vi "tvac_gui_chamber.vi"() -> ()   [LabVIEW 2017]
uses:
  Zones.ctl
  <vilib>/httpClient/ClientHandle.ctl
  <vilib>/Utility/miscctls.llb/LVPositionTypeDef.ctl
  Type_Defs/Cryo_Pump_Plots.ctl
  <vilib>/Utility/error.llb/DialogType.ctl
  <vilib>/Utility/miscctls.llb/LVBoundsTypeDef.ctl
  msg7171_linux.llb/send single message.vi
  <vilib>/httpClient/POSTBuffer.vi
  <vilib>/Utility/file.llb/Read Delimited Spreadsheet (string).vi
  <vilib>/Utility/file.llb/Write Delimited Spreadsheet (string).vi
  <vilib>/httpClient/LabVIEWHTTPClient.lvlib
panel:
  out "Taskbar Status":T1 {"Chamber" format="%#_2g"; "Cryo" format="%#_2g"; "Roughing" format="%#_2g"}
  in  "importexe":dbl
  in  "Path to PNG file":path=path "C:/Users/stefan/Documents/GitHub/TVAC/head/Labview2017/TVAC_GUI/Visualization/chamber_test.png"
  in  "Moving 1":bool
  in  "TC1to45PicRef":refnum<vi>
  in  "profilearray":dbl[][](array[numeric])
  in  "LastSetPt":i32
  in  "string":string
  in  "tprofilesheet":string[][](array[string])
  in  "Custom Graph Selector":i32
  in  "exit":bool
  in  "AlarmColor":u32(colorbox)
  in  "Alarm String":string
  in  "Plot Color":u32(colorbox)=16860
  in  "Temperature":dbl format="%#_13g"
  in  "TC Label":string
  in  "Graph ON/OFF":u32(colorbox)=4250624
  in  "index (col)":i32
  in  "index (row)":i32
  out "working array":bool[](array[boolean])
  in  "Tab Control":T2(tab)
  in  "Log/Linear Y-Axis":u16(ring) items=["Linear", "Log"]
  in  "Total Time":dbl
  in  "Set Time TC Graph":bool
  in  "Graphing Selection":u16(ring) items=["User Selection", "Graph All Thermocouples", "Clear Graph"]
  in  "Time Scale":u16(ring) items=["Minutes", "Hours", "Seconds"]
  out "Waveform Chart":waveform(dbl)[](graph)
  out "Thermocouples":T3(array[cluster])
  in  "Log/Linear Y-Axis 6":u16(ring) items=["Linear", "Log"]
  in  "Log/Linear Y-Axis 5":u16(ring) items=["Linear", "Log"]
  in  "Log/Linear Y-Axis 3":u16(ring) items=["Linear", "Log"]
  in  "Log/Linear Y-Axis 2":u16(ring) items=["Linear", "Log"]
  in  "Total Time 6":dbl
  in  "Set Time TC Graph 6":bool
  in  "Time Scale 6":u16(ring) items=["Minutes", "Hours", "Seconds"]
  in  "Total Time 5":dbl
  in  "Set Time TC Graph 5":bool
  in  "Time Scale 5":u16(ring) items=["Minutes", "Hours", "Seconds"]
  in  "Total Time 4":dbl
  in  "Set Time TC Graph 4":bool
  in  "Time Scale 4":u16(ring) items=["Minutes", "Hours", "Seconds"]
  in  "Total Time 3":dbl
  in  "Set Time TC Graph 3":bool
  in  "Time Scale 3":u16(ring) items=["Minutes", "Hours", "Seconds"]
  in  "Total Time 2":dbl
  in  "Set Time TC Graph 2":bool
  in  "Time Scale 2":u16(ring) items=["Minutes", "Hours", "Seconds"]
  in  "Log/Linear Y-Axis 1":u16(ring) items=["Linear", "Log"]
  in  "Total Time 1":dbl
  in  "Set Time TC Graph 1":bool
  in  "Time Scale 1":u16(ring) items=["Minutes", "Hours", "Seconds"]
  in  "Custom Chart 2 Selection":i32[](listbox)=[0]
  in  "Custom Chart 1 Selection":i32[](listbox)=[0]
  out "Custom Chart 1":waveform(dbl)[](graph)
  in  "Custom Chart 3 Selection":i32[](listbox)=[0]
  in  "Custom Chart 4 Selection":i32[](listbox)=[0]
  in  "Custom Chart 5 Selection":i32[](listbox)=[0]
  in  "Custom Chart 6 Selection":i32[](listbox)=[0]
  out "Custom Chart 2":waveform(dbl)[](graph)
  out "Custom Chart 3":waveform(dbl)[](graph)
  out "Custom Chart 4":waveform(dbl)[](graph)
  out "Custom Chart 5":waveform(dbl)[](graph)
  out "Custom Chart 6":waveform(dbl)[](graph)
  in  "Log/Linear Y-Axis 4":u16(ring) items=["Linear", "Log"]
  in  "Initiate Vacuum State":bool
  in  "Complete Event List":i32(listbox)
  in  "Database Logging On/Off":bool
  out "Thermal Profile Compiling Summary":string
  out "Active Profile":bool
  out "ThermalProfileStatus":string
  out "Thermal Profile":cluster{dbl, dbl, "temp":dbl[][]}(graph)
  in  "Thermal Profile Loader":T4(tab)
  in  "ZoneSetup":T5={"Number of Set points"=0.0, "Zone Selection"=[8], "Initiate Setup"=FALSE, "Thermal Profile Name"="", "Saved Database Profiles"=0, "Import CSV as a Thermal Profile"=path "", "Import Profile"=FALSE, "LoadFromDatabase"=FALSE} {"Saved Database Profiles" items=["debug4", "debug4_2", "debug5", "debug5_1", "debug5_2", "debug5_3", "debug5_4", "debug5_5", "debug5_6", "debug6_1", "oct_26_1", "oct_26_4", "oct_26_5", "oct_26_fast_1", "oct_26_fast_2", "oct_26_fast_3", "Oct_27_1", "oct_27_2", "oct_27_3", "oct_27_4", "oct_27_5", "oct_27_full_test", "testing_oct24_1", "testing_oct24_2", "testing_oct24_debug1", "testing_oct_25_1"]}
  in  "RampSoakTimes":cluster{"RampSoakTimes":dbl[][]}
  in  "Zone 1":T6={"Zone Thermocouples"=[0], "Temperature Calculation"=0, "Thermocouples Selected"="", "Temperature Goal"=[], "Max Allowable Temp"="", "Min Allowable Temp"="", "Max Temp Slope"=""} {"Temperature Calculation" items=["Average", "Minimum", "Maximum"]}
  in  "Zone 2":T6={"Zone Thermocouples"=[0], "Temperature Calculation"=0, "Thermocouples Selected"="", "Temperature Goal"=[], "Max Allowable Temp"="", "Min Allowable Temp"="", "Max Temp Slope"=""} {"Temperature Calculation" items=["Average", "Minimum", "Maximum"]}
  in  "Zone 3":T6={"Zone Thermocouples"=[0], "Temperature Calculation"=0, "Thermocouples Selected"="", "Temperature Goal"=[], "Max Allowable Temp"="", "Min Allowable Temp"="", "Max Temp Slope"=""} {"Temperature Calculation" items=["Average", "Minimum", "Maximum"]}
  in  "Zone 4":T6={"Zone Thermocouples"=[0], "Temperature Calculation"=0, "Thermocouples Selected"="", "Temperature Goal"=[], "Max Allowable Temp"="", "Min Allowable Temp"="", "Max Temp Slope"=""} {"Temperature Calculation" items=["Average", "Minimum", "Maximum"]}
  in  "Zone 5":T6={"Zone Thermocouples"=[0], "Temperature Calculation"=0, "Thermocouples Selected"="", "Temperature Goal"=[], "Max Allowable Temp"="", "Min Allowable Temp"="", "Max Temp Slope"=""} {"Temperature Calculation" items=["Average", "Minimum", "Maximum"]}
  in  "Zone 6":T6={"Zone Thermocouples"=[0], "Temperature Calculation"=0, "Thermocouples Selected"="", "Temperature Goal"=[], "Max Allowable Temp"="", "Min Allowable Temp"="", "Max Temp Slope"=""} {"Temperature Calculation" items=["Average", "Minimum", "Maximum"]}
  in  "Zone 7":T6={"Zone Thermocouples"=[0], "Temperature Calculation"=0, "Thermocouples Selected"="", "Temperature Goal"=[], "Max Allowable Temp"="", "Min Allowable Temp"="", "Max Temp Slope"=""} {"Temperature Calculation" items=["Average", "Minimum", "Maximum"]}
  in  "Zone 8":T6={"Zone Thermocouples"=[0], "Temperature Calculation"=0, "Thermocouples Selected"="", "Temperature Goal"=[], "Max Allowable Temp"="", "Min Allowable Temp"="", "Max Temp Slope"=""} {"Temperature Calculation" items=["Average", "Minimum", "Maximum"]}
  in  "Zone 9":T6={"Zone Thermocouples"=[0], "Temperature Calculation"=0, "Thermocouples Selected"="", "Temperature Goal"=[], "Max Allowable Temp"="", "Min Allowable Temp"="", "Max Temp Slope"=""} {"Temperature Calculation" items=["Average", "Minimum", "Maximum"]}
  out "Current Profile Name":string
  in  "Delete Profile":bool
  in  "New File Name":string
  in  "Rename":bool
  in  "2. Save Into Database and CSV":bool
  in  "3. Load into Memory":bool
  in  "1. Compile Profile":bool
  in  "4. Run Profile":bool
  in  "Delete From Database":u16(ring) items=["Awesome Profile", "Super Awesome Profile", "Rocket Profile", "Bannana"]
  in  "HARD STOP":bool
  in  "Pause Profile":bool
  in  "Hold Profile":bool
  out "tpStatus":T7 {"Chamber" format="%#_2g"; "Cryo" format="%#_2g"; "Roughing" format="%#_2g"}
  out "generalStatus":T7 {"Chamber" format="%#_2g"; "Cryo" format="%#_2g"; "Roughing" format="%#_2g"}
  in  "Tab Control 2":enum32{"TCs 1-75", "TCs 76-80, 96-120"}(tab)
  out "TC1to75visual":T8={"1"=TRUE, "2"=TRUE, "3"=TRUE, "4"=TRUE, "5"=TRUE, "6"=TRUE, "7"=TRUE, "8"=TRUE, "9"=TRUE, "10"=TRUE, "11"=TRUE, "12"=TRUE, "13"=TRUE, "14"=TRUE, "15"=TRUE, "16"=TRUE, "17"=TRUE, "18"=TRUE, "19"=TRUE, "20"=TRUE, "21"=TRUE, "22"=TRUE, "23"=TRUE, "24"=TRUE, "25"=TRUE, "26"=TRUE, "27"=TRUE, "28"=TRUE, "29"=TRUE, "30"=TRUE, "31"=TRUE, "32"=TRUE, "33"=TRUE, "34"=TRUE, "35"=TRUE, "36"=TRUE, "37"=TRUE, "38"=TRUE, "39"=TRUE, "40"=TRUE, "41"=TRUE, "42"=TRUE, "43"=TRUE, "44"=TRUE, "45"=TRUE, "46"=TRUE, "47"=TRUE, "48"=TRUE, "49"=TRUE, "50"=TRUE, "51"=TRUE, "52"=TRUE, "53"=TRUE, "54"=TRUE, "55"=TRUE, "56"=TRUE, "57"=TRUE, "58"=TRUE, "59"=TRUE, "60"=TRUE, "61"=TRUE, "62"=TRUE, "63"=TRUE, "64"=TRUE, "65"=TRUE, "66"=TRUE, "67"=TRUE, "68"=TRUE, "69"=TRUE, "70"=TRUE, "71"=TRUE, "72"=TRUE, "73"=TRUE, "74"=TRUE, "75"=TRUE, "new picture"=bytes[0]}
  in  "Reset All TC Positions":bool
  in  "Import UUT":bool
  out "Chamber Layout":T9 {"TC 120" format="%#_5g"; "TC 119" format="%#_5g"; "TC 118" format="%#_5g"; "TC 117" format="%#_5g"; "TC 116" format="%#_5g"; "TC 115" format="%#_5g"; "TC 114" format="%#_5g"; "TC 113" format="%#_5g"; "TC 112" format="%#_5g"; "TC 111" format="%#_5g"; "TC 110" format="%#_5g"; "TC 109" format="%#_5g"; "TC 108" format="%#_5g"; "TC 107" format="%#_5g"; "TC 106" format="%#_5g"; "TC 105" format="%#_5g"; "TC 104" format="%#_5g"; "TC 103" format="%#_5g"; "TC 102" format="%#_5g"; "TC 101" format="%#_5g"; "TC 100" format="%#_5g"; "TC 99" format="%#_5g"; "TC 98" format="%#_5g"; "TC 97" format="%#_5g"; "TC 96" format="%#_5g"; "TC 80" format="%#_5g"; "TC 79" format="%#_5g"; "TC 78" format="%#_5g"; "TC 77" format="%#_5g"; "TC 76" format="%#_5g"}
  out "Chamber Layout Picture":picture
  in  "Events":enum32{"Current", "Past"}(tab)
  in  "Clear All Events":bool
  in  "Current Events (click to clear)":i32(listbox)
  in  "Export Events":bool
  in  "Event History":i32(listbox)
  in  "Errors":enum32{"Current", "Past"}(tab)
  in  "Current Errors (click to clear)":i32(listbox)
  in  "Clear All Errors":bool
  in  "Export Errors":bool
  in  "Error History":i32(listbox)
  in  "Engineering":string
  in  "GetEvent":bool=TRUE
  in  "TCs On":bool=TRUE
  in  "Pressure On":bool=TRUE
  in  "MCC On":bool=TRUE
  in  "ZoneTemps On":bool=TRUE
  in  "Compressor On":bool
  in  "GetError":bool=TRUE
  out "flushed msgs":T10(array[cluster])
  out "system log event":string
  in  "getTvacStatus":bool=TRUE
  in  "Local Debug":bool
  in  "TVAC Labview":bool=TRUE
  # "Hidden Controls"
  # "Active Thermal Profile Commands"
  # "Create a New Thermal Profile"
  # "Import CSV as a Thermal Profile"
  # "Run Saved Database Profile"
  # "Set Pt #"
  # "Ramp Time (min)"
  # "Soak Time (min)"
  # "Set Pt #"
  # "Goal Temp (K)"
  # "Set Pt #"
  # "Goal Temp (K)"
  # "Set Pt #"
  # "Goal Temp (K)"
  # "Set Pt #"
  # "Goal Temp (K)"
  # "Set Pt #"
  # "Goal Temp (K)"
  # "Set Pt #"
  # "Goal Temp (K)"
  # "Set Pt #"
  # "Goal Temp (K)"
  # "Set Pt #"
  # "Goal Temp (K)"
  # "Set Pt #"
  # "Goal Temp (K)"
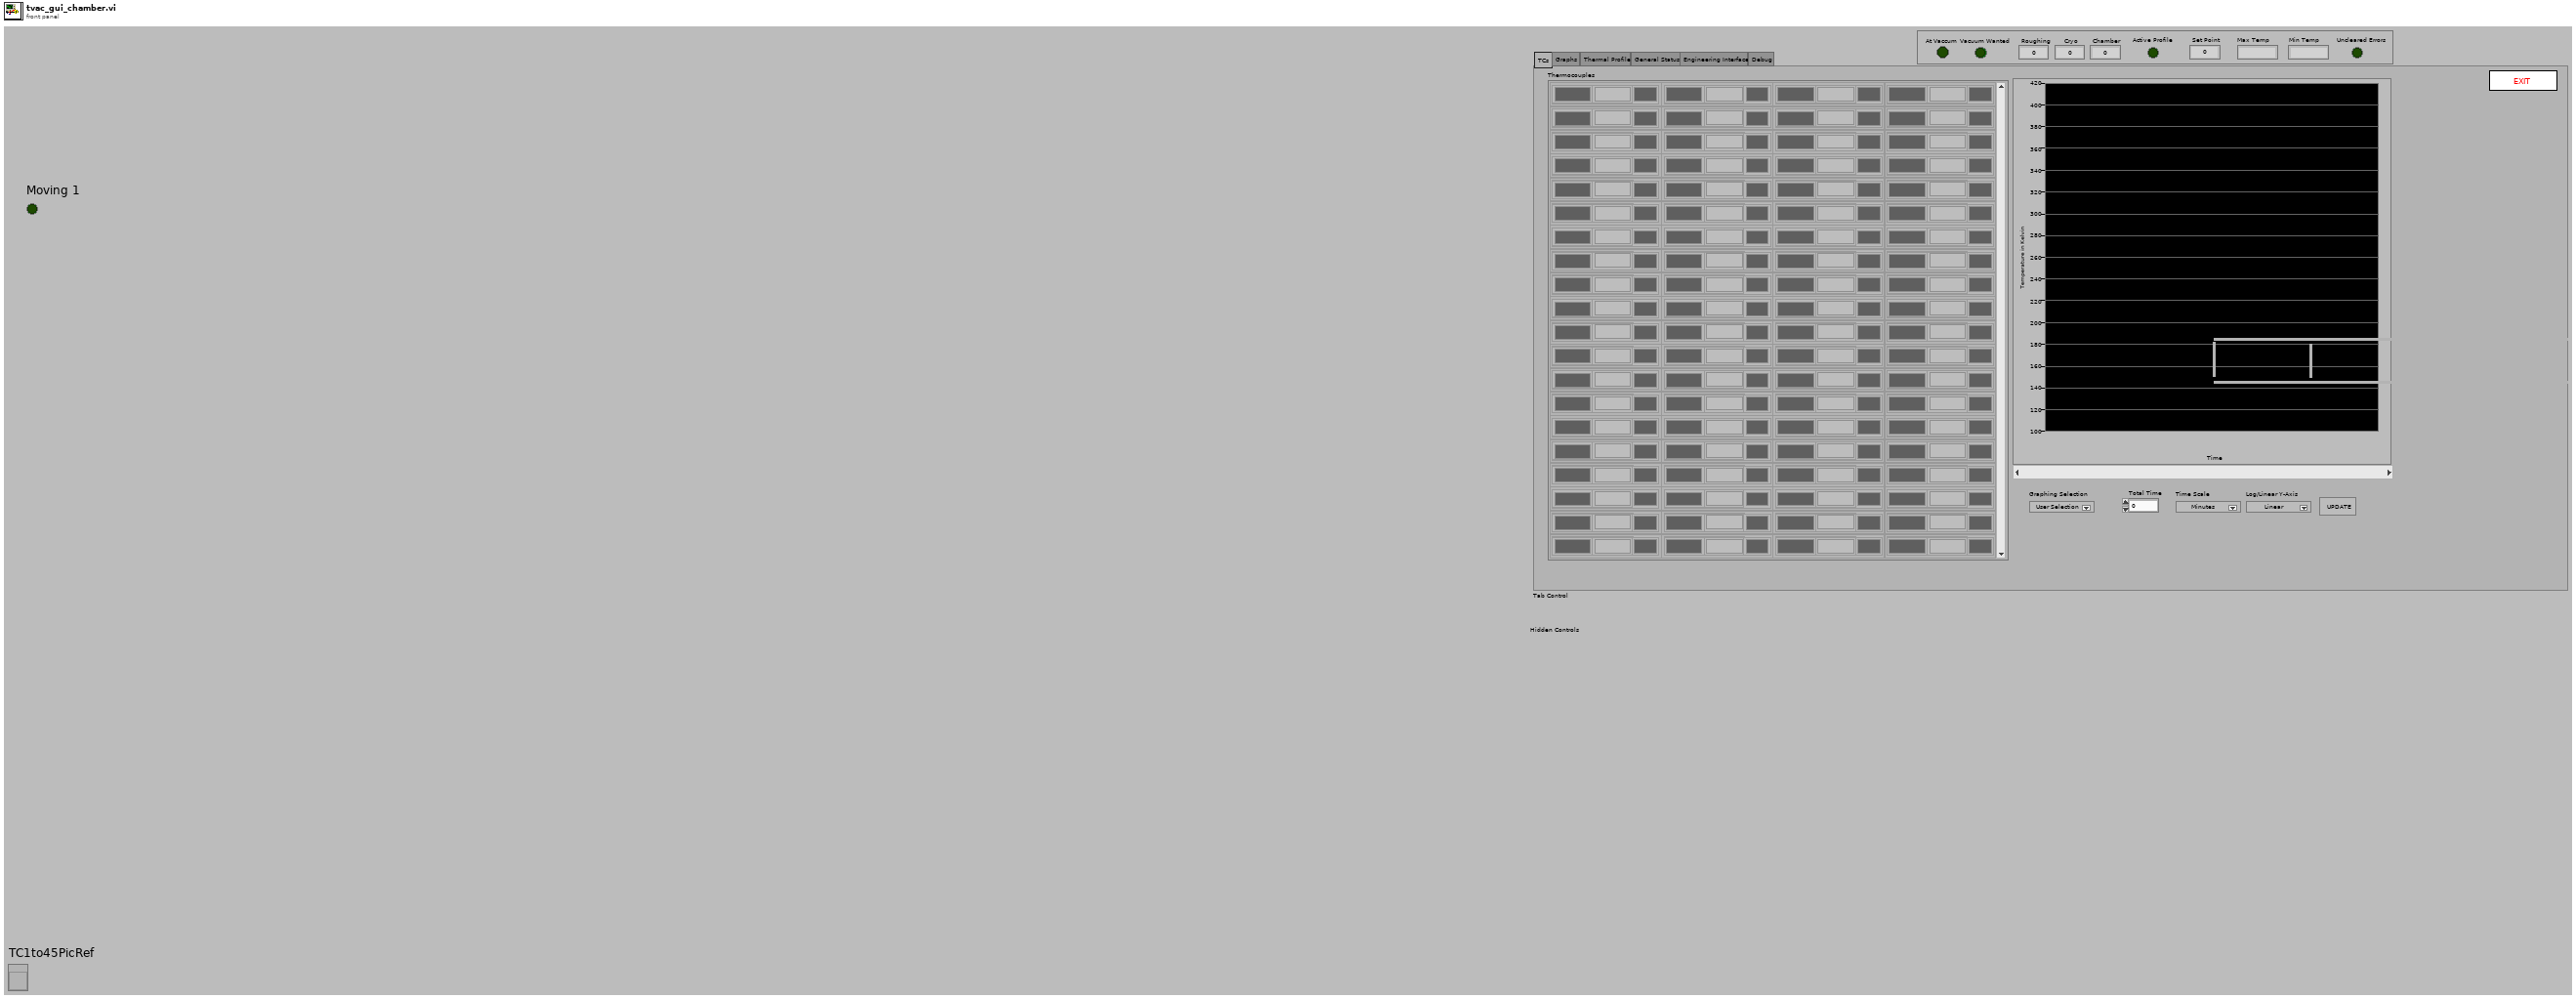
[diagram p1: front panel]
types:
  T1 = cluster{"At Vaccum":bool, "Vacuum Wanted":bool, "Roughing":dbl, "Cryo":dbl, "Chamber":dbl, "Active Profile":bool, "Set Point":dbl, "Max Temp":string, "Min Temp":string, "Uncleared Errors":bool}
  T2 = enum32{"TCs", "Graphs", "Thermal Profile", "General Status", "Engineering Interface", "Debug"}
  T3 = cluster{"TC Label":string, "Alarm Status":string, "Alarm Color":u32, "Temperature":string, "PlotColor":u32, "Graph On/Off":u32}[][]
  T4 = enum32{"Setup", "Set Point Timing", "Zone 1", "Zone 2", "Zone 3", "Zone 4", "Zone 5", "Zone 6", "Zone 7", "Zone 8", "Zone 9", "Run"}
  T5 = cluster{"Number of Set points":dbl, "Zone Selection":i32[], "Initiate Setup":bool, "Thermal Profile Name":string, "Saved Database Profiles":u16, "Import CSV as a Thermal Profile":path, "Import Profile":bool, "LoadFromDatabase":bool}
  T6 = typedef "Zones.ctl" = cluster{"Zone Thermocouples":i32[], "Temperature Calculation":u16, "Thermocouples Selected":string, "Temperature Goal":dbl[][], "Max Allowable Temp":string, "Min Allowable Temp":string, "Max Temp Slope":string}
  T7 = cluster{"Set Point":dbl, "Vacuum Wanted":bool, "Profile State":string, "Active Profile":bool, "Roughing":dbl, "Cryo":dbl, "Chamber":dbl, "Current Ramp/Soak Time":dbl, "Zone Temps":dbl[], "Remaining Ramp/Soak Time":dbl, "Max Ramp Rate":dbl, "Vacuum State":string, "At Vaccum":bool}
  T8 = cluster{"1":bool, "2":bool, "3":bool, "4":bool, "5":bool, "6":bool, "7":bool, "8":bool, "9":bool, "10":bool, "11":bool, "12":bool, "13":bool, "14":bool, "15":bool, "16":bool, "17":bool, "18":bool, "19":bool, "20":bool, "21":bool, "22":bool, "23":bool, "24":bool, "25":bool, "26":bool, "27":bool, "28":bool, "29":bool, "30":bool, "31":bool, "32":bool, "33":bool, "34":bool, "35":bool, "36":bool, "37":bool, "38":bool, "39":bool, "40":bool, "41":bool, "42":bool, "43":bool, "44":bool, "45":bool, "46":bool, "47":bool, "48":bool, "49":bool, "50":bool, "51":bool, "52":bool, "53":bool, "54":bool, "55":bool, "56":bool, "57":bool, "58":bool, "59":bool, "60":bool, "61":bool, "62":bool, "63":bool, "64":bool, "65":bool, "66":bool, "67":bool, "68":bool, "69":bool, "70":bool, "71":bool, "72":bool, "73":bool, "74":bool, "75":bool, "new picture":picture}
  T9 = cluster{"TC 76":dbl, "TC 77":dbl, "TC 78":dbl, "TC 79":dbl, "TC 80":dbl, "TC 96":dbl, "TC 97":dbl, "TC 98":dbl, "TC 99":dbl, "TC 100":dbl, "TC 101":dbl, "TC 102":dbl, "TC 103":dbl, "TC 104":dbl, "TC 105":dbl, "TC 106":dbl, "TC 107":dbl, "TC 108":dbl, "TC 109":dbl, "TC 110":dbl, "TC 111":dbl, "TC 112":dbl, "TC 113":dbl, "TC 114":dbl, "TC 115":dbl, "TC 116":dbl, "TC 117":dbl, "TC 118":dbl, "TC 119":dbl, "TC 120":dbl}
  T10 = cluster{"source":string, "event":string, "event buffer":string}[]
  T11 = typedef "LVPositionTypeDef.ctl" = cluster{"Left":i32, "Top":i32}
  T12 = cluster{"recordData":bool, "currentSetpoint":i32, "vacuumWanted":bool, "inPause":bool, "activeProfile":bool, "inRamp":bool, "inHold":bool, "CryoPressure":dbl, "ChamberPressure":dbl, "RoughingPressure":dbl, "OperationalVacuum":bool}
  T13 = cluster{"profiles":cluster{"zone":i32, "average":string, "thermocouples":i32[], "maxTemp":i32, "minTemp":i32, "maxSlope":dbl, "thermalprofiles":cluster{"thermalsetpoint":i32, "tempgoal":i32, "ramp":i32, "soakduration":i32}[]}[]}
  T14 = cluster{"thermocouple":i32, "time":dbl, "temp":dbl, "working":bool, "alarm":i32}[]
  T15 = cluster{"Cp Stage 1 Temp":dbl[], "Cp Stage 2 Temp":dbl[]}
  T16 = typedef "LabVIEWHTTPClient.lvlib/ClientHandle.ctl" = refnum<k1>
  T17 = cluster{"ZoneSetup":cluster{"Number of Set points":dbl, "Zone Selection":i32[], "Initiate Setup":bool, "Thermal Profile Name":string, "Saved Database Profiles":u16, "Import CSV as a Thermal Profile":path, "Import Profile":bool, "LoadFromDatabase":bool}, "go":bool, "Http session":T16, "URL prefex":string, "index (row)":i32, "index (col)":i32, "Graph ON/OFF":u32, "TC Label":string, "Temperature":dbl, "AlarmColor":u32, "Plot Color":u32, "Alarm String":string, "Thermocouples":cluster{"TC Label":string, "Alarm Status":string, "Alarm Color":u32, "Temperature":string, "PlotColor":u32, "Graph On/Off":u32}[][], "working array":bool[], "i":i32, "NumberTCs":i32, "Waveform Chart":waveform(dbl)[], "Custom Chart 1":waveform(dbl)[], "Pressure":dbl[], "numSensors":i32, "Database":dbl[], "PumpTemps":cluster{"Cp Stage 1 Temp":dbl[], "Cp Stage 2 Temp":dbl[]}, "Zones":dbl[], "Time":i32, "TCs":cluster{"thermocouple":i32, "time":dbl, "temp":dbl, "working":bool, "alarm":i32}[], "ZoneTemps":cluster{"ZoneTemps":dbl[]}, "Compressor":cluster{"CompressorTemp":dbl}, "ErrorArray":string[][], "PrevErrorArray":string[][], "MasterErrorArray":string[][], "tprofilesheet":string[][], "Zone 1":T6, "ZoneProfile":cluster{"profiles":cluster{"zone":i32, "average":string, "thermocouples":i32[], "maxTemp":i32, "minTemp":i32, "maxSlope":dbl, "thermalprofiles":cluster{"thermalsetpoint":i32, "tempgoal":i32, "ramp":i32, "soakduration":i32}[]}[]}, "ZonesSelected":bool[], "Zone 2":T6, "Zone 3":T6, "Zone 4":T6, "Zone 5":T6, "Zone 6":T6, "Zone 7":T6, "Zone 8":T6, "Zone 9":T6, "MasterEventArray":string[][], "PrevEventArray":string[][], "EventArray":string[][], "TC1to45PicRef":refnum<vi>, "TvacStatus":cluster{"recordData":bool, "currentSetpoint":i32, "vacuumWanted":bool, "inPause":bool, "activeProfile":bool, "inRamp":bool, "inHold":bool, "CryoPressure":dbl, "ChamberPressure":dbl, "RoughingPressure":dbl, "OperationalVacuum":bool}}
  T18 = cluster{"TC Label":string, "Alarm Status":string, "Alarm Color":u32, "Temperature":string, "PlotColor":u32, "Graph On/Off":u32}
  T19 = cluster{"time":string, "TCs":cluster{"thermocouple":i32, "time":dbl, "temp":dbl, "working":bool, "alarm":i32}[]}
  T20 = cluster{"name":string, "profiles":cluster{"zone":i32, "average":string, "thermocouples":i32[], "maxTemp":i32, "minTemp":i32, "maxSlope":i32, "thermalprofiles":cluster{"thermalsetpoint":i32, "tempgoal":i32, "ramp":i32, "soakduration":i32}[]}[]}
  T21 = enum16{"open", "replace", "create", "open or create", "replace or create", "replace or create with confirmation"}
  T22 = cluster{"zone":i32, "average":string, "thermocouples":i32[], "maxTemp":i32, "minTemp":i32, "maxSlope":dbl, "thermalprofiles":cluster{"thermalsetpoint":i32, "tempgoal":i32, "ramp":i32, "soakduration":i32}[]}
  T23 = cluster{"thermalsetpoint":i32, "tempgoal":i32, "ramp":i32, "soakduration":i32}
  T24 = cluster{"time":string[], "event":string[], "item":string[], "itemID":i32[], "details":string[], "actions":string[][]}
  T25 = enum32{"TCs", "Graphs", "Thermal Profile", "General Status"}
  T26 = cluster{"time":string[], "category":string[], "message":string[]}
  T27 = cluster{"CryoPressure":dbl, "ChamberPressure":dbl, "RoughingPressure":dbl}
  T28 = cluster{"Set Point":dbl, "Vacuum Wanted":bool, "Profile State":string, "Active Profile":bool, "Roughing":dbl, "Cryo":dbl, "Chamber":dbl, "Current Ramp/Soak Time":dbl, "Zone Temps":dbl[], "Remaining Ramp/Soak Time":dbl, "Max Ramp Rate":dbl, "Vacuum State":string, "At Vacuum":bool}
  T29 = typedef "imagedata.ctl" = cluster{"image type":i32, "image depth":i32, "image":u8[], "mask":u8[], "colors":u32[], "Rectangle":cluster{"left":i16, "top":i16, "right":i16, "bottom":i16}}
  T30 = typedef "LVPoint32TypeDef.ctl" = cluster{"Horizontal":i32, "Vertical":i32}
  T31 = typedef "LVRangeTypeDef.ctl" = cluster{"Minimum":dbl, "Maximum":dbl, "Increment":dbl, "Minor Increment":dbl, "Start":dbl}
  T32 = cluster{"zone":i32, "average":string, "thermocouples":i32[], "maxTemp":i32, "minTemp":i32, "maxSlope":dbl, "thermalprofiles":cluster{"thermalsetpoint":i32, "tempgoal":i32, "ramp":i32, "soakduration":i32}[]}[]
  T33 = typedef "LVRowAndColumnTypeDef.ctl" = cluster{"Row":i32, "Column":i32}
  T34 = cluster{"thermalsetpoint":i32, "tempgoal":i32, "ramp":i32, "soakduration":i32}[]
  T35 = cluster{"time":dbl[], "zone1":dbl[], "zone2":dbl[], "zone3":dbl[], "zone4":dbl[], "zone5":dbl[], "zone6":dbl[], "zone7":dbl[], "zone8":dbl[], "zone9":dbl[]}
  T36 = typedef "Cryo_Pump_Plots.ctl" = cluster{"Duty Cycle (0-100)":dbl, "1st stage Temp (K)":dbl, "2st stage Temp (K)":dbl, "Helium Return Pressure (psig)":u32, "Helium Discharge Temp (C)":u32, "Water Inlet Temp (C)":u32, "Water Outlet Temp (C)":u32}
  T37 = typedef "DialogType.ctl" = u16
  T38 = cluster{"thermocouple":i32, "time":dbl, "temp":dbl, "working":bool, "alarm":i32}
  T39 = cluster{"[0]":dbl, "[1]":dbl, "[2]":dbl, "[3]":dbl, "[4]":dbl, "[5]":dbl, "[6]":dbl, "[7]":dbl, "[8]":dbl, "[9]":dbl, "[10]":dbl, "[11]":dbl, "[12]":dbl, "[13]":dbl, "[14]":dbl, "[15]":dbl, "[16]":dbl, "[17]":dbl, "[18]":dbl, "[19]":dbl, "[20]":dbl, "[21]":dbl, "[22]":dbl, "[23]":dbl, "[24]":dbl, "[25]":dbl, "[26]":dbl, "[27]":dbl, "[28]":dbl, "[29]":dbl}
  T40 = typedef "LVBoundsTypeDef.ctl" = cluster{"Width":u32, "Height":u32}
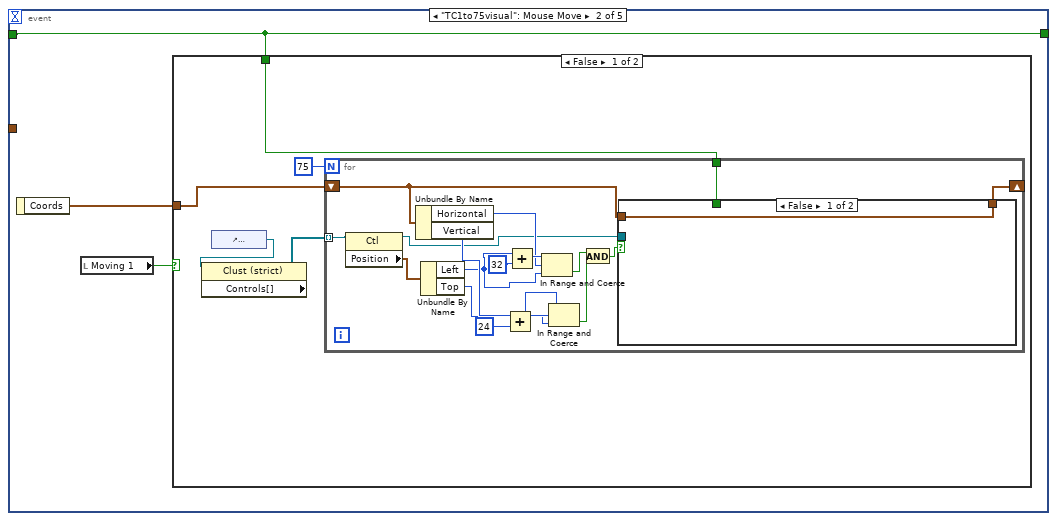
[diagram p3: hidden frame]
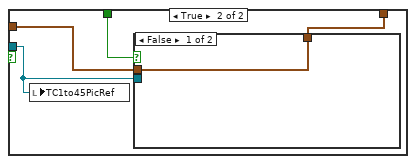
[diagram p4: hidden frame]
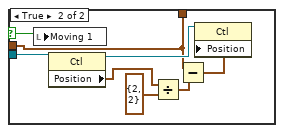
[diagram p5: hidden frame]
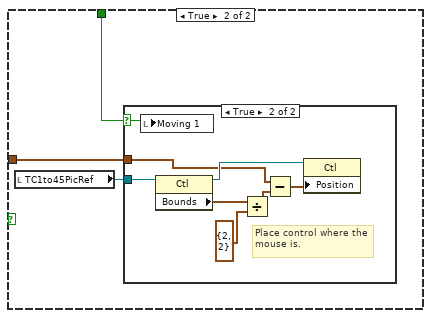
[diagram p6: hidden frame]
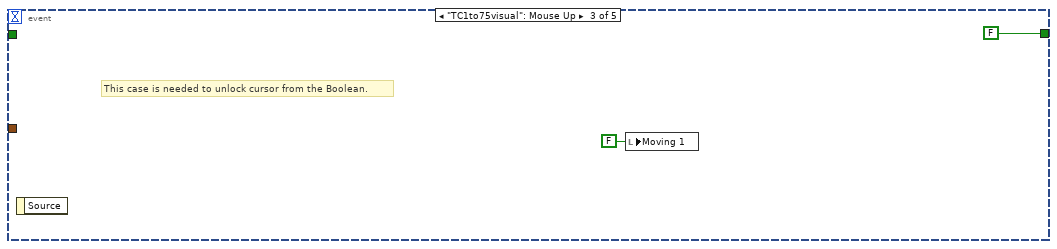
[diagram p8: hidden frame]
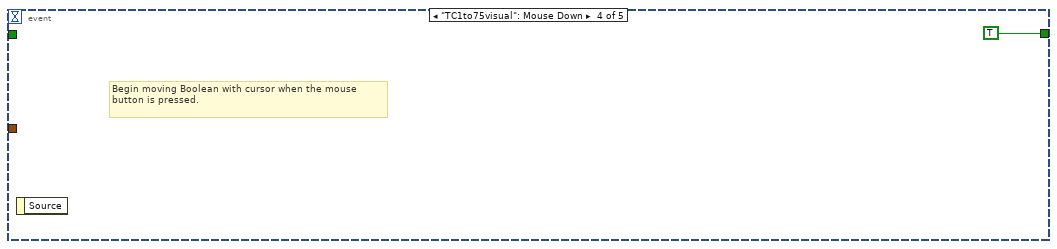
[diagram p9: hidden frame]
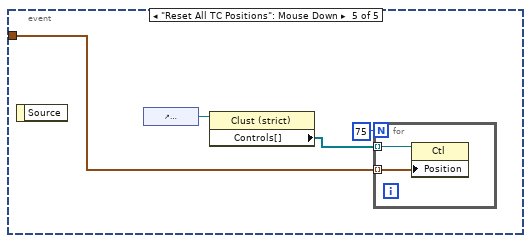
[diagram p10: hidden frame]
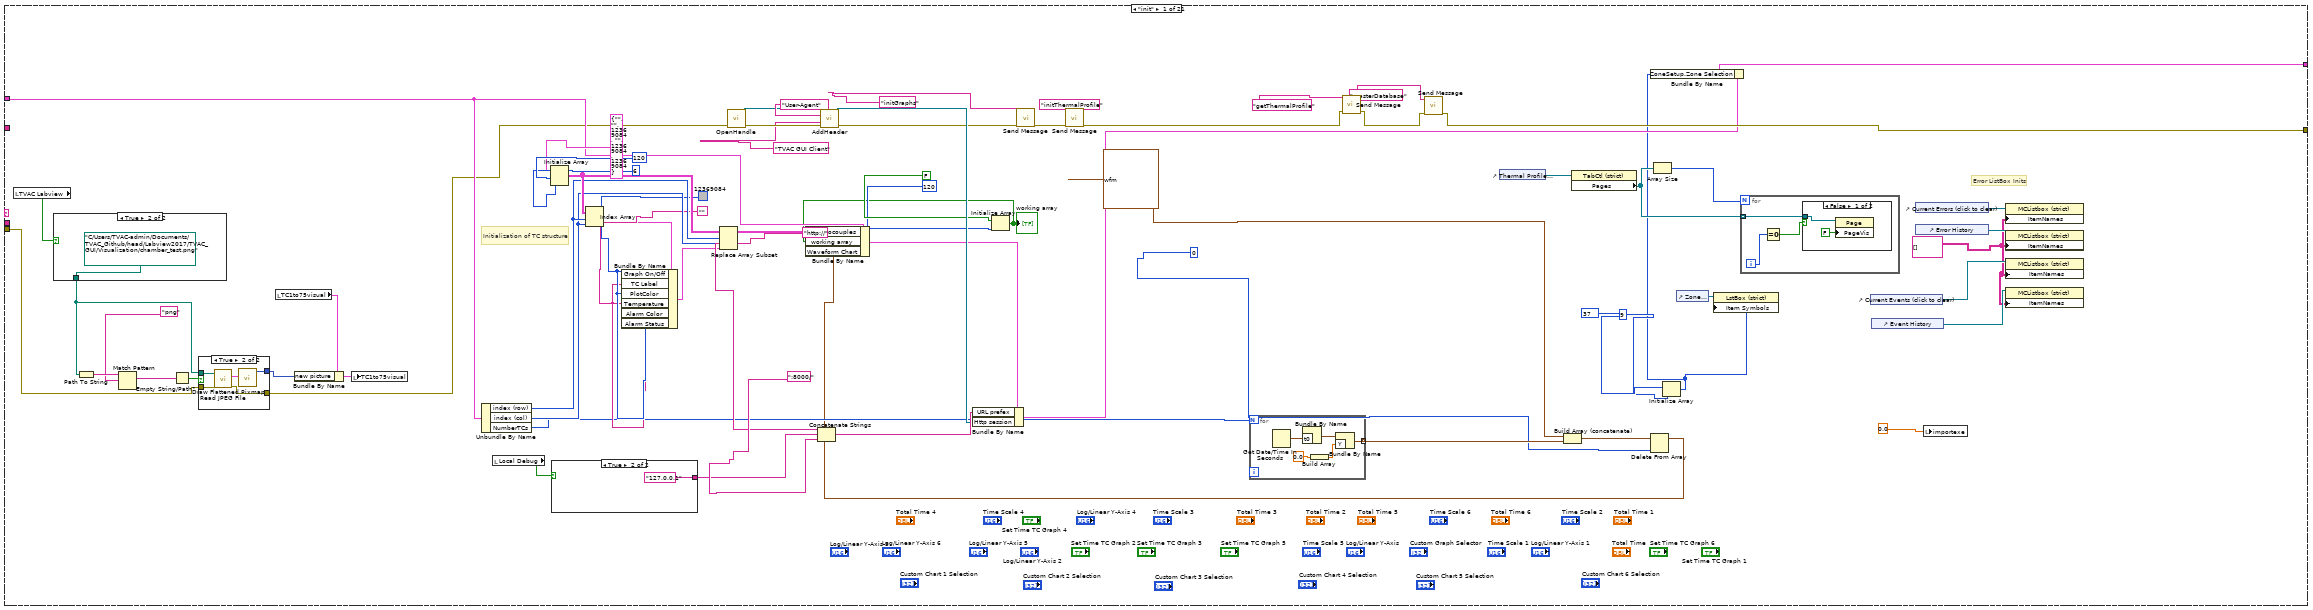
[diagram p11: hidden frame]
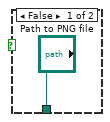
[diagram p12: hidden frame]
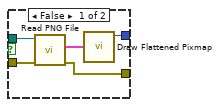
[diagram p13: hidden frame]
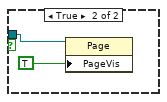
[diagram p14: hidden frame]
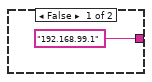
[diagram p15: hidden frame]
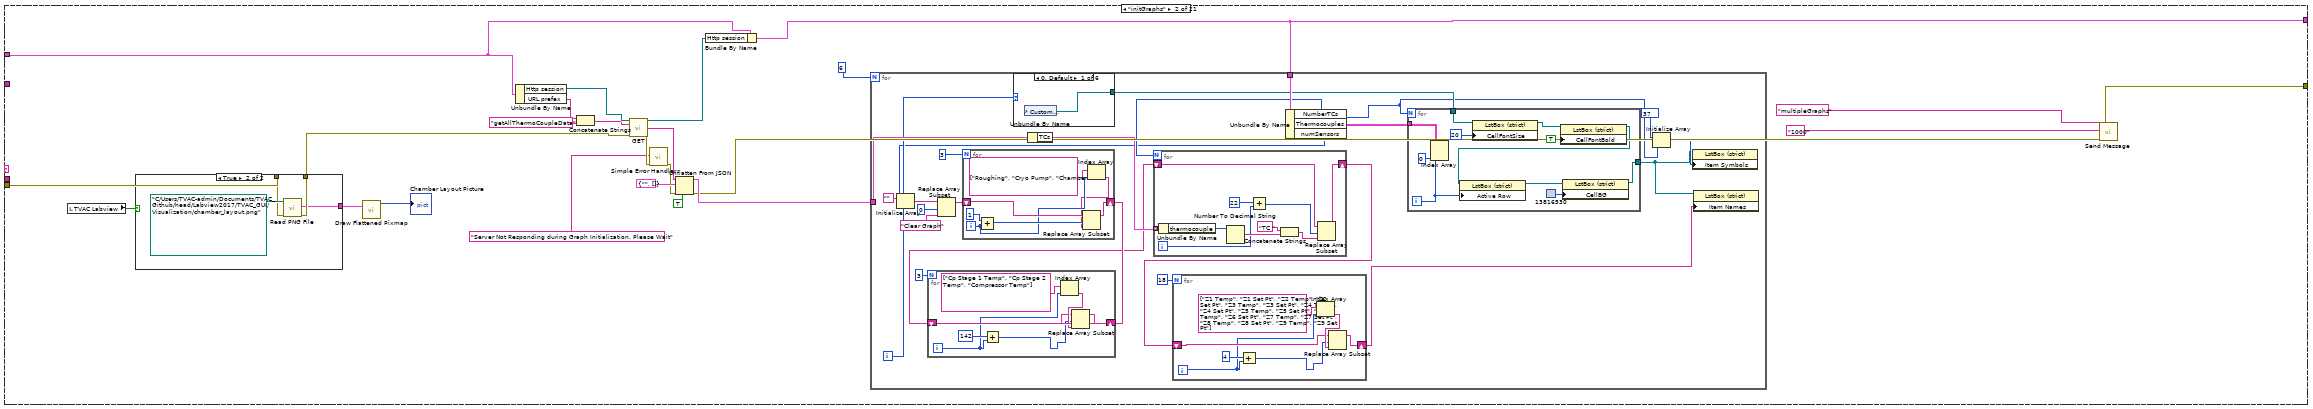
[diagram p16: hidden frame]
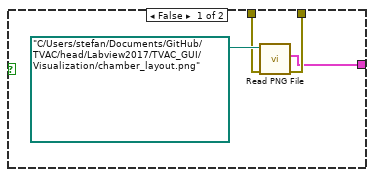
[diagram p17: hidden frame]
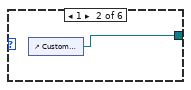
[diagram p18: hidden frame]
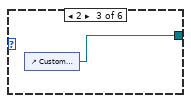
[diagram p19: hidden frame]
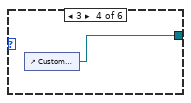
[diagram p20: hidden frame]
diagram:
  w5 = T12 {"recordData"=FALSE, "currentSetpoint"=0, "vacuumWanted"=FALSE, "inPause"=FALSE, "activeProfile"=FALSE, "inRamp"=FALSE, "inHold"=FALSE, "CryoPressure"=0.0, "ChamberPressure"=0.0, "RoughingPressure"=0.0, "OperationalVacuum"=FALSE}  # TvacStatus
  w9 = string[][] []  # MasterEventArray
  w7 = string[][] []  # EventArray
  w8 = string[][] []  # PrevEventArray
  w10 = string[][] []  # MasterErrorArray
  w14 = T13 {"profiles"=[]}  # ZoneProfile
  w23 = bool[] [FALSE, FALSE, FALSE, FALSE, FALSE, FALSE, FALSE, FALSE, FALSE]  # ZonesSelected
  w27 = string[][] []  # PrevErrorArray
  w28 = string[][] []  # ErrorArray
  w31 = cluster{"ZoneTemps":dbl[]} {"ZoneTemps"=[]}  # ZoneTemps
  w34 = dbl[] [24.54828257301887, 25.0, 20.035959453954195, 26.0, 28.926820041278148, 27.0, 21.321976066931608, 28.0, 29.197600688359813, 29.0, 29.117373424110085, 30.0, 21.092914485312942, 31.0, 27.791581465649088, 32.0, 24.70861457288988, 33.0]  # Zones
  w35 = T15 {"Cp Stage 1 Temp"=[0.0], "Cp Stage 2 Temp"=[0.0]}  # PumpTemps
  w36 = dbl[] [0.0, 1000.5841582194602, 1000.5841582194602, 1000.5841582194602, 0.6389895835935778, 0.7578061575842531, 1.153531014677555, 1.4572061556343079, 1.0192558642672256, 0.9245021790184325, 0.34311035179988925, 1.1970333160202968, 1.066989851322369, 0.5926593131154867, 0.7219240511326698, 1.0529790116491695, 1.4485694746891444, 0.9139060201605569, 0.7997359753068659, 0.6568795179977746, 0.8470104541419833, 1.0272585161866683, 0.6577301535824354, 0.645139941938139, 1.5235316442408067, 0.5128651184775285, 1.6421980587090137, 1.3961508335147417, 1.1242639015795428, 1.5954313466624428, 1.1919135255187876, 1.2615004458206727, 1.1320092264321664, 1.922759836270222, 1.1315561200367314, 1.4924621723754858, 0.6988771274186227, 1.069709701591943, 0.9920698240997152, 0.5395549253287656, 0.42891479657680576, 1.2794224940227927, 0.2687949632437338, 0.16127136772755854, 1.0174597006256374, 1.2079238230365172, 0.9745554383837218, 1.5348516925460962, 0.9488878852839246, 1.6634477658652282, 1.1924291951744272, 1.2231949298067308, 1.2223766746774598, 1.30664154589907, 1.2872878364107239, 0.5274250065177812, 0.7905999067114673, 1.2748974665085449, 1.216972941585413, 0.959115576325391, 0.5743502840762814, 0.8219540421676025, 0.613053899308251, 1.3785560870413707, 1.034117232127813, 1.1237698659753859, 1.4495548642149667, 0.6967905980938514, 0.6224497255665377, 1.6551326273040576, 1.2103048396824558, 0.6078721016951973, 1.3790669246280296, 0.5454332940871525, 1.5318777012492035, 1.2496539590411258, 0.9145395304446965, 1.3855381787793546, 1.0857600342029163, 1.3185833631438346, 0.9769688683142593, 1.026663691242448, 0.6744610422623843, 1.1965175398567691, 0.4847084945450119, 0.6435799980029115, 0.8079659363810663, 0.9130053929540112, 0.5271098423006861, 0.8088111736464799, 1.1455315536576556, 1.139809531926708, 1.5840192673434794, 1.0296748968089129, 1.7370669751200136, 1.3715484550405317, 0.3362063953932494, 1.0385868418202253, 1.4947740276021626, 1.0393600693910505, 0.8870410800672984, 1.2470388696569872, 0.9846724980375481, 0.9952471377109308, 1.0807485178906029, 1.1016630607035562, 1.3301039036808464, 0.8856852816151205, 0.4719509873120426, 0.5191430277856135, 0.12135113366044793, 0.4230478635224125, 1.1140562049976255, 1.5484968368781251, 1.1999891199114734, 1.8721302183420216, 1.071489235222563, 0.6260864330445979, 1.0305668002030492, 1.0223711899566386, 0.7842533472819472, 1.7301290335750898, 1.318694748426881, 0.6978662965493679]  # Database
  w38 = dbl[] [0.0, 0.0, 0.0]  # Pressure
  w57 = ""  # URL prefex
  w58 = T16 refnum  # Http session
  w59 = TRUE  # go
  n1 = call "Register Module.vi"() -> ("error out"=w55:errorcluster)  [unwired: 10 in, 1 out]
  n2 = call-poly "Send Message.vi"("error in (no error)"=w55, "event"="init") -> ("error out"=w54:errorcluster)  [unwired: 9 in]
  n3 = local read "Waveform Chart"() -> (w41:waveform(dbl)[])
  n4 = local read "Thermocouples"() -> (w40:T3)
  n5 = local read "Custom Chart 1"() -> (w39:waveform(dbl)[])
  n6 = Bundle("ZoneSetup"="ZoneSetup", "go"=w59, "Http session"=w58, "URL prefex"=w57, "index (row)"="index (row)", "index (col)"="index (col)", "Graph ON/OFF"="Graph ON/OFF", "TC Label"="TC Label", "Temperature"="Temperature", "AlarmColor"="AlarmColor", "Plot Color"="Plot Color", "Alarm String"="Alarm String", "Thermocouples"=w40, "working array"=bool[] [TRUE, TRUE, TRUE, TRUE, TRUE, TRUE, TRUE, TRUE, TRUE, TRUE, TRUE, TRUE, TRUE, TRUE, TRUE, TRUE, TRUE, TRUE, TRUE, TRUE, TRUE, TRUE, TRUE, TRUE, TRUE, TRUE, TRUE, TRUE, TRUE, TRUE, TRUE, TRUE, TRUE, TRUE, TRUE, TRUE, TRUE, TRUE, TRUE, TRUE, TRUE, TRUE, TRUE, TRUE, TRUE, TRUE, TRUE, TRUE, TRUE, TRUE, TRUE, TRUE, TRUE, TRUE, TRUE, TRUE, TRUE, TRUE, TRUE, TRUE, TRUE, TRUE, TRUE, TRUE, TRUE, TRUE, TRUE, TRUE, TRUE, TRUE, TRUE, TRUE, TRUE, TRUE, TRUE, TRUE, TRUE, TRUE, TRUE, TRUE, TRUE, TRUE, TRUE, TRUE, TRUE, TRUE, TRUE, TRUE, TRUE, TRUE, TRUE, TRUE, TRUE, TRUE, TRUE, TRUE, TRUE, TRUE, TRUE, TRUE, TRUE, TRUE, TRUE, TRUE, TRUE, TRUE, TRUE, TRUE, TRUE, TRUE, TRUE, TRUE, TRUE, TRUE, TRUE, TRUE, TRUE, TRUE, TRUE, TRUE], "i"=0, "NumberTCs"=120, "Waveform Chart"=w41, "Custom Chart 1"=w39, "Pressure"=w38, "numSensors"=145, "Database"=w36, "PumpTemps"=w35, "Zones"=w34, "Time"=0, "TCs"=T14 [], "ZoneTemps"=w31, "Compressor"=cluster{"CompressorTemp":dbl} {"CompressorTemp"=0.0}, "ErrorArray"=w28, "PrevErrorArray"=w27, "MasterErrorArray"=w10, "tprofilesheet"="tprofilesheet", "Zone 1"="Zone 1", "ZoneProfile"=w14, "ZonesSelected"=w23, "Zone 2"="Zone 2", "Zone 3"="Zone 3", "Zone 4"="Zone 4", "Zone 5"="Zone 5", "Zone 6"="Zone 6", "Zone 7"="Zone 7", "Zone 8"="Zone 8", "Zone 9"="Zone 9", "MasterEventArray"=w9, "PrevEventArray"=w8, "EventArray"=w7, "TC1to45PicRef"="TC1to45PicRef", "TvacStatus"=w5) -> (w45:T17)  [unwired: 1 in]
  n7 = invoke on="exit" class="Bool (strict)" method="Reinit To Default"() -> ()  [unwired: 3 in, 3 out]
  n8 = while {
    shift-left: w45 -> [w66]
    shift-right: [w64] -> _
    shift-right: [w65] -> w13
    shift-left: w54 -> [w70]
    stop <- w63 continue-if-true
    n9 = call "Get Message.vi"("error in (no error)"=w70) -> ("error out"=w69:errorcluster, "event buffer"=w61:string, "event"=w68:string, "source"=w67:string)  [unwired: 7 in]
    n10 = case shown="\"receiveCryoPump_plots\"" w68 {
      selector: w68 -> [_ _ _ _ _ _ _ _ _ _ _ _ _ _ _ _ _ _ _ _ w3925]
      tunnel: [w88 w170 w271 w377 w2380 w2704 w3217 w3332 w3414 w3420 w3434 w3457 w3552 w3614 w3626 w3674 w3740 w3753 w3773 w3923 w3927] -> w64
      tunnel: w66 -> [w113 w171 w272 w379 w2431 w2695 w3231 w3337 w3413 w3420 w3433 w3451 w3546 w3615 w3631 w3699 w3739 w3754 w3773 w3919 w3927]
      tunnel: w61 -> [_ _ _ _ w2393 _ _ _ w3411 w3418 w3426 w3458 w3553 w3606 w3630 w3704 w3737 _ w3774 _ _]
      tunnel: w69 -> [w75 w176 w280 w381 w2376 w2703 w3233 w3327 w3412 w3421 w3427 w3455 w3550 w3607 w3629 w3703 w3738 w3759 _ w3922 w3926]
      tunnel: [w98 w179 w277 w380 w2409 w2701 w3233 w3327 w3412 w3421 w3427 w3455 w3550 w3607 w3629 w3703 w3738 w3759 _ w3921 w3924] -> w60
      tunnel: w67 -> [_ _ _ _ _ _ _ _ _ _ _ _ _ _ _ _ _ _ _ _ _]
      frame "init" {
        w83 = string[][] [] ("Item Names")
        w118 = ""
        w119 = u32 12369084 ("PlotColor")
        # "Error ListBox Inits"
        # "Initialization of TC structure"
        n11 = local read "TVAC Labview"() -> (w71:bool)
        n12 = case shown="True" w71 {
          tunnel: ["Path to PNG file" path "C:/Users/TVAC-admin/Documents/TVAC_Github/head/Labview2017/TVAC_GUI/Visualization/chamber_test.png" ("Path to PNG file")] -> w76
          frame False {
          }
          frame True {
          }
        }
        n13 = Path To String(path=w76) -> (string=w80:string)
        n14 = Match Pattern(string=w80, regular expression="png") -> (match substring=w78:string)  [unwired: 1 in, 3 out]
        n15 = Empty String/Path?(string/path=w78) -> (empty?=w77:bool)
        n16 = case shown="True" w77 {
          tunnel: [w144 w149] -> w73
          tunnel: w75 -> [w143 w146]
          tunnel: [w142 w147] -> w74
          tunnel: w76 -> [w140 w145]
          frame False {
            n17 = call <vilib>:"Read PNG File.vi"("error in (no error)"=w143, "path to PNG file"=w140) -> ("error out"=w142:errorcluster, "image data"=w141:T29)  [unwired: 7 in, 1 out]
            n18 = call <vilib>:"Draw Flattened Pixmap.vi"("image data"=w141) -> ("new picture"=w144:picture)  [unwired: 8 in]
          }
          frame True {
            n19 = call <vilib>:"Read JPEG File.vi"("error in (no error)"=w146, "path to JPEG file"=w145) -> ("error out"=w147:errorcluster, "image data"=w148:T29)  [unwired: 7 in, 1 out]
            n20 = call <vilib>:"Draw Flattened Pixmap.vi"("image data"=w148) -> ("new picture"=w149:picture)  [unwired: 8 in]
          }
        }
        n21 = local read "TC1to75visual"() -> (w81:T8)
        n22 = Bundle By Name(cluster=w81, "new picture"=w73) -> (w82:T8)
        n23 = local write "TC1to75visual"(w82) -> ()
        n24 = Unbundle By Name(w113) -> ("index (row)"=w121:i32, "index (col)"=w120:i32, "NumberTCs"=w110:i32)
        n25 = local read "Local Debug"() -> (w126:bool)
        n26 = Initialize Array(T18 {"TC Label"="", "Alarm Status"="", "Alarm Color"=12369084, "Temperature"="", "PlotColor"=12369084, "Graph On/Off"=12369084}, 120 ("dimension size"), 6 ("dimension size")) -> (w122:T3)
        n27 = case shown="True" w126 {
          tunnel: ["192.168.99.1" ("Address") "127.0.0.1" ("Address")] -> w127
          frame False {
          }
          frame True {
          }
        }
        n28 = Index Array(array=w122, index (row)=w121, index (col)=w120) -> (element=w117:T18)
        n29 = Bundle By Name(cluster=w117, "Graph On/Off"=w119, "TC Label"=w118, "PlotColor"=w119, "Temperature"=w118, "Alarm Color"=w119, "Alarm Status"=w118) -> (w116:T18)
        n30 = Replace Array Subset(array=w122, new element=w116, index (row)=w121, index (col)=w120) -> (w104:T3)
        n31 = call <vilib>:"OpenHandle.vi"("error in (no error)"=w74) -> ("client handle out"=w134:T16, "error out"=w137:errorcluster)  [unwired: 13 in]
        n32 = Concatenate Strings("http://" ("url"), w127, ":8000/" ("url")) -> (w131:string)
        n33 = call <vilib>:"AddHeader.vi"("client handle"=w134, "header"="User-Agent", "value"="TVAC GUI Client", "error in (no error)"=w137) -> ("client handle out"=w130:T16, "error out"=w129:errorcluster)  [unwired: 10 in]
        n34 = Initialize Array(FALSE ("Boolean"), 120 ("dimension size")) -> (w111:bool[])
        "working array" <- w111
        n35 = call-poly "Send Message.vi"("error in (no error)"=w129, "event"="initGraphs") -> ("error out"=w103:errorcluster)  [unwired: 9 in]
        n36 = call-poly "Send Message.vi"("error in (no error)"=w103, "event"="initThermalProfile") -> ("error out"=w101:errorcluster)  [unwired: 9 in]
        n37 = for {
          N: w110 -> [_]
          tunnel: [w157] -> w108 mode=indexing
          n38 = Get Date/Time In Seconds() -> (seconds since 1Jan1904=w161:timestamp)
          n39 = Bundle By Name("t0"=w161) -> (w158:waveform(dbl))  [unwired: 1 in]
          n40 = Build Array(0.0) -> (w160:dbl[])
          n41 = Bundle By Name(cluster=w158, "Y"=w160) -> (w157:waveform(dbl))
        }
        n42 = call-poly "Send Message.vi"("error in (no error)"=w101, "event"="getThermalProfile") -> ("error out"=w99:errorcluster)  [unwired: 9 in]
        n43 = call-poly "Send Message.vi"("error in (no error)"=w99, "event"="masterDatabase") -> ("error out"=w98:errorcluster)  [unwired: 9 in]
        n44 = control-ref of="Thermal Profile Loader"() -> (w96:refnum<vi>)
        n45 = Build Array (concatenate)(waveform(dbl) {"t0"=timestamp(0 s since 1904-01-01), "dt"=1.0, "Y"=[0.0]} ("element"), w108) -> (w109:waveform(dbl)[])
        n46 = property on="Property Node" class="TabCtl (strict)"(reference=w96) -> ("Pages"=w94:refnum<vi>[])  [unwired: 1 in, 2 out]
        n47 = Delete From Array(array=w109, index=0) -> (array with subset deleted=w107:waveform(dbl)[])  [unwired: 1 in, 1 out]
        n48 = Bundle By Name(cluster=w113, "Thermocouples"=w104, "working array"=w111, "Waveform Chart"=w107) -> (w112:T17)
        n49 = Bundle By Name(cluster=w112, "URL prefex"=w131, "Http session"=w130) -> (w91:T17)
        n50 = Array Size(array=w94) -> (size(s)=w95:i32)
        n51 = Initialize Array(37, 9 ("dimension size")) -> (w89:i32[])
        n52 = Bundle By Name(cluster=w91, "ZoneSetup.Zone Selection"=w89) -> (w88:T17)
        n53 = control-ref of="Zone Selection"() -> (w90:refnum<vi>)
        n54 = property class="LstBox (strict)"(reference=w90, "Item Symbols"=w89) -> ()  [unwired: 1 in, 2 out]
        n55 = for {
          N: w95 -> [_]
          tunnel: w94 -> [w150] mode=indexing
          i -> [w152]
          n56 = Equal To 0?(x=w152) -> (x = 0?=w151:bool)
          n57 = case shown="False" w151 {
            tunnel: w150 -> [w153 w155]
            frame False {
              n58 = property on="Property Node" class="Page"(reference=w153, "PageVis"=FALSE ("Page Visible")) -> ()  [unwired: 1 in, 2 out]
            }
            frame True {
              n59 = property on="Property Node" class="Page"(reference=w155, "PageVis"=TRUE ("Page Selector Visible")) -> ()  [unwired: 1 in, 2 out]
            }
          }
        }
        n60 = control-ref of="Current Events (click to clear)"() -> (w85:refnum<vi>)
        n61 = control-ref of="Event History"() -> (w84:refnum<vi>)
        n62 = control-ref of="Current Errors (click to clear)"() -> (w87:refnum<vi>)
        n63 = control-ref of="Error History"() -> (w86:refnum<vi>)
        n64 = local write "importexe"(0.0 ("importexe")) -> ()
        n65 = property on="Property Node" class="MCListbox (strict)"(reference=w87, "ItemNames"=w83) -> ()  [unwired: 1 in, 2 out]
        n66 = property on="Property Node" class="MCListbox (strict)"(reference=w86, "ItemNames"=w83) -> ()  [unwired: 1 in, 2 out]
        n67 = property on="Property Node" class="MCListbox (strict)"(reference=w85, "ItemNames"=w83) -> ()  [unwired: 1 in, 2 out]
        n68 = property on="Property Node" class="MCListbox (strict)"(reference=w84, "ItemNames"=w83) -> ()  [unwired: 1 in, 2 out]
      }
      frame "initGraphs" {
        n69 = local read "TVAC Labview"() -> (w177:bool)
        n70 = case shown="True" w177 {
          tunnel: w176 -> [w190 w194]
          tunnel: [w189 w193] -> w175
          tunnel: [w188 w192] -> w174
          frame False {
            n71 = call <vilib>:"Read PNG File.vi"("error in (no error)"=w190, "path to PNG file"=path "C:/Users/stefan/Documents/GitHub/TVAC/head/Labview2017/TVAC_GUI/Visualization/chamber_layout.png") -> ("error out"=w189:errorcluster, "image data"=w188:T29)  [unwired: 7 in, 1 out]
          }
          frame True {
            n72 = call <vilib>:"Read PNG File.vi"("error in (no error)"=w194, "path to PNG file"=path "C:/Users/TVAC-admin/Documents/TVAC_Github/head/Labview2017/TVAC_GUI/Visualization/chamber_layout.png") -> ("error out"=w193:errorcluster, "image data"=w192:T29)  [unwired: 7 in, 1 out]
          }
        }
        n73 = call <vilib>:"Draw Flattened Pixmap.vi"("image data"=w174) -> ("new picture"=→"Chamber Layout Picture":picture)  [unwired: 8 in]
        n74 = Unbundle By Name(w171) -> ("Http session"=w187:T16, "URL prefex"=w185:string)
        n75 = Concatenate Strings(w185, "getAllThermoCoupleData" ("url")) -> (w186:string)
        n76 = call <vilib>:"GET.vi"("client handle"=w187, "url"=w186, "error in (no error)"=w175) -> ("client handle out"=w169:T16, "body"=w183:string, "error out"=w166:errorcluster)  [unwired: 9 in, 1 out]
        n77 = call <vilib>:"Simple Error Handler.vi"("error source (\" \")"="Server Not Responding during Graph Initialization. Please Wait", "error in (no error)"=w166) -> ("error out"=w165:errorcluster)  [unwired: 3 in, 4 out]
        n78 = Unflatten From JSON(JSON string=w183, type and defaults=T19 {"time"="", "TCs"=[]} ("Cluster"), default null elements? (F)=TRUE, error in (no error)=w165) -> (value=w182:T19, error out=w167:errorcluster)  [unwired: 3 in]
        n79 = Bundle By Name(cluster=w171, "Http session"=w169) -> (w170:T17)
        n80 = for {
          N: 6 ("Numeric") -> [_]
          tunnel: w182 -> [w217]
          tunnel: w170 -> [w216]
          i -> [w199]
          n81 = case shown="0, Default" w199 {
            tunnel: [w219 w220 w221 w222 w223 w224] -> w200
            frame 0, Default {
              n82 = control-ref of="Custom Chart 1 Selection"() -> (w219:refnum<vi>)
            }
            frame 1 {
              n83 = control-ref of="Custom Chart 2 Selection"() -> (w220:refnum<vi>)
            }
            frame 2 {
              n84 = control-ref of="Custom Chart 3 Selection"() -> (w221:refnum<vi>)
            }
            frame 3 {
              n85 = control-ref of="Custom Chart 4 Selection"() -> (w222:refnum<vi>)
            }
            frame 4 {
              n86 = control-ref of="Custom Chart 5 Selection"() -> (w223:refnum<vi>)
            }
            frame 5 {
              n87 = control-ref of="Custom Chart 6 Selection"() -> (w224:refnum<vi>)
            }
          }
          n88 = Unbundle By Name(w217) -> ("TCs"=w213:T14)
          n89 = Unbundle By Name(w216) -> ("NumberTCs"=w211:i32, "Thermocouples"=w218:T3, "numSensors"=w197:i32)
          n90 = Initialize Array("", w197) -> (w209:string[])
          n91 = Replace Array Subset(array=w209, new element="Clear Graph" ("new element/subarray"), index=0) -> (w206:string[])
          n92 = for {
            N: 3 -> [_]
            shift-right: [w244] -> w204
            shift-left: w206 -> [w245]
            i -> [w240]
            n93 = Add(x=1 ("index"), y=w240) -> (x+y=w242:i32)
            n94 = Index Array(array=string[] ["Roughing", "Cryo Pump", "Chamber"], index=w240) -> (element=w239:string)
            n95 = Replace Array Subset(array=w245, new element=w239, index=w242) -> (w244:string[])
          }
          n96 = for {
            N: 3 -> [_]
            shift-right: [w235] -> w203
            shift-left: w204 -> [w236]
            i -> [w232]
            n97 = Add(x=142 ("index"), y=w232) -> (x+y=w233:i32)
            n98 = Index Array(array=string[] ["Cp Stage 1 Temp", "Cp Stage 2 Temp", "Compressor Temp"], index=w232) -> (element=w237:string)
            n99 = Replace Array Subset(array=w236, new element=w237, index=w233) -> (w235:string[])
          }
          n100 = for {
            N: w211 -> [_]
            tunnel: w213 -> [w252] mode=indexing
            shift-right: [w246] -> w196
            shift-left: w203 -> [w248]
            i -> [w250]
            n101 = Unbundle By Name(w252) -> ("thermocouple"=w253:i32)
            n102 = Number To Decimal String(number=w253) -> (decimal integer string=w255:string)  [unwired: 1 in]
            n103 = Add(x=22 ("index"), y=w250) -> (x+y=w249:i32)
            n104 = Concatenate Strings("TC " ("string"), w255) -> (w247:string)
            n105 = Replace Array Subset(array=w248, new element=w247, index=w249) -> (w246:string[])
          }
          n106 = for {
            N: 18 -> [_]
            shift-right: [w225] -> w202
            shift-left: w196 -> [w227]
            i -> [w226]
            n107 = Add(x=4 ("index"), y=w226) -> (x+y=w228:i32)
            n108 = Index Array(array=string[] ["Z1 Temp", "Z1 Set Pt", "Z2 Temp", "Z2 Set Pt", "Z3 Temp", "Z3 Set Pt", "Z4 Temp", "Z4 Set Pt", "Z5 Temp", "Z5 Set Pt", "Z6 Temp", "Z6 Set Pt", "Z7 Temp", "Z7 Set Pt", "Z8 Temp", "Z8 Set Pt", "Z9 Temp", "Z9 Set Pt"], index=w226) -> (element=w230:string)
            n109 = Replace Array Subset(array=w227, new element=w230, index=w228) -> (w225:string[])
          }
          n110 = for {
            N: w197 -> [_]
            tunnel: w218 -> [w266]
            tunnel: w200 -> [w260]
            tunnel: [w256] -> w198
            i -> [w263]
            n111 = Index Array(array=w266, index (row)=w263, index (col)=0 ("disabled index (col)")) -> ()  [unwired: 1 out]
            n112 = property on="Property Node" class="LstBox (strict)"(reference=w260, "CellFontSize"=u32 20 ("Active Row:Cell Font:Size")) -> (reference out=w259:refnum<vi>)  [unwired: 1 in, 1 out]
            n113 = property on="Property Node" class="LstBox (strict)"(reference=w259, "CellFontBold"=TRUE ("Active Row:Cell Font:Bold")) -> (reference out=w258:refnum<vi>)  [unwired: 1 in, 1 out]
            n114 = property on="Property Node" class="LstBox (strict)"(reference=w258, "Active Row"=w263) -> (reference out=w257:refnum<vi>)  [unwired: 1 in, 1 out]
            n115 = property on="Property Node" class="LstBox (strict)"(reference=w257, "CellBG"=u32 13816530 ("Active Row:Cell Background Color")) -> (reference out=w256:refnum<vi>)  [unwired: 1 in, 1 out]
          }
          n116 = Initialize Array(37, w197) -> (w214:i32[])
          n117 = property on="Property Node" class="LstBox (strict)"(reference=w198, "Item Symbols"=w214) -> ()  [unwired: 1 in, 2 out]
          n118 = property on="Property Node" class="LstBox (strict)"(reference=w198, "Item Names"=w202) -> ()  [unwired: 1 in, 2 out]
        }
        n119 = call-poly "Send Message.vi"("error in (no error)"=w167, "event buffer"="1000", "event"="multipleGraphs") -> ("error out"=w179:errorcluster)  [unwired: 8 in]
      }
      frame "initThermalProfile" {
        n120 = Unbundle By Name(w272) -> ("Http session"=w286:T16, "URL prefex"=w284:string)
        n121 = Concatenate Strings(w284, "getAllThermoCoupleData" ("url")) -> (w285:string)
        n122 = call <vilib>:"GET.vi"("client handle"=w286, "url"=w285, "error in (no error)"=w280) -> ("client handle out"=w273:T16, "body"=w282:string, "error out"=w269:errorcluster)  [unwired: 9 in, 1 out]
        n123 = call <vilib>:"Simple Error Handler.vi"("error source (\" \")"="Server Not Responding during Graph Initialization. Please Wait", "error in (no error)"=w269) -> ("error out"=w268:errorcluster)  [unwired: 3 in, 4 out]
        n124 = Unflatten From JSON(JSON string=w282, type and defaults=T19 {"time"="", "TCs"=[]} ("Cluster"), default null elements? (F)=TRUE, error in (no error)=w268) -> (value=w281:T19, error out=w270:errorcluster)  [unwired: 3 in]
        n125 = Bundle By Name(cluster=w272, "Http session"=w273) -> (w271:T17)
        n126 = for {
          N: 9 ("Numeric") -> [_]
          tunnel: w281 -> [w309]
          tunnel: w271 -> [w308]
          i -> [w299]
          w287 = ""
          w292 = 81 ("dimension size")
          w293 = 80
          n127 = Add(x=w293, y=1 ("index")) -> (x+y=w294:i32)
          n128 = Initialize Array("", w294) -> (w303:string[])
          n129 = Replace Array Subset(array=w303, new element="Clear Selection" ("new element/subarray"), index=0) -> (w297:string[])
          n130 = case shown="4" w299 {
            tunnel: [w315 w320 w325 w330 w335 w340 w345 w350 w355] -> w300
            tunnel: [w314 w319 w324 w329 w334 w339 w344 w349 w354] -> w291
            tunnel: [w313 w318 w323 w328 w333 w338 w343 w348 w353] -> w290
            tunnel: [w312 w317 w322 w327 w332 w337 w342 w347 w352] -> w289
            tunnel: [w311 w316 w321 w326 w331 w336 w341 w346 w351] -> w288
            frame 0, Default {
              n131 = control-ref of="Zone Thermocouples"() -> (w315:refnum<vi>)
              n132 = control-ref of="Thermocouples Selected"() -> (w314:refnum<vi>)
              n133 = control-ref of="Min Allowable Temp"() -> (w312:refnum<vi>)
              n134 = control-ref of="Max Temp Slope"() -> (w311:refnum<vi>)
              n135 = control-ref of="Max Allowable Temp"() -> (w313:refnum<vi>)
            }
            frame 1 {
              n136 = control-ref of="Max Temp Slope"() -> (w316:refnum<vi>)
              n137 = control-ref of="Max Allowable Temp"() -> (w318:refnum<vi>)
              n138 = control-ref of="Min Allowable Temp"() -> (w317:refnum<vi>)
              n139 = control-ref of="Thermocouples Selected"() -> (w319:refnum<vi>)
              n140 = control-ref of="Zone Thermocouples"() -> (w320:refnum<vi>)
            }
            frame 2 {
              n141 = control-ref of="Max Temp Slope"() -> (w321:refnum<vi>)
              n142 = control-ref of="Min Allowable Temp"() -> (w322:refnum<vi>)
              n143 = control-ref of="Thermocouples Selected"() -> (w324:refnum<vi>)
              n144 = control-ref of="Max Allowable Temp"() -> (w323:refnum<vi>)
              n145 = control-ref of="Zone Thermocouples"() -> (w325:refnum<vi>)
            }
            frame 3 {
              n146 = control-ref of="Max Allowable Temp"() -> (w328:refnum<vi>)
              n147 = control-ref of="Min Allowable Temp"() -> (w327:refnum<vi>)
              n148 = control-ref of="Max Temp Slope"() -> (w326:refnum<vi>)
              n149 = control-ref of="Zone Thermocouples"() -> (w330:refnum<vi>)
              n150 = control-ref of="Thermocouples Selected"() -> (w329:refnum<vi>)
            }
            frame 4 {
              n151 = control-ref of="Max Temp Slope"() -> (w331:refnum<vi>)
              n152 = control-ref of="Max Allowable Temp"() -> (w333:refnum<vi>)
              n153 = control-ref of="Min Allowable Temp"() -> (w332:refnum<vi>)
              n154 = control-ref of="Zone Thermocouples"() -> (w335:refnum<vi>)
              n155 = control-ref of="Thermocouples Selected"() -> (w334:refnum<vi>)
            }
            frame 5 {
              n156 = control-ref of="Min Allowable Temp"() -> (w337:refnum<vi>)
              n157 = control-ref of="Max Allowable Temp"() -> (w338:refnum<vi>)
              n158 = control-ref of="Max Temp Slope"() -> (w336:refnum<vi>)
              n159 = control-ref of="Thermocouples Selected"() -> (w339:refnum<vi>)
              n160 = control-ref of="Zone Thermocouples"() -> (w340:refnum<vi>)
            }
            frame 6 {
              n161 = control-ref of="Max Temp Slope"() -> (w341:refnum<vi>)
              n162 = control-ref of="Min Allowable Temp"() -> (w342:refnum<vi>)
              n163 = control-ref of="Max Allowable Temp"() -> (w343:refnum<vi>)
              n164 = control-ref of="Thermocouples Selected"() -> (w344:refnum<vi>)
              n165 = control-ref of="Zone Thermocouples"() -> (w345:refnum<vi>)
            }
            frame 7 {
              n166 = control-ref of="Max Temp Slope"() -> (w346:refnum<vi>)
              n167 = control-ref of="Min Allowable Temp"() -> (w347:refnum<vi>)
              n168 = control-ref of="Max Allowable Temp"() -> (w348:refnum<vi>)
              n169 = control-ref of="Thermocouples Selected"() -> (w349:refnum<vi>)
              n170 = control-ref of="Zone Thermocouples"() -> (w350:refnum<vi>)
            }
            frame 8 {
              n171 = control-ref of="Min Allowable Temp"() -> (w352:refnum<vi>)
              n172 = control-ref of="Max Allowable Temp"() -> (w353:refnum<vi>)
              n173 = control-ref of="Zone Thermocouples"() -> (w355:refnum<vi>)
              n174 = control-ref of="Thermocouples Selected"() -> (w354:refnum<vi>)
              n175 = control-ref of="Max Temp Slope"() -> (w351:refnum<vi>)
            }
          }
          n176 = Unbundle By Name(w309) -> ("TCs"=w305:T14)
          n177 = for {
            N: w293 -> [_]
            tunnel: w305 -> [w362] mode=indexing
            shift-right: [w356] -> w296
            shift-left: w297 -> [w358]
            i -> [w360]
            n178 = Unbundle By Name(w362) -> ("thermocouple"=w363:i32)
            n179 = Number To Decimal String(number=w363) -> (decimal integer string=w365:string)  [unwired: 1 in]
            n180 = Add(x=1 ("index"), y=w360) -> (x+y=w359:i32)
            n181 = Concatenate Strings("TC " ("string"), w365) -> (w357:string)
            n182 = Replace Array Subset(array=w358, new element=w357, index=w359) -> (w356:string[])
          }
          n183 = property class="Str"(reference=w291, "Text.Text"=w287) -> ()  [unwired: 1 in, 2 out]
          n184 = property class="Str"(reference=w290, "Value"=w287) -> ()  [unwired: 1 in, 2 out]
          n185 = property class="Str"(reference=w288, "Value"=w287) -> ()  [unwired: 1 in, 2 out]
          n186 = property class="Str"(reference=w289, "Value"=w287) -> ()  [unwired: 1 in, 2 out]
          n187 = Unbundle By Name(w308) -> ("Thermocouples"=w310:T3)
          n188 = for {
            N: w292 -> [_]
            tunnel: w310 -> [w376]
            tunnel: w300 -> [w370]
            tunnel: [w366] -> w298
            i -> [w373]
            n189 = Index Array(array=w376, index (row)=w373, index (col)=0 ("disabled index (col)")) -> ()  [unwired: 1 out]
            n190 = property on="Property Node" class="LstBox (strict)"(reference=w370, "CellFontSize"=u32 20 ("Active Row:Cell Font:Size")) -> (reference out=w369:refnum<vi>)  [unwired: 1 in, 1 out]
            n191 = property on="Property Node" class="LstBox (strict)"(reference=w369, "CellFontBold"=TRUE ("Active Row:Cell Font:Bold")) -> (reference out=w368:refnum<vi>)  [unwired: 1 in, 1 out]
            n192 = property on="Property Node" class="LstBox (strict)"(reference=w368, "Active Row"=w373) -> (reference out=w367:refnum<vi>)  [unwired: 1 in, 1 out]
            n193 = property on="Property Node" class="LstBox (strict)"(reference=w367, "CellBG"=u32 13816530 ("Active Row:Cell Background Color")) -> (reference out=w366:refnum<vi>)  [unwired: 1 in, 1 out]
          }
          n194 = Initialize Array(37, w292) -> (w306:i32[])
          n195 = property on="Property Node" class="LstBox (strict)"(reference=w298, "Item Symbols"=w306) -> ()  [unwired: 1 in, 2 out]
          n196 = property on="Property Node" class="LstBox (strict)"(reference=w298, "Item Names"=w296) -> ()  [unwired: 1 in, 2 out]
        }
        n197 = call-poly "Send Message.vi"("error in (no error)"=w270, "event buffer"="1000", "event"="multipleGraphs") -> ("error out"=w277:errorcluster)  [unwired: 8 in]
      }
      frame "", "Idle" {
        n198 = control-ref of="Thermocouples"() -> (w389:refnum<vi>)
        n199 = property on="Property Node" class="Arr (strict)"(reference=w389) -> ("Position"=w388:T11)  [unwired: 1 in, 2 out]
        n200 = Unbundle By Name(w388) -> ("Left"=w387:i32, "Top"=w385:i32)
        n201 = Add(x=4, y=w387) -> (x+y=w383:i32)
        n202 = Add(x=w385, y=23 ("x")) -> (x+y=w382:i32)
        n203 = event shown="[27] \"Current Errors (click to clear)\": Mouse Down" {
          selector: _ -> [_ _ _ _ _ _ _ _ _ _ _ _ _ _ _ _ _ _ _ _ _ _ _ _ _ _ _ _ _ _ _ _ _ _ _ _ _ _ _ _ _ _ _ _ _ _]
          dyn-events: _ -> [_ _ _ _ _ _ _ _ _ _ _ _ _ _ _ _ _ _ _ _ _ _ _ _ _ _ _ _ _ _ _ _ _ _ _ _ _ _ _ _ _ _ _ _ _ _]
          timeout: 200 ("milliseconds to wait") -> [_ _ _ _ _ _ _ _ _ _ _ _ _ _ _ _ _ _ _ _ _ _ _ _ _ _ _ _ _ _ _ _ _ _ _ _ _ _ _ _ _ _ _ _ _ _]
          tunnel: [w390 w475 w489 w503 w517 w531 w545 w558 w579 w672 w736 w801 w866 w931 w996 w1061 w1126 w1190 w1196 w1249 w1265 w1275 w1281 w1305 w1329 w1340 w1514 w1596 w1628 w1673 w1715 w1746 w1766 w1856 w1910 w1964 w2018 w2072 w2126 w2180 w2234 w2288 w2339 w2343 w2353 w2370] -> w380
          tunnel: [w399 w477 w491 w505 w519 w533 w547 w562 w580 w666 w737 w802 w867 w932 w997 w1062 w1127 w1193 w1209 w1239 w1259 w1273 w1278 w1302 w1326 w1345 w1512 w1592 w1624 w1671 w1713 w1741 w1778 w1855 w1909 w1963 w2017 w2071 w2125 w2179 w2233 w2287 w2341 w2345 w2359 w2373] -> w377
          tunnel: w379 -> [w400 w477 w491 w505 w519 w533 w547 w562 w581 w668 w737 w802 w867 w932 w997 w1062 w1127 w1194 w1200 w1240 w1260 w1274 w1279 w1303 w1327 w1346 w1513 w1593 w1625 w1672 w1714 w1742 w1778 w1855 w1909 w1963 w2017 w2071 w2125 w2179 w2233 w2287 w2341 w2345 w2359 w2373]
          tunnel: w383 -> [_ _ _ _ _ _ _ _ w578 _ _ _ _ _ _ _ _ _ _ _ _ _ _ _ _ _ _ _ _ _ _ _ _ _ _ _ _ _ _ _ _ _ _ _ _ _]
          tunnel: w382 -> [_ _ _ _ _ _ _ _ w575 _ _ _ _ _ _ _ _ _ _ _ _ _ _ _ _ _ _ _ _ _ _ _ _ _ _ _ _ _ _ _ _ _ _ _ _ _]
          tunnel: w381 -> [w395 w476 w490 w504 w518 w532 w546 w559 w579 w672 w736 w801 w866 w931 w996 w1061 w1126 w1187 w1201 w1249 w1265 w1275 w1282 w1306 w1330 w1336 w1515 w1596 w1628 w1673 w1715 w1746 w1767 w1856 w1910 w1964 w2018 w2072 w2126 w2180 w2234 w2288 w2340 w2344 w2356 w2372]
          event Timeout {
            n204 = event-data() -> ("Time"=w398:u32)  [unwired: 1 in, 1 out]
            n205 = Unbundle By Name(w400) -> ("Time"=w403:i32)
            n206 = Subtract(x=w398, y=w403) -> (x-y=w402:u32)
            n207 = Greater?(x=w402, y=u32 5000 ("millisecond multiple")) -> (0:w391:bool)
            n208 = case shown="True" w391 {
              tunnel: w400 -> [w407 w430]
              tunnel: [w407 w429] -> w399
              tunnel: w398 -> [_ w428]
              tunnel: [w406 w408] -> w397
              tunnel: w395 -> [w406 w427]
              frame False {
              }
              frame True {
                n209 = case shown="True" "TCs On" {
                  tunnel: w427 -> [w441 w445]
                  tunnel: [w441 w443] -> w426
                  frame False {
                  }
                  frame True {
                    n210 = call-poly "Send Message.vi"("Destination Module"="getData.vi", "error in (no error)"=w445, "event"="getTC") -> ("error out"=w443:errorcluster)  [unwired: 8 in]
                  }
                }
                n211 = Bundle By Name(cluster=w430, "Time"=w428) -> (w429:T17)
                n212 = case shown="True" "Pressure On" {
                  tunnel: w426 -> [w461 w464]
                  tunnel: [w461 w462] -> w425
                  frame False {
                  }
                  frame True {
                    n213 = call-poly "Send Message.vi"("Destination Module"="getData.vi", "error in (no error)"=w464, "event"="getPressure") -> ("error out"=w462:errorcluster)  [unwired: 8 in]
                  }
                }
                n214 = case shown="True" "MCC On" {
                  tunnel: w425 -> [w456 w458]
                  tunnel: [w456 w457] -> w424
                  frame False {
                  }
                  frame True {
                    n215 = call-poly "Send Message.vi"("Destination Module"="getData.vi", "error in (no error)"=w458, "event"="getMCCData") -> ("error out"=w457:errorcluster)  [unwired: 8 in]
                  }
                }
                n216 = case shown="True" "ZoneTemps On" {
                  tunnel: w424 -> [w451 w455]
                  tunnel: [w451 w452] -> w423
                  frame False {
                  }
                  frame True {
                    n217 = call-poly "Send Message.vi"("Destination Module"="getData.vi", "error in (no error)"=w455, "event"="getZoneTemps") -> ("error out"=w452:errorcluster)  [unwired: 8 in]
                  }
                }
                n218 = case shown="True" "Compressor On" {
                  tunnel: w423 -> [w446 w448]
                  tunnel: [w446 w447] -> w422
                  frame False {
                  }
                  frame True {
                    n219 = call-poly "Send Message.vi"("Destination Module"="getData.vi", "error in (no error)"=w448, "event"="getCompressorTemp") -> ("error out"=w447:errorcluster)  [unwired: 8 in]
                  }
                }
                n220 = case shown="True" "GetError" {
                  tunnel: w422 -> [w466 w468]
                  tunnel: [w466 w467] -> w415
                  frame False {
                  }
                  frame True {
                    n221 = call-poly "Send Message.vi"("Destination Module"="getData.vi", "error in (no error)"=w468, "event"="getLastError") -> ("error out"=w467:errorcluster)  [unwired: 8 in]
                  }
                }
                n222 = case shown="True" "GetEvent" {
                  tunnel: w415 -> [w436 w439]
                  tunnel: [w436 w438] -> w413
                  frame False {
                  }
                  frame True {
                    n223 = call-poly "Send Message.vi"("Destination Module"="getData.vi", "error in (no error)"=w439, "event"="getLastEvent") -> ("error out"=w438:errorcluster)  [unwired: 8 in]
                  }
                }
                n224 = case shown="True" "getTvacStatus" {
                  tunnel: w413 -> [w431 w434]
                  tunnel: [w431 w433] -> w409
                  frame False {
                  }
                  frame True {
                    n225 = call-poly "Send Message.vi"("Destination Module"="getData.vi", "error in (no error)"=w434, "event"="getTvacStatus") -> ("error out"=w433:errorcluster)  [unwired: 8 in]
                  }
                }
                n226 = call-poly "Send Message.vi"("Destination Module"="getData.vi" ("event"), "error in (no error)"=w409, "event"="getDatabase") -> ("error out"=w408:errorcluster)  [unwired: 8 in]
              }
            }
            n227 = call-poly "Send Message.vi"("error in (no error)"=w397, "event"="masterDatabase") -> ("error out"=w394:errorcluster)  [unwired: 9 in]
            n228 = call-poly "Send Message.vi"("error in (no error)"=w394, "event"="graphTC") -> ("error out"=w393:errorcluster)  [unwired: 9 in]
            n229 = call-poly "Send Message.vi"("error in (no error)"=w393, "event buffer"="1000", "event"="multipleGraphs") -> ("error out"=w390:errorcluster)  [unwired: 8 in]
          }
          event "Custom Chart 1 Selection": Mouse Down {
            n230 = event-data() -> ("CtlRef"=w474:refnum<vi>, "Coords"=w473:T30)  [unwired: 1 in, 6 out]
            n231 = invoke on="Invoke Node" class="LstBox (strict)" method="Point To Row"(reference=w474, "Point"=w473) -> ("InBounds"=w471:bool, "Row"=w472:i32)  [unwired: 5 in, 5 out]
            n232 = case shown="True" w471 {
              tunnel: w476 -> [w478 w484]
              tunnel: [w478 w483] -> w475
              tunnel: w472 -> [_ w479]
              frame False {
              }
              frame True {
                n233 = local write "Custom Graph Selector"(0) -> ()
                n234 = Number To Decimal String(number=w479) -> (decimal integer string=w481:string)  [unwired: 1 in]
                n235 = call-poly "Send Message.vi"("error in (no error)"=w484, "event buffer"=w481, "event"="multipleGraphs") -> ("error out"=w483:errorcluster)  [unwired: 8 in]
              }
            }
          }
          event "Custom Chart 2 Selection": Mouse Down {
            n236 = event-data() -> ("CtlRef"=w488:refnum<vi>, "Coords"=w487:T30)  [unwired: 1 in, 6 out]
            n237 = invoke on="Invoke Node" class="LstBox (strict)" method="Point To Row"(reference=w488, "Point"=w487) -> ("InBounds"=w485:bool, "Row"=w486:i32)  [unwired: 5 in, 5 out]
            n238 = case shown="True" w485 {
              tunnel: w490 -> [w492 w498]
              tunnel: [w492 w497] -> w489
              tunnel: w486 -> [_ w493]
              frame False {
              }
              frame True {
                n239 = local write "Custom Graph Selector"(1) -> ()
                n240 = Number To Decimal String(number=w493) -> (decimal integer string=w495:string)  [unwired: 1 in]
                n241 = call-poly "Send Message.vi"("error in (no error)"=w498, "event buffer"=w495, "event"="multipleGraphs") -> ("error out"=w497:errorcluster)  [unwired: 8 in]
              }
            }
          }
          event "Custom Chart 3 Selection": Mouse Down {
            n242 = event-data() -> ("CtlRef"=w502:refnum<vi>, "Coords"=w501:T30)  [unwired: 1 in, 6 out]
            n243 = invoke on="Invoke Node" class="LstBox (strict)" method="Point To Row"(reference=w502, "Point"=w501) -> ("InBounds"=w499:bool, "Row"=w500:i32)  [unwired: 5 in, 5 out]
            n244 = case shown="False" w499 {
              tunnel: w504 -> [w506 w512]
              tunnel: [w506 w511] -> w503
              tunnel: w500 -> [_ w507]
              frame False {
              }
              frame True {
                n245 = local write "Custom Graph Selector"(2) -> ()
                n246 = Number To Decimal String(number=w507) -> (decimal integer string=w509:string)  [unwired: 1 in]
                n247 = call-poly "Send Message.vi"("error in (no error)"=w512, "event buffer"=w509, "event"="multipleGraphs") -> ("error out"=w511:errorcluster)  [unwired: 8 in]
              }
            }
          }
          event "Custom Chart 4 Selection": Mouse Down {
            n248 = event-data() -> ("CtlRef"=w516:refnum<vi>, "Coords"=w515:T30)  [unwired: 1 in, 6 out]
            n249 = invoke on="Invoke Node" class="LstBox (strict)" method="Point To Row"(reference=w516, "Point"=w515) -> ("InBounds"=w513:bool, "Row"=w514:i32)  [unwired: 5 in, 5 out]
            n250 = case shown="False" w513 {
              tunnel: w518 -> [w520 w526]
              tunnel: [w520 w525] -> w517
              tunnel: w514 -> [_ w521]
              frame False {
              }
              frame True {
                n251 = local write "Custom Graph Selector"(3) -> ()
                n252 = Number To Decimal String(number=w521) -> (decimal integer string=w523:string)  [unwired: 1 in]
                n253 = call-poly "Send Message.vi"("error in (no error)"=w526, "event buffer"=w523, "event"="multipleGraphs") -> ("error out"=w525:errorcluster)  [unwired: 8 in]
              }
            }
          }
          event "Custom Chart 5 Selection": Mouse Down {
            n254 = event-data() -> ("CtlRef"=w530:refnum<vi>, "Coords"=w529:T30)  [unwired: 1 in, 6 out]
            n255 = invoke on="Invoke Node" class="LstBox (strict)" method="Point To Row"(reference=w530, "Point"=w529) -> ("InBounds"=w527:bool, "Row"=w528:i32)  [unwired: 5 in, 5 out]
            n256 = case shown="False" w527 {
              tunnel: w532 -> [w534 w540]
              tunnel: [w534 w539] -> w531
              tunnel: w528 -> [_ w535]
              frame False {
              }
              frame True {
                n257 = Number To Decimal String(number=w535) -> (decimal integer string=w537:string)  [unwired: 1 in]
                n258 = local write "Custom Graph Selector"(4) -> ()
                n259 = call-poly "Send Message.vi"("error in (no error)"=w540, "event buffer"=w537, "event"="multipleGraphs") -> ("error out"=w539:errorcluster)  [unwired: 8 in]
              }
            }
          }
          event "Custom Chart 6 Selection": Mouse Down {
            n260 = event-data() -> ("CtlRef"=w544:refnum<vi>, "Coords"=w543:T30)  [unwired: 1 in, 6 out]
            n261 = invoke on="Invoke Node" class="LstBox (strict)" method="Point To Row"(reference=w544, "Point"=w543) -> ("InBounds"=w541:bool, "Row"=w542:i32)  [unwired: 5 in, 5 out]
            n262 = case shown="False" w541 {
              tunnel: w546 -> [w548 w554]
              tunnel: [w548 w553] -> w545
              tunnel: w542 -> [_ w549]
              frame False {
              }
              frame True {
                n263 = local write "Custom Graph Selector"(5) -> ()
                n264 = Number To Decimal String(number=w549) -> (decimal integer string=w551:string)  [unwired: 1 in]
                n265 = call-poly "Send Message.vi"("error in (no error)"=w554, "event buffer"=w551, "event"="multipleGraphs") -> ("error out"=w553:errorcluster)  [unwired: 8 in]
              }
            }
          }
          event "Tab Control": Value Change {
            n266 = event-data() -> ("NewVal"=w555:T2)  [unwired: 1 in, 5 out]
            n267 = Equal?(x=w555, y=enum16{"Graphs"}."Graphs") -> (x = y?=w560:bool)
            n268 = case shown="True" w560 {
              tunnel: w559 -> [w569 w571]
              tunnel: [w569 w570] -> w558
              frame False {
              }
              frame True {
                n269 = call-poly "Send Message.vi"("error in (no error)"=w571, "event"="getGraphs") -> ("error out"=w570:errorcluster)  [unwired: 9 in]
              }
            }
            n270 = Equal?(x=w555, y=T2."Engineering Interface") -> (x = y?=w556:bool)
            n271 = case shown="True" w556 {
              frame False {
              }
              frame True {
                n272 = call "Unlock Engineering Mode"() -> ("Password"=w563:string)  [unwired: 17 in, 2 out]
                n273 = Equal?(x=w563, y="admin") -> (x = y?=w565:bool)
                n274 = case shown="False" w565 {
                  frame False {
                    n275 = local write "Tab Control"(T2."General Status" ("Tab Control")) -> ()
                    n276 = One Button Dialog(message="Access Denied") -> ()  [unwired: 1 in, 1 out]
                  }
                  frame True {
                    n277 = local write "Engineering"("Unlocked!" ("Engineering")) -> ()
                  }
                }
              }
            }
          }
          event "Thermocouples": Mouse Down {
            n278 = event-data() -> ("CtlRef"=w583:refnum<vi>, "Coords"=w588:T30)  [unwired: 1 in, 3 out]
            n279 = Unbundle By Name(w588) -> ("Horizontal"=w586:i32, "Vertical"=w585:i32)
            n280 = Add(x=783 ("y"), y=w578) -> (x+y=w573:i32)
            n281 = Less?(x=w586, y=w573) -> (x < y?=w587:bool)
            n282 = Add(x=w575, y=854) -> (x+y=w574:i32)
            n283 = Less?(x=w585, y=w574) -> (x < y?=w584:bool)
            n284 = And(x=w587, y=w584) -> (x .and. y?=w582:bool)
            n285 = case shown="True" w582 {
              tunnel: w583 -> [_ w630]
              tunnel: w581 -> [_ w602]
              tunnel: w581 -> [w589 w600]
              tunnel: [w589 w592] -> w580
              tunnel: w578 -> [_ w591]
              tunnel: w575 -> [_ w590]
              frame False {
              }
              frame True {
                w624 = u16 0 items=["User Selection", "Graph All Thermocouples", "Clear Graph"] ("Graphing Selection")
                n286 = property class="Arr (strict)"(reference=w630) -> ("Array Element.Position"=w622:T11)  [unwired: 1 in, 2 out]
                n287 = local write "Graphing Selection"(w624) -> ()
                n288 = Unbundle By Name(w622) -> ("Left"=w620:i32, "Top"=w623:i32)
                n289 = property on="Thermocouples" class="Arr (strict)"() -> ("Index Values"=w614:u32[])  [unwired: 2 in, 2 out]
                n290 = Subtract(x=w591, y=w620) -> (x-y=w619:i32)
                n291 = Subtract(x=w590, y=w623) -> (x-y=w611:i32)
                n292 = Absolute Value(x=w611) -> (abs(x)=w621:i32)
                n293 = Index Array(array=w614, index=0) -> (element=w610:u32)
                n294 = To Byte Integer(number=w610) -> (8bit integer=w609:i8)
                n295 = Absolute Value(x=w619) -> (abs(x)=w618:i32)
                n296 = local read "Thermocouples"() -> (w593:T3)
                n297 = Quotient & Remainder(x=w621, y=42) -> (floor(x/y)=w608:i32)  [unwired: 1 out]
                n298 = Add(x=w609, y=w608) -> (x+y=w595:i32)
                n299 = Quotient & Remainder(x=w618, y=197 ("Numeric 2")) -> (floor(x/y)=w594:i32)  [unwired: 1 out]
                n300 = Index Array(array=w593, index (row)=w595, index (col)=w594) -> (element=w596:T18)
                n301 = Multiply(x=4, y=w595) -> (x*y=w615:i32)
                n302 = Unbundle By Name(w602) -> ("working array"=w601:bool[])  [unwired: 1 out]
                n303 = Unbundle By Name(w596) -> ("Alarm Color"=w628:u32, "Graph On/Off"=w627:u32, "TC Label"=w626:string, "PlotColor"=w607:u32, "Alarm Status"=w625:string, "Temperature"=w598:string)
                n304 = Add(x=w615, y=w594) -> (x+y=w604:i32)
                n305 = control-ref of="Waveform Chart"() -> (w629:refnum<vi>)
                n306 = Index Array(array=w601, index=w604) -> (element=w603:bool)
                n307 = Decimal String To Number(string=w598) -> ()  [unwired: 2 in, 2 out]
                n308 = Equal?(x=w627, y=u32 12369084) -> (x = y?=w605:bool)
                n309 = case shown="True" w603 {
                  selector: w603 -> [_ w636]
                  tunnel: w629 -> [_ w642]
                  tunnel: w628 -> [_ w641]
                  tunnel: w626 -> [_ w640]
                  tunnel: w625 -> [_ w639]
                  tunnel: w604 -> [_ w632]
                  tunnel: w607 -> [_ w638]
                  tunnel: w605 -> [_ w637]
                  tunnel: w598 -> [_ w635]
                  tunnel: [w631 w634] -> w597
                  tunnel: w596 -> [w631 w633]
                  frame False {
                  }
                  frame True {
                    n310 = case shown="True" w637 {
                      tunnel: w642 -> [w652 w663]
                      tunnel: w641 -> [w646 w658]
                      tunnel: w640 -> [w647 w657]
                      tunnel: w639 -> [w648 w659]
                      tunnel: w638 -> [_ w661]
                      tunnel: w636 -> [_ _]
                      tunnel: w635 -> [w649 w660]
                      tunnel: [w644 w656] -> w634
                      tunnel: w633 -> [w645 w655]
                      tunnel: w632 -> [w643 w654]
                      frame False {
                        w650 = u32 12369084
                        n311 = property on="Property Node" class="WFChart (strict)"(reference=w652, "Active Plot"=w643) -> (reference out=w653:refnum<vi>)  [unwired: 1 in, 1 out]
                        n312 = Bundle By Name(cluster=w645, "Graph On/Off"=w650, "TC Label"=w647, "PlotColor"=w650, "Temperature"=w649, "Alarm Color"=w646, "Alarm Status"=w648) -> (w644:T18)
                        n313 = property class="WFChart (strict)"(reference=w653, "Plot.Visible?"=FALSE ("Plot.Visible")) -> ()  [unwired: 1 in, 2 out]
                      }
                      frame True {
                        n314 = property class="WFChart (strict)"(reference=w663, "Active Plot"=w654) -> (reference out=w664:refnum<vi>)  [unwired: 1 in, 1 out]
                        n315 = Bundle By Name(cluster=w655, "Graph On/Off"=u32 6618880, "TC Label"=w657, "PlotColor"=w661, "Temperature"=w660, "Alarm Color"=w658, "Alarm Status"=w659) -> (w656:T18)
                        n316 = property class="WFChart (strict)"(reference=w664, "Plot.Visible?"=TRUE ("Plot.Visible")) -> ()  [unwired: 1 in, 2 out]
                      }
                    }
                  }
                }
                n317 = Replace Array Subset(array=w593, new element=w597, index (row)=w595, index (col)=w594) -> (w599:T3)
                n318 = Bundle By Name(cluster=w600, "Thermocouples"=w599) -> (w592:T17)
              }
            }
          }
          event "Graphing Selection": Value Change {
            n319 = event-data() -> ("NewVal"=w673:u16)  [unwired: 1 in, 5 out]
            n320 = Unbundle By Name(w668) -> ("Thermocouples"=w667:T3, "working array"=w670:bool[])
            n321 = control-ref of="Waveform Chart"() -> (w674:refnum<vi>)
            n322 = case shown="1" w673 {
              tunnel: w667 -> [w675 w680 w711]
              tunnel: w674 -> [_ w679 w710]
              tunnel: 120 ("disabled index (col)") -> [_ w678 w709]
              tunnel: w668 -> [_ _ _]
              tunnel: w670 -> [_ w677 _]
              tunnel: [w675 w676 w708] -> w669
              frame 0, Default {
              }
              frame 1 {
                n323 = for {
                  N: w678 -> [_]
                  tunnel: w679 -> [w686]
                  shift-right: [w681] -> w676
                  shift-left: w680 -> [w685]
                  tunnel: w677 -> [w682]
                  i -> [w684]
                  n324 = Index Array(array=w682, index=w684) -> (element=w683:bool)
                  n325 = case shown="True" w683 {
                    tunnel: w686 -> [_ w707]
                    tunnel: w685 -> [w687 w688]
                    tunnel: [w687 w689] -> w681
                    tunnel: w684 -> [_ w706]
                    frame False {
                    }
                    frame True {
                      n326 = Quotient & Remainder(x=w706, y=4) -> (x-y*floor(x/y)=w692:i32, floor(x/y)=w691:i32)
                      n327 = Multiply(x=4, y=w691) -> (x*y=w702:i32)
                      n328 = Add(x=w702, y=w692) -> (x+y=w701:i32)
                      n329 = property class="WFChart (strict)"(reference=w707, "Active Plot"=w701) -> (reference out=w704:refnum<vi>)  [unwired: 1 in, 1 out]
                      n330 = Index Array(array=w688, index (row)=w691, index (col)=w692) -> (element=w690:T18)
                      n331 = Unbundle By Name(w690) -> ("TC Label"=w693:string, "Alarm Status"=w699:string, "Temperature"=w698:string, "PlotColor"=w695:u32, "Alarm Color"=w694:u32)
                      n332 = property class="WFChart (strict)"(reference=w704, "Plot.Visible?"=TRUE ("Plot.Visible")) -> ()  [unwired: 1 in, 2 out]
                      n333 = Bundle By Name(cluster=w690, "TC Label"=w693, "Alarm Status"=w699, "Alarm Color"=w694, "Temperature"=w698, "PlotColor"=w695, "Graph On/Off"=u32 6618880) -> (w697:T18)
                      n334 = Replace Array Subset(array=w688, new element=w697, index (row)=w691, index (col)=w692) -> (w689:T3)
                    }
                  }
                }
              }
              frame 2 {
                n335 = for {
                  N: w709 -> [_]
                  tunnel: w710 -> [w729]
                  shift-right: [w712] -> w708
                  shift-left: w711 -> [w716]
                  i -> [w730]
                  w722 = u32 12369084
                  n336 = local read "working array"() -> (w731:bool[])
                  n337 = Quotient & Remainder(x=w730, y=4 ("Numeric")) -> (x-y*floor(x/y)=w714:i32, floor(x/y)=w713:i32)
                  n338 = Index Array(array=w716, index (row)=w713, index (col)=w714) -> (element=w721:T18)
                  n339 = Multiply(x=4, y=w713) -> (x*y=w725:i32)
                  n340 = Add(x=w725, y=w714) -> (x+y=w724:i32)
                  n341 = Index Array(array=w731, index=w730) -> ()  [unwired: 1 out]
                  n342 = property class="WFChart (strict)"(reference=w729, "Active Plot"=w724) -> (reference out=w727:refnum<vi>)  [unwired: 1 in, 1 out]
                  n343 = Unbundle By Name(w721) -> ("TC Label"=w720:string, "Alarm Status"=w719:string, "Temperature"=w718:string, "PlotColor"=w717:u32)
                  n344 = property class="WFChart (strict)"(reference=w727, "Plot.Visible?"=FALSE ("Plot.Visible")) -> ()  [unwired: 1 in, 2 out]
                  n345 = Bundle By Name(cluster=w721, "TC Label"=w720, "Alarm Status"=w719, "Alarm Color"=w722, "Temperature"=w718, "PlotColor"=w717, "Graph On/Off"=w722) -> (w715:T18)
                  n346 = Replace Array Subset(array=w716, new element=w715, index (row)=w713, index (col)=w714) -> (w712:T3)
                }
              }
            }
            n347 = Bundle By Name(cluster=w668, "Thermocouples"=w669) -> (w666:T17)
          }
          event "Set Time TC Graph": Mouse Down {
            n348 = event-data() -> ()  [unwired: 1 in, 8 out]
            n349 = local read "Log/Linear Y-Axis"() -> (w732:u16)
            n350 = control-ref of="Waveform Chart"() -> (w733:refnum<vi>)
            n351 = property on="Property Node" class="WFChart (strict)"(reference=w733, "YScale.Mapping Mode"=w732) -> ()  [unwired: 1 in, 2 out]
            n352 = case shown="0, Default" w732 {
              tunnel: w733 -> [w738 w740]
              frame 0, Default {
                n353 = property class="WFChart (strict)"(reference=w738, "YScale.LooseFit"=TRUE ("Y Scale.Flipped")) -> ()  [unwired: 1 in, 2 out]
              }
              frame 1 {
                n354 = property class="WFChart (strict)"(reference=w740, "YScale.LooseFit"=FALSE ("Y Scale.Flipped")) -> ()  [unwired: 1 in, 2 out]
              }
            }
            n355 = local read "Total Time"() -> (w734:dbl)
            n356 = local read "Time Scale"() -> (w735:u16)
            n357 = case shown="1" w735 {
              tunnel: w733 -> [w744 w763 w782]
              tunnel: w734 -> [w742 w761 w780]
              frame 0, Default {
                n358 = Not Equal To 0?(x=w742) -> (x != 0?=w743:bool)
                n359 = case shown="True" w743 {
                  tunnel: w744 -> [w746 w758]
                  tunnel: w742 -> [_ w752]
                  frame False {
                    n360 = property on="Property Node" class="WFChart (strict)"(reference=w746) -> (reference out=w745:refnum<vi>, "XScale.Range"=w751:T31)  [unwired: 1 in, 1 out]
                    n361 = Bundle By Name(cluster=w751, "Minimum"=0.0, "Maximum"=3600.0, "Increment"=60.0) -> (w750:T31)
                    n362 = property on="Property Node" class="WFChart (strict)"(reference=w745, "XScale.Range"=w750) -> ()  [unwired: 1 in, 2 out]
                  }
                  frame True {
                    n363 = property on="Property Node" class="WFChart (strict)"(reference=w758) -> (reference out=w755:refnum<vi>, "XScale.Range"=w760:T31)  [unwired: 1 in, 1 out]
                    n364 = Multiply(x=w752, y=60.0) -> (x*y=w754:dbl)
                    n365 = Bundle By Name(cluster=w760, "Minimum"=0.0, "Maximum"=w754, "Increment"=1.0) -> (w759:T31)
                    n366 = property on="Property Node" class="WFChart (strict)"(reference=w755, "XScale.Range"=w759) -> ()  [unwired: 1 in, 2 out]
                  }
                }
              }
              frame 1 {
                n367 = Not Equal To 0?(x=w761) -> (x != 0?=w762:bool)
                n368 = case shown="True" w762 {
                  tunnel: w763 -> [w765 w775]
                  tunnel: w761 -> [_ w772]
                  frame False {
                    n369 = property on="Property Node" class="WFChart (strict)"(reference=w765) -> (reference out=w764:refnum<vi>, "XScale.Range"=w770:T31)  [unwired: 1 in, 1 out]
                    n370 = Bundle By Name(cluster=w770, "Minimum"=0.0, "Maximum"=43200.0, "Increment"=3600.0) -> (w766:T31)
                    n371 = property on="Property Node" class="WFChart (strict)"(reference=w764, "XScale.Range"=w766) -> ()  [unwired: 1 in, 2 out]
                  }
                  frame True {
                    n372 = Multiply(x=w772, y=3600.0) -> (x*y=w771:dbl)
                    n373 = property on="Property Node" class="WFChart (strict)"(reference=w775) -> (reference out=w774:refnum<vi>, "XScale.Range"=w779:T31)  [unwired: 1 in, 1 out]
                    n374 = Bundle By Name(cluster=w779, "Minimum"=0.0, "Maximum"=w771, "Increment"=3600.0) -> (w776:T31)
                    n375 = property on="Property Node" class="WFChart (strict)"(reference=w774, "XScale.Range"=w776) -> ()  [unwired: 1 in, 2 out]
                  }
                }
              }
              frame 2 {
                n376 = Not Equal To 0?(x=w780) -> (x != 0?=w781:bool)
                n377 = case shown="True" w781 {
                  tunnel: w782 -> [w784 w792]
                  tunnel: w780 -> [_ w790]
                  frame False {
                    n378 = property on="Property Node" class="WFChart (strict)"(reference=w784) -> (reference out=w783:refnum<vi>, "XScale.Range"=w789:T31)  [unwired: 1 in, 1 out]
                    n379 = Bundle By Name(cluster=w789, "Minimum"=0.0, "Maximum"=60.0, "Increment"=1.0) -> (w785:T31)
                    n380 = property on="Property Node" class="WFChart (strict)"(reference=w783, "XScale.Range"=w785) -> ()  [unwired: 1 in, 2 out]
                  }
                  frame True {
                    n381 = property on="Property Node" class="WFChart (strict)"(reference=w792) -> (reference out=w791:refnum<vi>, "XScale.Range"=w796:T31)  [unwired: 1 in, 1 out]
                    n382 = Bundle By Name(cluster=w796, "Minimum"=0.0, "Maximum"=w790, "Increment"=1.0) -> (w793:T31)
                    n383 = property on="Property Node" class="WFChart (strict)"(reference=w791, "XScale.Range"=w793) -> ()  [unwired: 1 in, 2 out]
                  }
                }
              }
            }
          }
          event "Set Time TC Graph 1": Mouse Down {
            n384 = event-data() -> ()  [unwired: 1 in, 8 out]
            n385 = local read "Log/Linear Y-Axis 1"() -> (w797:u16)
            n386 = control-ref of="Custom Chart 1"() -> (w798:refnum<vi>)
            n387 = case shown="0, Default" w797 {
              tunnel: w798 -> [w803 w805]
              frame 0, Default {
                n388 = property class="WFChart (strict)"(reference=w803, "YScale.LooseFit"=TRUE ("Y Scale.Flipped")) -> ()  [unwired: 1 in, 2 out]
              }
              frame 1 {
                n389 = property class="WFChart (strict)"(reference=w805, "YScale.LooseFit"=FALSE ("Y Scale.Flipped")) -> ()  [unwired: 1 in, 2 out]
              }
            }
            n390 = property on="Property Node" class="WFChart (strict)"(reference=w798, "YScale.Mapping Mode"=w797) -> ()  [unwired: 1 in, 2 out]
            n391 = local read "Total Time 1"() -> (w799:dbl)
            n392 = local read "Time Scale 1"() -> (w800:u16)
            n393 = case shown="0, Default" w800 {
              tunnel: w798 -> [w809 w828 w847]
              tunnel: w799 -> [w807 w826 w845]
              frame 0, Default {
                n394 = Not Equal To 0?(x=w807) -> (x != 0?=w808:bool)
                n395 = case shown="True" w808 {
                  tunnel: w809 -> [w811 w823]
                  tunnel: w807 -> [_ w817]
                  frame False {
                    n396 = property on="Property Node" class="WFChart (strict)"(reference=w811) -> (reference out=w810:refnum<vi>, "XScale.Range"=w816:T31)  [unwired: 1 in, 1 out]
                    n397 = Bundle By Name(cluster=w816, "Minimum"=0.0, "Maximum"=3600.0, "Increment"=60.0) -> (w815:T31)
                    n398 = property on="Property Node" class="WFChart (strict)"(reference=w810, "XScale.Range"=w815) -> ()  [unwired: 1 in, 2 out]
                  }
                  frame True {
                    n399 = property on="Property Node" class="WFChart (strict)"(reference=w823) -> (reference out=w820:refnum<vi>, "XScale.Range"=w825:T31)  [unwired: 1 in, 1 out]
                    n400 = Multiply(x=w817, y=60.0) -> (x*y=w819:dbl)
                    n401 = Bundle By Name(cluster=w825, "Minimum"=0.0, "Maximum"=w819, "Increment"=1.0) -> (w824:T31)
                    n402 = property on="Property Node" class="WFChart (strict)"(reference=w820, "XScale.Range"=w824) -> ()  [unwired: 1 in, 2 out]
                  }
                }
              }
              frame 1 {
                n403 = Not Equal To 0?(x=w826) -> (x != 0?=w827:bool)
                n404 = case shown="True" w827 {
                  tunnel: w828 -> [w830 w840]
                  tunnel: w826 -> [_ w837]
                  frame False {
                    n405 = property on="Property Node" class="WFChart (strict)"(reference=w830) -> (reference out=w829:refnum<vi>, "XScale.Range"=w835:T31)  [unwired: 1 in, 1 out]
                    n406 = Bundle By Name(cluster=w835, "Minimum"=0.0, "Maximum"=43200.0, "Increment"=3600.0) -> (w831:T31)
                    n407 = property on="Property Node" class="WFChart (strict)"(reference=w829, "XScale.Range"=w831) -> ()  [unwired: 1 in, 2 out]
                  }
                  frame True {
                    n408 = Multiply(x=w837, y=3600.0) -> (x*y=w836:dbl)
                    n409 = property on="Property Node" class="WFChart (strict)"(reference=w840) -> (reference out=w839:refnum<vi>, "XScale.Range"=w844:T31)  [unwired: 1 in, 1 out]
                    n410 = Bundle By Name(cluster=w844, "Minimum"=0.0, "Maximum"=w836, "Increment"=3600.0) -> (w841:T31)
                    n411 = property on="Property Node" class="WFChart (strict)"(reference=w839, "XScale.Range"=w841) -> ()  [unwired: 1 in, 2 out]
                  }
                }
              }
              frame 2 {
                n412 = Not Equal To 0?(x=w845) -> (x != 0?=w846:bool)
                n413 = case shown="True" w846 {
                  tunnel: w847 -> [w849 w857]
                  tunnel: w845 -> [_ w855]
                  frame False {
                    n414 = property on="Property Node" class="WFChart (strict)"(reference=w849) -> (reference out=w848:refnum<vi>, "XScale.Range"=w854:T31)  [unwired: 1 in, 1 out]
                    n415 = Bundle By Name(cluster=w854, "Minimum"=0.0, "Maximum"=60.0, "Increment"=1.0) -> (w850:T31)
                    n416 = property on="Property Node" class="WFChart (strict)"(reference=w848, "XScale.Range"=w850) -> ()  [unwired: 1 in, 2 out]
                  }
                  frame True {
                    n417 = property on="Property Node" class="WFChart (strict)"(reference=w857) -> (reference out=w856:refnum<vi>, "XScale.Range"=w861:T31)  [unwired: 1 in, 1 out]
                    n418 = Bundle By Name(cluster=w861, "Minimum"=0.0, "Maximum"=w855, "Increment"=1.0) -> (w858:T31)
                    n419 = property on="Property Node" class="WFChart (strict)"(reference=w856, "XScale.Range"=w858) -> ()  [unwired: 1 in, 2 out]
                  }
                }
              }
            }
          }
          event "Set Time TC Graph 2": Mouse Down {
            n420 = event-data() -> ()  [unwired: 1 in, 8 out]
            n421 = local read "Log/Linear Y-Axis 2"() -> (w862:u16)
            n422 = control-ref of="Custom Chart 2"() -> (w863:refnum<vi>)
            n423 = property on="Property Node" class="WFChart (strict)"(reference=w863, "YScale.Mapping Mode"=w862) -> ()  [unwired: 1 in, 2 out]
            n424 = local read "Total Time 2"() -> (w864:dbl)
            n425 = case shown="0, Default" w862 {
              tunnel: w863 -> [w868 w870]
              frame 0, Default {
                n426 = property class="WFChart (strict)"(reference=w868, "YScale.LooseFit"=TRUE ("Y Scale.Flipped")) -> ()  [unwired: 1 in, 2 out]
              }
              frame 1 {
                n427 = property class="WFChart (strict)"(reference=w870, "YScale.LooseFit"=FALSE ("Y Scale.Flipped")) -> ()  [unwired: 1 in, 2 out]
              }
            }
            n428 = local read "Time Scale 2"() -> (w865:u16)
            n429 = case shown="2" w865 {
              tunnel: w863 -> [w874 w893 w912]
              tunnel: w864 -> [w872 w891 w910]
              frame 0, Default {
                n430 = Not Equal To 0?(x=w872) -> (x != 0?=w873:bool)
                n431 = case shown="True" w873 {
                  tunnel: w874 -> [w876 w888]
                  tunnel: w872 -> [_ w882]
                  frame False {
                    n432 = property on="Property Node" class="WFChart (strict)"(reference=w876) -> (reference out=w875:refnum<vi>, "XScale.Range"=w881:T31)  [unwired: 1 in, 1 out]
                    n433 = Bundle By Name(cluster=w881, "Minimum"=0.0, "Maximum"=3600.0, "Increment"=60.0) -> (w880:T31)
                    n434 = property on="Property Node" class="WFChart (strict)"(reference=w875, "XScale.Range"=w880) -> ()  [unwired: 1 in, 2 out]
                  }
                  frame True {
                    n435 = property on="Property Node" class="WFChart (strict)"(reference=w888) -> (reference out=w885:refnum<vi>, "XScale.Range"=w890:T31)  [unwired: 1 in, 1 out]
                    n436 = Multiply(x=w882, y=60.0) -> (x*y=w884:dbl)
                    n437 = Bundle By Name(cluster=w890, "Minimum"=0.0, "Maximum"=w884, "Increment"=1.0) -> (w889:T31)
                    n438 = property on="Property Node" class="WFChart (strict)"(reference=w885, "XScale.Range"=w889) -> ()  [unwired: 1 in, 2 out]
                  }
                }
              }
              frame 1 {
                n439 = Not Equal To 0?(x=w891) -> (x != 0?=w892:bool)
                n440 = case shown="True" w892 {
                  tunnel: w893 -> [w895 w905]
                  tunnel: w891 -> [_ w902]
                  frame False {
                    n441 = property on="Property Node" class="WFChart (strict)"(reference=w895) -> (reference out=w894:refnum<vi>, "XScale.Range"=w900:T31)  [unwired: 1 in, 1 out]
                    n442 = Bundle By Name(cluster=w900, "Minimum"=0.0, "Maximum"=43200.0, "Increment"=3600.0) -> (w896:T31)
                    n443 = property on="Property Node" class="WFChart (strict)"(reference=w894, "XScale.Range"=w896) -> ()  [unwired: 1 in, 2 out]
                  }
                  frame True {
                    n444 = Multiply(x=w902, y=3600.0) -> (x*y=w901:dbl)
                    n445 = property on="Property Node" class="WFChart (strict)"(reference=w905) -> (reference out=w904:refnum<vi>, "XScale.Range"=w909:T31)  [unwired: 1 in, 1 out]
                    n446 = Bundle By Name(cluster=w909, "Minimum"=0.0, "Maximum"=w901, "Increment"=3600.0) -> (w906:T31)
                    n447 = property on="Property Node" class="WFChart (strict)"(reference=w904, "XScale.Range"=w906) -> ()  [unwired: 1 in, 2 out]
                  }
                }
              }
              frame 2 {
                n448 = Not Equal To 0?(x=w910) -> (x != 0?=w911:bool)
                n449 = case shown="True" w911 {
                  tunnel: w912 -> [w914 w922]
                  tunnel: w910 -> [_ w920]
                  frame False {
                    n450 = property on="Property Node" class="WFChart (strict)"(reference=w914) -> (reference out=w913:refnum<vi>, "XScale.Range"=w919:T31)  [unwired: 1 in, 1 out]
                    n451 = Bundle By Name(cluster=w919, "Minimum"=0.0, "Maximum"=60.0, "Increment"=1.0) -> (w915:T31)
                    n452 = property on="Property Node" class="WFChart (strict)"(reference=w913, "XScale.Range"=w915) -> ()  [unwired: 1 in, 2 out]
                  }
                  frame True {
                    n453 = property on="Property Node" class="WFChart (strict)"(reference=w922) -> (reference out=w921:refnum<vi>, "XScale.Range"=w926:T31)  [unwired: 1 in, 1 out]
                    n454 = Bundle By Name(cluster=w926, "Minimum"=0.0, "Maximum"=w920, "Increment"=1.0) -> (w923:T31)
                    n455 = property on="Property Node" class="WFChart (strict)"(reference=w921, "XScale.Range"=w923) -> ()  [unwired: 1 in, 2 out]
                  }
                }
              }
            }
          }
          event "Set Time TC Graph 3": Mouse Down {
            n456 = event-data() -> ()  [unwired: 1 in, 8 out]
            n457 = local read "Log/Linear Y-Axis 3"() -> (w927:u16)
            n458 = control-ref of="Custom Chart 3"() -> (w928:refnum<vi>)
            n459 = property on="Property Node" class="WFChart (strict)"(reference=w928, "YScale.Mapping Mode"=w927) -> ()  [unwired: 1 in, 2 out]
            n460 = local read "Total Time 3"() -> (w929:dbl)
            n461 = case shown="0, Default" w927 {
              tunnel: w928 -> [w933 w935]
              frame 0, Default {
                n462 = property class="WFChart (strict)"(reference=w933, "YScale.LooseFit"=TRUE ("Y Scale.Flipped")) -> ()  [unwired: 1 in, 2 out]
              }
              frame 1 {
                n463 = property class="WFChart (strict)"(reference=w935, "YScale.LooseFit"=FALSE ("Y Scale.Flipped")) -> ()  [unwired: 1 in, 2 out]
              }
            }
            n464 = local read "Time Scale 3"() -> (w930:u16)
            n465 = case shown="2" w930 {
              tunnel: w928 -> [w939 w958 w977]
              tunnel: w929 -> [w937 w956 w975]
              frame 0, Default {
                n466 = Not Equal To 0?(x=w937) -> (x != 0?=w938:bool)
                n467 = case shown="True" w938 {
                  tunnel: w939 -> [w941 w953]
                  tunnel: w937 -> [_ w947]
                  frame False {
                    n468 = property on="Property Node" class="WFChart (strict)"(reference=w941) -> (reference out=w940:refnum<vi>, "XScale.Range"=w946:T31)  [unwired: 1 in, 1 out]
                    n469 = Bundle By Name(cluster=w946, "Minimum"=0.0, "Maximum"=3600.0, "Increment"=60.0) -> (w945:T31)
                    n470 = property on="Property Node" class="WFChart (strict)"(reference=w940, "XScale.Range"=w945) -> ()  [unwired: 1 in, 2 out]
                  }
                  frame True {
                    n471 = property on="Property Node" class="WFChart (strict)"(reference=w953) -> (reference out=w950:refnum<vi>, "XScale.Range"=w955:T31)  [unwired: 1 in, 1 out]
                    n472 = Multiply(x=w947, y=60.0) -> (x*y=w949:dbl)
                    n473 = Bundle By Name(cluster=w955, "Minimum"=0.0, "Maximum"=w949, "Increment"=1.0) -> (w954:T31)
                    n474 = property on="Property Node" class="WFChart (strict)"(reference=w950, "XScale.Range"=w954) -> ()  [unwired: 1 in, 2 out]
                  }
                }
              }
              frame 1 {
                n475 = Not Equal To 0?(x=w956) -> (x != 0?=w957:bool)
                n476 = case shown="True" w957 {
                  tunnel: w958 -> [w960 w970]
                  tunnel: w956 -> [_ w967]
                  frame False {
                    n477 = property on="Property Node" class="WFChart (strict)"(reference=w960) -> (reference out=w959:refnum<vi>, "XScale.Range"=w965:T31)  [unwired: 1 in, 1 out]
                    n478 = Bundle By Name(cluster=w965, "Minimum"=0.0, "Maximum"=43200.0, "Increment"=3600.0) -> (w961:T31)
                    n479 = property on="Property Node" class="WFChart (strict)"(reference=w959, "XScale.Range"=w961) -> ()  [unwired: 1 in, 2 out]
                  }
                  frame True {
                    n480 = Multiply(x=w967, y=3600.0) -> (x*y=w966:dbl)
                    n481 = property on="Property Node" class="WFChart (strict)"(reference=w970) -> (reference out=w969:refnum<vi>, "XScale.Range"=w974:T31)  [unwired: 1 in, 1 out]
                    n482 = Bundle By Name(cluster=w974, "Minimum"=0.0, "Maximum"=w966, "Increment"=3600.0) -> (w971:T31)
                    n483 = property on="Property Node" class="WFChart (strict)"(reference=w969, "XScale.Range"=w971) -> ()  [unwired: 1 in, 2 out]
                  }
                }
              }
              frame 2 {
                n484 = Not Equal To 0?(x=w975) -> (x != 0?=w976:bool)
                n485 = case shown="True" w976 {
                  tunnel: w977 -> [w979 w987]
                  tunnel: w975 -> [_ w985]
                  frame False {
                    n486 = property on="Property Node" class="WFChart (strict)"(reference=w979) -> (reference out=w978:refnum<vi>, "XScale.Range"=w984:T31)  [unwired: 1 in, 1 out]
                    n487 = Bundle By Name(cluster=w984, "Minimum"=0.0, "Maximum"=60.0, "Increment"=1.0) -> (w980:T31)
                    n488 = property on="Property Node" class="WFChart (strict)"(reference=w978, "XScale.Range"=w980) -> ()  [unwired: 1 in, 2 out]
                  }
                  frame True {
                    n489 = property on="Property Node" class="WFChart (strict)"(reference=w987) -> (reference out=w986:refnum<vi>, "XScale.Range"=w991:T31)  [unwired: 1 in, 1 out]
                    n490 = Bundle By Name(cluster=w991, "Minimum"=0.0, "Maximum"=w985, "Increment"=1.0) -> (w988:T31)
                    n491 = property on="Property Node" class="WFChart (strict)"(reference=w986, "XScale.Range"=w988) -> ()  [unwired: 1 in, 2 out]
                  }
                }
              }
            }
          }
          event "Set Time TC Graph 4": Mouse Down {
            n492 = event-data() -> ()  [unwired: 1 in, 8 out]
            n493 = local read "Log/Linear Y-Axis 4"() -> (w992:u16)
            n494 = control-ref of="Custom Chart 4"() -> (w993:refnum<vi>)
            n495 = property on="Property Node" class="WFChart (strict)"(reference=w993, "YScale.Mapping Mode"=w992) -> ()  [unwired: 1 in, 2 out]
            n496 = local read "Total Time 4"() -> (w994:dbl)
            n497 = case shown="0, Default" w992 {
              tunnel: w993 -> [w998 w1000]
              frame 0, Default {
                n498 = property class="WFChart (strict)"(reference=w998, "YScale.LooseFit"=TRUE ("Y Scale.Flipped")) -> ()  [unwired: 1 in, 2 out]
              }
              frame 1 {
                n499 = property class="WFChart (strict)"(reference=w1000, "YScale.LooseFit"=FALSE ("Y Scale.Flipped")) -> ()  [unwired: 1 in, 2 out]
              }
            }
            n500 = local read "Time Scale 4"() -> (w995:u16)
            n501 = case shown="2" w995 {
              tunnel: w993 -> [w1004 w1023 w1042]
              tunnel: w994 -> [w1002 w1021 w1040]
              frame 0, Default {
                n502 = Not Equal To 0?(x=w1002) -> (x != 0?=w1003:bool)
                n503 = case shown="True" w1003 {
                  tunnel: w1004 -> [w1006 w1018]
                  tunnel: w1002 -> [_ w1012]
                  frame False {
                    n504 = property on="Property Node" class="WFChart (strict)"(reference=w1006) -> (reference out=w1005:refnum<vi>, "XScale.Range"=w1011:T31)  [unwired: 1 in, 1 out]
                    n505 = Bundle By Name(cluster=w1011, "Minimum"=0.0, "Maximum"=3600.0, "Increment"=60.0) -> (w1010:T31)
                    n506 = property on="Property Node" class="WFChart (strict)"(reference=w1005, "XScale.Range"=w1010) -> ()  [unwired: 1 in, 2 out]
                  }
                  frame True {
                    n507 = property on="Property Node" class="WFChart (strict)"(reference=w1018) -> (reference out=w1015:refnum<vi>, "XScale.Range"=w1020:T31)  [unwired: 1 in, 1 out]
                    n508 = Multiply(x=w1012, y=60.0) -> (x*y=w1014:dbl)
                    n509 = Bundle By Name(cluster=w1020, "Minimum"=0.0, "Maximum"=w1014, "Increment"=1.0) -> (w1019:T31)
                    n510 = property on="Property Node" class="WFChart (strict)"(reference=w1015, "XScale.Range"=w1019) -> ()  [unwired: 1 in, 2 out]
                  }
                }
              }
              frame 1 {
                n511 = Not Equal To 0?(x=w1021) -> (x != 0?=w1022:bool)
                n512 = case shown="True" w1022 {
                  tunnel: w1023 -> [w1025 w1035]
                  tunnel: w1021 -> [_ w1032]
                  frame False {
                    n513 = property on="Property Node" class="WFChart (strict)"(reference=w1025) -> (reference out=w1024:refnum<vi>, "XScale.Range"=w1030:T31)  [unwired: 1 in, 1 out]
                    n514 = Bundle By Name(cluster=w1030, "Minimum"=0.0, "Maximum"=43200.0, "Increment"=3600.0) -> (w1026:T31)
                    n515 = property on="Property Node" class="WFChart (strict)"(reference=w1024, "XScale.Range"=w1026) -> ()  [unwired: 1 in, 2 out]
                  }
                  frame True {
                    n516 = Multiply(x=w1032, y=3600.0) -> (x*y=w1031:dbl)
                    n517 = property on="Property Node" class="WFChart (strict)"(reference=w1035) -> (reference out=w1034:refnum<vi>, "XScale.Range"=w1039:T31)  [unwired: 1 in, 1 out]
                    n518 = Bundle By Name(cluster=w1039, "Minimum"=0.0, "Maximum"=w1031, "Increment"=3600.0) -> (w1036:T31)
                    n519 = property on="Property Node" class="WFChart (strict)"(reference=w1034, "XScale.Range"=w1036) -> ()  [unwired: 1 in, 2 out]
                  }
                }
              }
              frame 2 {
                n520 = Not Equal To 0?(x=w1040) -> (x != 0?=w1041:bool)
                n521 = case shown="True" w1041 {
                  tunnel: w1042 -> [w1044 w1052]
                  tunnel: w1040 -> [_ w1050]
                  frame False {
                    n522 = property on="Property Node" class="WFChart (strict)"(reference=w1044) -> (reference out=w1043:refnum<vi>, "XScale.Range"=w1049:T31)  [unwired: 1 in, 1 out]
                    n523 = Bundle By Name(cluster=w1049, "Minimum"=0.0, "Maximum"=60.0, "Increment"=1.0) -> (w1045:T31)
                    n524 = property on="Property Node" class="WFChart (strict)"(reference=w1043, "XScale.Range"=w1045) -> ()  [unwired: 1 in, 2 out]
                  }
                  frame True {
                    n525 = property on="Property Node" class="WFChart (strict)"(reference=w1052) -> (reference out=w1051:refnum<vi>, "XScale.Range"=w1056:T31)  [unwired: 1 in, 1 out]
                    n526 = Bundle By Name(cluster=w1056, "Minimum"=0.0, "Maximum"=w1050, "Increment"=1.0) -> (w1053:T31)
                    n527 = property on="Property Node" class="WFChart (strict)"(reference=w1051, "XScale.Range"=w1053) -> ()  [unwired: 1 in, 2 out]
                  }
                }
              }
            }
          }
          event "Set Time TC Graph 5": Mouse Down {
            n528 = event-data() -> ()  [unwired: 1 in, 8 out]
            n529 = local read "Log/Linear Y-Axis 5"() -> (w1057:u16)
            n530 = control-ref of="Custom Chart 5"() -> (w1058:refnum<vi>)
            n531 = property on="Property Node" class="WFChart (strict)"(reference=w1058, "YScale.Mapping Mode"=w1057) -> ()  [unwired: 1 in, 2 out]
            n532 = case shown="0, Default" w1057 {
              tunnel: w1058 -> [w1063 w1065]
              frame 0, Default {
                n533 = property class="WFChart (strict)"(reference=w1063, "YScale.LooseFit"=TRUE ("Y Scale.Flipped")) -> ()  [unwired: 1 in, 2 out]
              }
              frame 1 {
                n534 = property class="WFChart (strict)"(reference=w1065, "YScale.LooseFit"=FALSE ("Y Scale.Flipped")) -> ()  [unwired: 1 in, 2 out]
              }
            }
            n535 = local read "Total Time 5"() -> (w1059:dbl)
            n536 = local read "Time Scale 5"() -> (w1060:u16)
            n537 = case shown="2" w1060 {
              tunnel: w1058 -> [w1069 w1088 w1107]
              tunnel: w1059 -> [w1067 w1086 w1105]
              frame 0, Default {
                n538 = Not Equal To 0?(x=w1067) -> (x != 0?=w1068:bool)
                n539 = case shown="True" w1068 {
                  tunnel: w1069 -> [w1071 w1083]
                  tunnel: w1067 -> [_ w1077]
                  frame False {
                    n540 = property on="Property Node" class="WFChart (strict)"(reference=w1071) -> (reference out=w1070:refnum<vi>, "XScale.Range"=w1076:T31)  [unwired: 1 in, 1 out]
                    n541 = Bundle By Name(cluster=w1076, "Minimum"=0.0, "Maximum"=3600.0, "Increment"=60.0) -> (w1075:T31)
                    n542 = property on="Property Node" class="WFChart (strict)"(reference=w1070, "XScale.Range"=w1075) -> ()  [unwired: 1 in, 2 out]
                  }
                  frame True {
                    n543 = property on="Property Node" class="WFChart (strict)"(reference=w1083) -> (reference out=w1080:refnum<vi>, "XScale.Range"=w1085:T31)  [unwired: 1 in, 1 out]
                    n544 = Multiply(x=w1077, y=60.0) -> (x*y=w1079:dbl)
                    n545 = Bundle By Name(cluster=w1085, "Minimum"=0.0, "Maximum"=w1079, "Increment"=1.0) -> (w1084:T31)
                    n546 = property on="Property Node" class="WFChart (strict)"(reference=w1080, "XScale.Range"=w1084) -> ()  [unwired: 1 in, 2 out]
                  }
                }
              }
              frame 1 {
                n547 = Not Equal To 0?(x=w1086) -> (x != 0?=w1087:bool)
                n548 = case shown="True" w1087 {
                  tunnel: w1088 -> [w1090 w1100]
                  tunnel: w1086 -> [_ w1097]
                  frame False {
                    n549 = property on="Property Node" class="WFChart (strict)"(reference=w1090) -> (reference out=w1089:refnum<vi>, "XScale.Range"=w1095:T31)  [unwired: 1 in, 1 out]
                    n550 = Bundle By Name(cluster=w1095, "Minimum"=0.0, "Maximum"=43200.0, "Increment"=3600.0) -> (w1091:T31)
                    n551 = property on="Property Node" class="WFChart (strict)"(reference=w1089, "XScale.Range"=w1091) -> ()  [unwired: 1 in, 2 out]
                  }
                  frame True {
                    n552 = Multiply(x=w1097, y=3600.0) -> (x*y=w1096:dbl)
                    n553 = property on="Property Node" class="WFChart (strict)"(reference=w1100) -> (reference out=w1099:refnum<vi>, "XScale.Range"=w1104:T31)  [unwired: 1 in, 1 out]
                    n554 = Bundle By Name(cluster=w1104, "Minimum"=0.0, "Maximum"=w1096, "Increment"=3600.0) -> (w1101:T31)
                    n555 = property on="Property Node" class="WFChart (strict)"(reference=w1099, "XScale.Range"=w1101) -> ()  [unwired: 1 in, 2 out]
                  }
                }
              }
              frame 2 {
                n556 = Not Equal To 0?(x=w1105) -> (x != 0?=w1106:bool)
                n557 = case shown="True" w1106 {
                  tunnel: w1107 -> [w1109 w1117]
                  tunnel: w1105 -> [_ w1115]
                  frame False {
                    n558 = property on="Property Node" class="WFChart (strict)"(reference=w1109) -> (reference out=w1108:refnum<vi>, "XScale.Range"=w1114:T31)  [unwired: 1 in, 1 out]
                    n559 = Bundle By Name(cluster=w1114, "Minimum"=0.0, "Maximum"=60.0, "Increment"=1.0) -> (w1110:T31)
                    n560 = property on="Property Node" class="WFChart (strict)"(reference=w1108, "XScale.Range"=w1110) -> ()  [unwired: 1 in, 2 out]
                  }
                  frame True {
                    n561 = property on="Property Node" class="WFChart (strict)"(reference=w1117) -> (reference out=w1116:refnum<vi>, "XScale.Range"=w1121:T31)  [unwired: 1 in, 1 out]
                    n562 = Bundle By Name(cluster=w1121, "Minimum"=0.0, "Maximum"=w1115, "Increment"=1.0) -> (w1118:T31)
                    n563 = property on="Property Node" class="WFChart (strict)"(reference=w1116, "XScale.Range"=w1118) -> ()  [unwired: 1 in, 2 out]
                  }
                }
              }
            }
          }
          event "Set Time TC Graph 6": Mouse Down {
            n564 = event-data() -> ()  [unwired: 1 in, 8 out]
            n565 = local read "Log/Linear Y-Axis 6"() -> (w1122:u16)
            n566 = control-ref of="Custom Chart 6"() -> (w1123:refnum<vi>)
            n567 = property on="Property Node" class="WFChart (strict)"(reference=w1123, "YScale.Mapping Mode"=w1122) -> ()  [unwired: 1 in, 2 out]
            n568 = local read "Total Time 6"() -> (w1124:dbl)
            n569 = case shown="0, Default" w1122 {
              tunnel: w1123 -> [w1128 w1130]
              frame 0, Default {
                n570 = property class="WFChart (strict)"(reference=w1128, "YScale.LooseFit"=TRUE ("Y Scale.Flipped")) -> ()  [unwired: 1 in, 2 out]
              }
              frame 1 {
                n571 = property class="WFChart (strict)"(reference=w1130, "YScale.LooseFit"=FALSE ("Y Scale.Flipped")) -> ()  [unwired: 1 in, 2 out]
              }
            }
            n572 = local read "Time Scale 6"() -> (w1125:u16)
            n573 = case shown="2" w1125 {
              tunnel: w1123 -> [w1134 w1153 w1172]
              tunnel: w1124 -> [w1132 w1151 w1170]
              frame 0, Default {
                n574 = Not Equal To 0?(x=w1132) -> (x != 0?=w1133:bool)
                n575 = case shown="True" w1133 {
                  tunnel: w1134 -> [w1136 w1148]
                  tunnel: w1132 -> [_ w1142]
                  frame False {
                    n576 = property on="Property Node" class="WFChart (strict)"(reference=w1136) -> (reference out=w1135:refnum<vi>, "XScale.Range"=w1141:T31)  [unwired: 1 in, 1 out]
                    n577 = Bundle By Name(cluster=w1141, "Minimum"=0.0, "Maximum"=3600.0, "Increment"=60.0) -> (w1140:T31)
                    n578 = property on="Property Node" class="WFChart (strict)"(reference=w1135, "XScale.Range"=w1140) -> ()  [unwired: 1 in, 2 out]
                  }
                  frame True {
                    n579 = property on="Property Node" class="WFChart (strict)"(reference=w1148) -> (reference out=w1145:refnum<vi>, "XScale.Range"=w1150:T31)  [unwired: 1 in, 1 out]
                    n580 = Multiply(x=w1142, y=60.0) -> (x*y=w1144:dbl)
                    n581 = Bundle By Name(cluster=w1150, "Minimum"=0.0, "Maximum"=w1144, "Increment"=1.0) -> (w1149:T31)
                    n582 = property on="Property Node" class="WFChart (strict)"(reference=w1145, "XScale.Range"=w1149) -> ()  [unwired: 1 in, 2 out]
                  }
                }
              }
              frame 1 {
                n583 = Not Equal To 0?(x=w1151) -> (x != 0?=w1152:bool)
                n584 = case shown="True" w1152 {
                  tunnel: w1153 -> [w1155 w1165]
                  tunnel: w1151 -> [_ w1162]
                  frame False {
                    n585 = property on="Property Node" class="WFChart (strict)"(reference=w1155) -> (reference out=w1154:refnum<vi>, "XScale.Range"=w1160:T31)  [unwired: 1 in, 1 out]
                    n586 = Bundle By Name(cluster=w1160, "Minimum"=0.0, "Maximum"=43200.0, "Increment"=3600.0) -> (w1156:T31)
                    n587 = property on="Property Node" class="WFChart (strict)"(reference=w1154, "XScale.Range"=w1156) -> ()  [unwired: 1 in, 2 out]
                  }
                  frame True {
                    n588 = Multiply(x=w1162, y=3600.0) -> (x*y=w1161:dbl)
                    n589 = property on="Property Node" class="WFChart (strict)"(reference=w1165) -> (reference out=w1164:refnum<vi>, "XScale.Range"=w1169:T31)  [unwired: 1 in, 1 out]
                    n590 = Bundle By Name(cluster=w1169, "Minimum"=0.0, "Maximum"=w1161, "Increment"=3600.0) -> (w1166:T31)
                    n591 = property on="Property Node" class="WFChart (strict)"(reference=w1164, "XScale.Range"=w1166) -> ()  [unwired: 1 in, 2 out]
                  }
                }
              }
              frame 2 {
                n592 = Not Equal To 0?(x=w1170) -> (x != 0?=w1171:bool)
                n593 = case shown="True" w1171 {
                  tunnel: w1172 -> [w1174 w1182]
                  tunnel: w1170 -> [_ w1180]
                  frame False {
                    n594 = property on="Property Node" class="WFChart (strict)"(reference=w1174) -> (reference out=w1173:refnum<vi>, "XScale.Range"=w1179:T31)  [unwired: 1 in, 1 out]
                    n595 = Bundle By Name(cluster=w1179, "Minimum"=0.0, "Maximum"=60.0, "Increment"=1.0) -> (w1175:T31)
                    n596 = property on="Property Node" class="WFChart (strict)"(reference=w1173, "XScale.Range"=w1175) -> ()  [unwired: 1 in, 2 out]
                  }
                  frame True {
                    n597 = property on="Property Node" class="WFChart (strict)"(reference=w1182) -> (reference out=w1181:refnum<vi>, "XScale.Range"=w1186:T31)  [unwired: 1 in, 1 out]
                    n598 = Bundle By Name(cluster=w1186, "Minimum"=0.0, "Maximum"=w1180, "Increment"=1.0) -> (w1183:T31)
                    n599 = property on="Property Node" class="WFChart (strict)"(reference=w1181, "XScale.Range"=w1183) -> ()  [unwired: 1 in, 2 out]
                  }
                }
              }
            }
          }
          event "1. Compile Profile": Mouse Down {
            n600 = event-data() -> ()  [unwired: 1 in, 1 out]
            n601 = control-ref of="Number of Set points"() -> (w1195:refnum<vi>)
            n602 = property class="DigNum (strict)"(reference=w1195) -> ("Value"=w1192:dbl)  [unwired: 1 in, 2 out]
            n603 = Bundle By Name(cluster=w1194, "ZoneSetup.Number of Set points"=w1192) -> (w1193:T17)
            n604 = local write "ThermalProfileStatus"("Compiling..........." ("String")) -> ()
            n605 = call-poly "Send Message.vi"("error in (no error)"=w1187, "event buffer"="1", "event"="compileProfile") -> ("error out"=w1190:errorcluster)  [unwired: 8 in]
          }
          event "2. Save Into Database and CSV": Mouse Down {
            n606 = event-data() -> ()  [unwired: 1 in, 1 out]
            n607 = Unbundle By Name(w1200) -> ("Http session"=w1217:T16, "URL prefex"=w1213:string, "ZoneProfile.profiles"=w1212:T32, "ZoneSetup.Thermal Profile Name"=w1197:string)
            n608 = Empty String/Path?(string/path=w1197) -> (empty?=w1203:bool)
            n609 = case shown="True" w1203 {
              tunnel: w1197 -> [w1220 _]
              tunnel: [w1220 w1221] -> w1202
              tunnel: w1201 -> [w1219 w1225]
              tunnel: [w1219 w1224] -> w1198
              tunnel: w1200 -> [w1218 w1223]
              tunnel: [w1218 w1222] -> w1199
              frame False {
              }
              frame True {
                n610 = call "Prompt User for Input"("error in (no error)"=w1225) -> ("Profile Name"=w1221:string, "error out"=w1224:errorcluster)  [unwired: 16 in, 1 out]
                n611 = Bundle By Name(cluster=w1223, "ZoneSetup.Thermal Profile Name"=w1221) -> (w1222:T17)
              }
            }
            n612 = Bundle By Name(cluster=T20 {"name"="", "profiles"=[]}, "name"=w1202, "profiles"=w1212) -> (w1210:T20)
            n613 = Concatenate Strings(w1213, "saveProfile" ("url")) -> (w1216:string)
            n614 = Flatten To JSON(anything=w1210) -> (JSON string=w1215:string)  [unwired: 2 in, 1 out]
            n615 = call-poly <vilib>:"POST.vi"("client handle"=w1217, "url"=w1216, "buffer"=w1215) -> ("client handle out"=w1208:T16, "body"=w1204:string)  [unwired: 9 in, 2 out]
            n616 = Match True/False String(2:"" ("false string"), 3:"{'result':'success'}" ("true string"), 4:w1204) -> (0:w1205:bool)  [unwired: 1 out]
            n617 = Bundle By Name(cluster=w1199, "Http session"=w1208) -> (w1209:T17)
            n618 = case shown="True" w1205 {
              tunnel: w1204 -> [w1228 _]
              tunnel: w1198 -> [w1226 w1231]
              tunnel: [w1226 w1230] -> w1196
              frame False {
                n619 = Concatenate Strings("Error While Saving : " ("string"), w1228) -> (w1227:string)
                n620 = One Button Dialog(message=w1227) -> ()  [unwired: 1 in, 1 out]
              }
              frame True {
                n621 = One Button Dialog(message="Profile Saved To Database Successfully") -> ()  [unwired: 1 in, 1 out]
                n622 = call-poly "Send Message.vi"("error in (no error)"=w1231, "event"="saveProfile") -> ("error out"=w1230:errorcluster)  [unwired: 9 in]
              }
            }
          }
          event "3. Load into Memory": Mouse Down {
            n623 = event-data() -> ()  [unwired: 1 in, 1 out]
            n624 = Unbundle By Name(w1240) -> ("Http session"=w1241:T16, "URL prefex"=w1248:string, "ZoneSetup.Thermal Profile Name"=w1244:string)  [unwired: 1 out]
            n625 = Bundle By Name(cluster=cluster{"profile_name":string} {"profile_name"=""}, "profile_name"=w1244) -> (w1243:cluster{"profile_name":string})
            n626 = Flatten To JSON(anything=w1243) -> (JSON string=w1242:string)  [unwired: 2 in, 1 out]
            n627 = Concatenate Strings(w1248, "loadProfile" ("url")) -> (w1246:string)
            n628 = call-poly <vilib>:"POST.vi"("client handle"=w1241, "url"=w1246, "buffer"=w1242) -> ("client handle out"=w1238:T16, "body"=w1234:string)  [unwired: 9 in, 2 out]
            n629 = Match True/False String(2:"" ("false string"), 3:"{'result':'success'}" ("true string"), 4:w1234) -> (0:w1235:bool)  [unwired: 1 out]
            n630 = case shown="True" w1235 {
              tunnel: w1234 -> [w1251 _]
              frame False {
                n631 = Concatenate Strings("Error While Loading : " ("string"), w1251) -> (w1250:string)
                n632 = One Button Dialog(message=w1250) -> ()  [unwired: 1 in, 1 out]
              }
              frame True {
                n633 = One Button Dialog(message="Profile Loaded into Memory Successfully") -> ()  [unwired: 1 in, 1 out]
              }
            }
            n634 = Bundle By Name(cluster=w1240, "Http session"=w1238) -> (w1239:T17)
          }
          event "4. Run Profile": Mouse Down {
            n635 = event-data() -> ()  [unwired: 1 in, 1 out]
            n636 = Unbundle By Name(w1260) -> ("Http session"=w1261:T16, "URL prefex"=w1262:string)
            n637 = Concatenate Strings(w1262, "runProfile" ("url")) -> (w1263:string)
            n638 = call <vilib>:"GET.vi"("client handle"=w1261, "url"=w1263) -> ("client handle out"=w1258:T16, "body"=w1254:string)  [unwired: 10 in, 2 out]
            n639 = Match True/False String(2:"" ("false string"), 3:"{'result':'success'}" ("true string"), 4:w1254) -> (0:w1255:bool)  [unwired: 1 out]
            n640 = case shown="True" w1255 {
              tunnel: w1254 -> [w1267 _]
              frame False {
                n641 = Concatenate Strings("Error While Starting : " ("string"), w1267) -> (w1266:string)
                n642 = One Button Dialog(message=w1266) -> ()  [unwired: 1 in, 1 out]
              }
              frame True {
                n643 = One Button Dialog(message="Success: Profile is Running") -> ()  [unwired: 1 in, 1 out]
              }
            }
            n644 = Bundle By Name(cluster=w1260, "Http session"=w1258) -> (w1259:T17)
          }
          event "Rename": Value Change {
            n645 = event-data() -> ("CtlRef"=w1271:refnum<vi>, "OldVal"=w1272:bool)  [unwired: 1 in, 4 out]
            n646 = property class="Bool (strict)"(reference=w1271, "Value"=w1272) -> ()  [unwired: 1 in, 2 out]
            n647 = local read "New File Name"() -> (w1270:string)
            n648 = Bundle By Name(cluster=w1274, "ZoneSetup.Thermal Profile Name"=w1270) -> (w1273:T17)
            n649 = local write "Current Profile Name"(w1270) -> ()
          }
          event "Hold Profile": Value Change {
            n650 = event-data() -> ("NewVal"=w1276:bool)  [unwired: 1 in, 5 out]
            n651 = Unbundle By Name(w1279) -> ("Http session"=w1280:T16, "URL prefex"=w1283:string)
            n652 = case shown="True" w1276 {
              tunnel: w1283 -> [w1290 w1299]
              tunnel: w1282 -> [w1286 w1297]
              tunnel: [w1287 w1296] -> w1281
              tunnel: w1280 -> [w1289 w1295]
              tunnel: [w1288 w1294] -> w1277
              tunnel: [w1285 w1293] -> _
              tunnel: [w1284 w1292] -> _
              frame False {
                w1284 = "unHold" ("url")
                n653 = Concatenate Strings(w1290, w1284) -> (w1291:string)
                n654 = call <vilib>:"GET.vi"("client handle"=w1289, "url"=w1291, "error in (no error)"=w1286) -> ("client handle out"=w1288:T16, "body"=w1285:string, "error out"=w1287:errorcluster)  [unwired: 9 in, 1 out]
              }
              frame True {
                w1292 = "hold" ("url")
                n655 = Concatenate Strings(w1299, w1292) -> (w1298:string)
                n656 = call <vilib>:"GET.vi"("client handle"=w1295, "url"=w1298, "error in (no error)"=w1297) -> ("client handle out"=w1294:T16, "body"=w1293:string, "error out"=w1296:errorcluster)  [unwired: 9 in, 1 out]
              }
            }
            n657 = Bundle By Name(cluster=w1279, "Http session"=w1277) -> (w1278:T17)
          }
          event "Pause Profile": Value Change {
            n658 = event-data() -> ("NewVal"=w1300:bool)  [unwired: 1 in, 5 out]
            n659 = Unbundle By Name(w1303) -> ("Http session"=w1304:T16, "URL prefex"=w1307:string)
            n660 = case shown="False" w1300 {
              tunnel: w1307 -> [w1314 w1323]
              tunnel: w1306 -> [w1310 w1321]
              tunnel: [w1311 w1320] -> w1305
              tunnel: w1304 -> [w1313 w1319]
              tunnel: [w1312 w1318] -> w1301
              tunnel: [w1309 w1317] -> _
              tunnel: [w1308 w1316] -> _
              frame False {
                w1309 = "resume" ("url")
                n661 = Concatenate Strings(w1314, w1309) -> (w1315:string)
                n662 = call <vilib>:"GET.vi"("client handle"=w1313, "url"=w1315, "error in (no error)"=w1310) -> ("client handle out"=w1312:T16, "body"=w1308:string, "error out"=w1311:errorcluster)  [unwired: 9 in, 1 out]
              }
              frame True {
                w1317 = "pause" ("url")
                n663 = Concatenate Strings(w1323, w1317) -> (w1322:string)
                n664 = call <vilib>:"GET.vi"("client handle"=w1319, "url"=w1322, "error in (no error)"=w1321) -> ("client handle out"=w1318:T16, "body"=w1316:string, "error out"=w1320:errorcluster)  [unwired: 9 in, 1 out]
              }
            }
            n665 = Bundle By Name(cluster=w1303, "Http session"=w1301) -> (w1302:T17)
          }
          event "HARD STOP": Mouse Down {
            n666 = event-data() -> ()  [unwired: 1 in, 1 out]
            n667 = Unbundle By Name(w1327) -> ("Http session"=w1328:T16, "URL prefex"=w1332:string)
            n668 = Concatenate Strings(w1332, "hardStop" ("url")) -> (w1331:string)
            n669 = call <vilib>:"GET.vi"("client handle"=w1328, "url"=w1331, "error in (no error)"=w1330) -> ("client handle out"=w1325:T16, "error out"=w1329:errorcluster)  [unwired: 9 in, 2 out]
            n670 = Bundle By Name(cluster=w1327, "Http session"=w1325) -> (w1326:T17)
          }
          event "ZoneSetup.Import Profile": Value Change {
            w1355 = TRUE ("Page Visible")
            n671 = event-data() -> ("CtlRef"=w1334:refnum<vi>, "OldVal"=w1333:bool)  [unwired: 1 in, 4 out]
            n672 = control-ref of="Import CSV as a Thermal Profile"() -> (w1339:refnum<vi>)
            n673 = property class="Path"(reference=w1339) -> ("Value"=w1338:path)  [unwired: 1 in, 2 out]
            n674 = control-ref of="Thermal Profile Loader"() -> (w1365:refnum<vi>)
            n675 = property class="Bool (strict)"(reference=w1334, "Value"=w1333) -> ()  [unwired: 1 in, 2 out]
            n676 = control-ref of="Zone Selection"() -> (w1364:refnum<vi>)
            n677 = property on="Property Node" class="TabCtl (strict)"(reference=w1365) -> ("Pages"=w1358:refnum<vi>[])  [unwired: 1 in, 2 out]
            n678 = property on="Property Node" class="LstBox (strict)"(reference=w1364) -> ("Item Symbols"=w1363:i32[])  [unwired: 1 in, 2 out]
            n679 = call-poly <vilib>:"Read Delimited Spreadsheet.vi"("file path (dialog if empty)"=w1338, "delimiter (\\t)"="," ("delimiter (\\t)")) -> ("all rows"=w1348:string[][])  [unwired: 8 in, 5 out]
            n680 = Array Size(array=w1348) -> (size(s)=w1353:i32[])
            n681 = Index Array(array=w1353, index=0) -> (element=w1351:i32)
            n682 = Subtract(x=w1351, y=7) -> (x-y=w1349:i32)
            n683 = Unbundle By Name(w1346) -> ("ZonesSelected"=w1343:bool[])
            n684 = To Double Precision Float(number=w1349) -> (double precision float=w1347:dbl)
            n685 = for {
              N: 13 -> [_]
              tunnel: w1363 -> [w1482]
              tunnel: w1358 -> [w1483] mode=indexing
              shift-right: [w1475] -> w1344
              shift-left: w1343 -> [w1474]
              i -> [w1477]
              n686 = Greater?(x=w1477, y=1) -> (0:w1479:bool)
              n687 = Less?(x=w1477, y=11 ("x")) -> (x < y?=w1480:bool)
              n688 = And(x=w1480, y=w1479) -> (x .and. y?=w1478:bool)
              n689 = case shown="True" w1478 {
                tunnel: w1483 -> [_ w1494]
                tunnel: w1482 -> [_ w1491]
                tunnel: w1477 -> [_ w1490]
                tunnel: w1474 -> [w1484 w1487]
                tunnel: [w1484 w1485] -> w1475
                frame False {
                }
                frame True {
                  n690 = Subtract(x=w1490, y=2) -> (x-y=w1486:i32)
                  n691 = Index Array(array=w1491, index=w1486) -> (element=w1488:i32)
                  n692 = Equal?(x=38, y=w1488) -> (x = y?=w1492:bool)
                  n693 = case shown="False" w1492 {
                    tunnel: w1494 -> [w1499 w1504]
                    tunnel: w1487 -> [w1498 w1503]
                    tunnel: w1486 -> [w1496 w1502]
                    tunnel: [w1497 w1500] -> w1485
                    frame False {
                      w1495 = FALSE ("Page Visible")
                      n694 = property class="Page"(reference=w1499, "Page Visible"=w1495) -> ()  [unwired: 1 in, 2 out]
                      n695 = Replace Array Subset(array=w1498, new element=w1495, index=w1496) -> (w1497:bool[])
                    }
                    frame True {
                      w1501 = TRUE ("Page Visible")
                      n696 = property class="Page"(reference=w1504, "Page Visible"=w1501) -> ()  [unwired: 1 in, 2 out]
                      n697 = Replace Array Subset(array=w1503, new element=w1501, index=w1502) -> (w1500:bool[])
                    }
                  }
                }
              }
            }
            n698 = call-poly "Send Message.vi"("error in (no error)"=w1336, "event"="initThermalProfile") -> ("error out"=w1335:errorcluster)  [unwired: 9 in]
            n699 = local write "ThermalProfileStatus"("Compiling..........." ("String")) -> ()
            n700 = Bundle By Name(cluster=w1346, "ZonesSelected"=w1344) -> (w1345:T17)
            n701 = Index Array(array=w1358, index #1=11 ("index"), index #2=1 ("index")) -> (element #1=w1360:refnum<vi>, element #2=w1356:refnum<vi>)
            n702 = property class="Page"(reference=w1360, "Page Visible"=w1355) -> ()  [unwired: 1 in, 2 out]
            n703 = property class="Page"(reference=w1356, "Page Visible"=w1355) -> ()  [unwired: 1 in, 2 out]
            n704 = for {
              N: 9 -> [_]
              tunnel: w1347 -> [w1372]
              i -> [w1366]
              n705 = Initialize Array(0, w1372, 2 ("dimension size")) -> (w1371:i32[][])
              n706 = Initialize Array(0, w1372, 3 ("dimension size")) -> (w1377:i32[][])
              n707 = for {
                N: w1372 -> [_]
                shift-right: [w1472] -> w1368
                shift-left: w1377 -> [w1473]
                shift-right: [w1463] -> w1370
                shift-left: w1371 -> [w1464]
                i -> [w1461]
                w1465 = 0 ("disabled index (col)")
                w1467 = 0 ("disabled index (col)")
                n708 = Increment(x=w1461) -> (x+1=w1466:i32)
                n709 = Increment(x=w1461) -> (x+1=w1468:i32)
                n710 = Replace Array Subset(array=i32[][] [[0]], new element=w1466, index (row)=w1465, index (col)=w1465) -> (w1459:i32[][])
                n711 = Replace Array Subset(array=i32[][] [[0, 0, 0]], new element=w1468, index (row)=w1467, index (col)=w1467) -> (w1471:i32[][])
                n712 = Index Array(array=w1459, index (row)=w1465) -> (element=w1462:i32[])  [unwired: 1 in]
                n713 = Index Array(array=w1471, index (row)=w1467) -> (element=w1470:i32[])  [unwired: 1 in]
                n714 = Replace Array Subset(array=w1464, new element=w1462, index (row)=w1461) -> (w1463:i32[][])  [unwired: 1 in]
                n715 = Replace Array Subset(array=w1473, new element=w1470, index (row)=w1461) -> (w1472:i32[][])  [unwired: 1 in]
              }
              n716 = control-ref of="RampSoakTimes"() -> (w1369:refnum<vi>)
              n717 = To Double Precision Float(number=w1368) -> (double precision float=w1367:dbl[][])
              n718 = property class="Arr (strict)"(reference=w1369, "Value"=w1367) -> ()  [unwired: 1 in, 2 out]
              n719 = Number To Decimal String(number=w1370) -> ()  [unwired: 1 in, 1 out]
              n720 = case shown="8" w1366 {
                frame 0, Default {
                  n721 = control-ref of="Zone Thermocouples"() -> (w1381:refnum<vi>)
                  n722 = property class="LstBox (strict)"(reference=w1381) -> (reference out=w1379:refnum<vi>, "Item Symbols"=w1380:i32[])  [unwired: 1 in, 1 out]
                  n723 = for {
                    N: 81 -> [_]
                    shift-right: [w1383] -> w1378
                    shift-left: w1380 -> [w1385]
                    i -> [w1384]
                    n724 = Replace Array Subset(array=w1385, new element=37, index=w1384) -> (w1383:i32[])
                  }
                  n725 = property class="LstBox (strict)"(reference=w1379, "Item Symbols"=w1378) -> ()  [unwired: 1 in, 2 out]
                }
                frame 1 {
                  n726 = control-ref of="Zone Thermocouples"() -> (w1390:refnum<vi>)
                  n727 = property class="LstBox (strict)"(reference=w1390) -> (reference out=w1388:refnum<vi>, "Item Symbols"=w1389:i32[])  [unwired: 1 in, 1 out]
                  n728 = for {
                    N: 81 -> [_]
                    shift-right: [w1392] -> w1387
                    shift-left: w1389 -> [w1394]
                    i -> [w1393]
                    n729 = Replace Array Subset(array=w1394, new element=37, index=w1393) -> (w1392:i32[])
                  }
                  n730 = property class="LstBox (strict)"(reference=w1388, "Item Symbols"=w1387) -> ()  [unwired: 1 in, 2 out]
                }
                frame 2 {
                  n731 = control-ref of="Zone Thermocouples"() -> (w1399:refnum<vi>)
                  n732 = property class="LstBox (strict)"(reference=w1399) -> (reference out=w1397:refnum<vi>, "Item Symbols"=w1398:i32[])  [unwired: 1 in, 1 out]
                  n733 = for {
                    N: 81 -> [_]
                    shift-right: [w1401] -> w1396
                    shift-left: w1398 -> [w1403]
                    i -> [w1402]
                    n734 = Replace Array Subset(array=w1403, new element=37, index=w1402) -> (w1401:i32[])
                  }
                  n735 = property class="LstBox (strict)"(reference=w1397, "Item Symbols"=w1396) -> ()  [unwired: 1 in, 2 out]
                }
                frame 3 {
                  n736 = control-ref of="Zone Thermocouples"() -> (w1408:refnum<vi>)
                  n737 = property class="LstBox (strict)"(reference=w1408) -> (reference out=w1406:refnum<vi>, "Item Symbols"=w1407:i32[])  [unwired: 1 in, 1 out]
                  n738 = for {
                    N: 81 -> [_]
                    shift-right: [w1410] -> w1405
                    shift-left: w1407 -> [w1412]
                    i -> [w1411]
                    n739 = Replace Array Subset(array=w1412, new element=37, index=w1411) -> (w1410:i32[])
                  }
                  n740 = property class="LstBox (strict)"(reference=w1406, "Item Symbols"=w1405) -> ()  [unwired: 1 in, 2 out]
                }
                frame 4 {
                  n741 = control-ref of="Zone Thermocouples"() -> (w1417:refnum<vi>)
                  n742 = property class="LstBox (strict)"(reference=w1417) -> (reference out=w1415:refnum<vi>, "Item Symbols"=w1416:i32[])  [unwired: 1 in, 1 out]
                  n743 = for {
                    N: 81 -> [_]
                    shift-right: [w1419] -> w1414
                    shift-left: w1416 -> [w1421]
                    i -> [w1420]
                    n744 = Replace Array Subset(array=w1421, new element=37, index=w1420) -> (w1419:i32[])
                  }
                  n745 = property class="LstBox (strict)"(reference=w1415, "Item Symbols"=w1414) -> ()  [unwired: 1 in, 2 out]
                }
                frame 5 {
                  n746 = control-ref of="Zone Thermocouples"() -> (w1426:refnum<vi>)
                  n747 = property class="LstBox (strict)"(reference=w1426) -> (reference out=w1424:refnum<vi>, "Item Symbols"=w1425:i32[])  [unwired: 1 in, 1 out]
                  n748 = for {
                    N: 81 -> [_]
                    shift-right: [w1428] -> w1423
                    shift-left: w1425 -> [w1430]
                    i -> [w1429]
                    n749 = Replace Array Subset(array=w1430, new element=37, index=w1429) -> (w1428:i32[])
                  }
                  n750 = property class="LstBox (strict)"(reference=w1424, "Item Symbols"=w1423) -> ()  [unwired: 1 in, 2 out]
                }
                frame 6 {
                  n751 = control-ref of="Zone Thermocouples"() -> (w1435:refnum<vi>)
                  n752 = property class="LstBox (strict)"(reference=w1435) -> (reference out=w1433:refnum<vi>, "Item Symbols"=w1434:i32[])  [unwired: 1 in, 1 out]
                  n753 = for {
                    N: 81 -> [_]
                    shift-right: [w1437] -> w1432
                    shift-left: w1434 -> [w1439]
                    i -> [w1438]
                    n754 = Replace Array Subset(array=w1439, new element=37, index=w1438) -> (w1437:i32[])
                  }
                  n755 = property class="LstBox (strict)"(reference=w1433, "Item Symbols"=w1432) -> ()  [unwired: 1 in, 2 out]
                }
                frame 7 {
                  n756 = control-ref of="Zone Thermocouples"() -> (w1444:refnum<vi>)
                  n757 = property class="LstBox (strict)"(reference=w1444) -> (reference out=w1442:refnum<vi>, "Item Symbols"=w1443:i32[])  [unwired: 1 in, 1 out]
                  n758 = for {
                    N: 81 -> [_]
                    shift-right: [w1446] -> w1441
                    shift-left: w1443 -> [w1448]
                    i -> [w1447]
                    n759 = Replace Array Subset(array=w1448, new element=37, index=w1447) -> (w1446:i32[])
                  }
                  n760 = property class="LstBox (strict)"(reference=w1442, "Item Symbols"=w1441) -> ()  [unwired: 1 in, 2 out]
                }
                frame 8 {
                  n761 = control-ref of="Zone Thermocouples"() -> (w1453:refnum<vi>)
                  n762 = property class="LstBox (strict)"(reference=w1453) -> (reference out=w1451:refnum<vi>, "Item Symbols"=w1452:i32[])  [unwired: 1 in, 1 out]
                  n763 = for {
                    N: 81 -> [_]
                    shift-right: [w1455] -> w1450
                    shift-left: w1452 -> [w1457]
                    i -> [w1456]
                    n764 = Replace Array Subset(array=w1457, new element=37, index=w1456) -> (w1455:i32[])
                  }
                  n765 = property class="LstBox (strict)"(reference=w1451, "Item Symbols"=w1450) -> ()  [unwired: 1 in, 2 out]
                }
              }
            }
            n766 = call-poly "Send Message.vi"("error in (no error)"=w1335, "event"="importProfile") -> ("error out"=w1340:errorcluster)  [unwired: 9 in]
          }
          event "ZoneSetup.LoadFromDatabase": Value Change {
            n767 = event-data() -> ("CtlRef"=w1511:refnum<vi>, "OldVal"=w1510:bool)  [unwired: 1 in, 4 out]
            n768 = local read "TVAC Labview"() -> (w1518:bool)
            n769 = property class="Bool (strict)"(reference=w1511, "Value"=w1510) -> ()  [unwired: 1 in, 2 out]
            n770 = control-ref of="Saved Database Profiles"() -> (w1524:refnum<vi>)
            n771 = property class="Ring (strict)" props=["Value"](reference=w1524, error in=w1515) -> (reference out=w1523:refnum<vi>, error out=w1517:errorcluster)  [unwired: 1 out]
            n772 = case shown="True" w1518 {
              tunnel: ["C:\\Users\\stefan\\Documents\\GitHub\\TVAC\\head\\Labview2017\\TVAC_GUI\\DatabaseCSV\\" "C:\\Users\\TVAC-admin\\Documents\\TVAC_Github\\head\\Labview2017\\TVAC_GUI\\DatabaseCSV\\" ("file path (use dialog)")] -> w1522
              frame False {
              }
              frame True {
              }
            }
            n773 = property class="Ring (strict)"(reference=w1523, error in=w1517) -> (error out=w1516:errorcluster, "RingText.Text"=w1521:string)  [unwired: 1 out]
            n774 = Concatenate Strings(w1522, w1521, ".csv" ("string")) -> (w1519:string)
            n775 = String To Path(string=w1519) -> (path=w1506:path)
            n776 = control-ref of="Import CSV as a Thermal Profile"() -> (w1525:refnum<vi>)
            n777 = property class="Path"(reference=w1525, error in=w1516, "Value"=w1506) -> (error out=w1507:errorcluster)  [unwired: 1 out]
            n778 = call <vilib>:"Simple Error Handler.vi"("error in (no error)"=w1507) -> ("error?"=w1508:bool, "error out"=w1509:errorcluster)  [unwired: 4 in, 3 out]
            n779 = call-poly <vilib>:"Read Delimited Spreadsheet.vi"("file path (dialog if empty)"=w1506) -> ("all rows"=w1505:string[][])  [unwired: 9 in, 5 out]
            n780 = case shown="False" w1508 {
              tunnel: [w1547 w1587] -> w1514
              tunnel: w1513 -> [w1540 w1588]
              tunnel: [w1539 w1588] -> w1512
              tunnel: w1509 -> [w1530 w1587]
              tunnel: w1505 -> [w1526 _]
              frame False {
                w1546 = TRUE ("Page Visible")
                (unwired) 13
                n781 = control-ref of="Thermal Profile Loader"() -> (w1554:refnum<vi>)
                n782 = control-ref of="Zone Selection"() -> (w1553:refnum<vi>)
                n783 = property on="Property Node" class="TabCtl (strict)"(reference=w1554) -> ("Pages"=w1543:refnum<vi>[])  [unwired: 1 in, 2 out]
                n784 = property class="LstBox (strict)"(reference=w1553) -> ("Value"=w1537:i32[])  [unwired: 1 in, 2 out]
                n785 = Index Array(array=w1526, index (row)=1, index (col)=0 ("disabled index (col)")) -> (element=w1533:string)
                n786 = Unbundle By Name(w1540) -> ("ZonesSelected"=w1541:bool[])
                n787 = Spreadsheet String To Array(delimiter (Tab)=",", format string="%s", spreadsheet string=w1533, array type (2D Dbl)=string[] []) -> (array=w1531:string[])
                n788 = call-poly "Send Message.vi"("error in (no error)"=w1530, "event"="initThermalProfile") -> ("error out"=w1529:errorcluster)  [unwired: 9 in]
                n789 = for {
                  N: 9 -> [_]
                  tunnel: w1531 -> [w1557]
                  shift-right: [w1562] -> w1538
                  shift-left: w1541 -> [w1561]
                  shift-right: [w1559] -> _
                  shift-left: w1537 -> [w1560]
                  shift-right: [w1558] -> _
                  shift-left: w1543 -> [w1563]
                  i -> [w1555]
                  n790 = Index Array(array=w1557, index=w1555) -> (element=w1556:string)
                  n791 = Empty String/Path?(string/path=w1556) -> (empty?=w1564:bool)
                  n792 = case shown="True" w1564 {
                    tunnel: w1563 -> [w1565 w1576]
                    tunnel: w1555 -> [w1567 w1578]
                    tunnel: w1561 -> [w1571 w1583]
                    tunnel: [w1570 w1582] -> w1562
                    tunnel: w1560 -> [w1569 w1580]
                    tunnel: [w1568 w1579] -> w1559
                    tunnel: [w1565 w1576] -> w1558
                    frame False {
                      w1572 = TRUE ("Page Visible")
                      n793 = Add(x=2, y=w1567) -> (x+y=w1575:i32)
                      n794 = Index Array(array=w1565, index=w1575) -> (element=w1573:refnum<vi>)
                      n795 = property class="Page"(reference=w1573, "Page Visible"=w1572) -> ()  [unwired: 1 in, 2 out]
                      n796 = Replace Array Subset(array=w1571, new element=w1572, index=w1567) -> (w1570:bool[])
                      n797 = Replace Array Subset(array=w1569, new element=38, index=w1567) -> (w1568:i32[])
                    }
                    frame True {
                      w1581 = FALSE ("Page Visible")
                      n798 = Add(x=2, y=w1578) -> (x+y=w1586:i32)
                      n799 = Index Array(array=w1576, index=w1586) -> (element=w1584:refnum<vi>)
                      n800 = property class="Page"(reference=w1584, "Page Visible"=w1581) -> ()  [unwired: 1 in, 2 out]
                      n801 = Replace Array Subset(array=w1583, new element=w1581, index=w1578) -> (w1582:bool[])
                      n802 = Replace Array Subset(array=w1580, new element=37, index=w1578) -> (w1579:i32[])
                    }
                  }
                }
                n803 = call-poly "Send Message.vi"("error in (no error)"=w1529, "event"="importProfile") -> ("error out"=w1542:errorcluster)  [unwired: 9 in]
                n804 = Bundle By Name(cluster=w1540, "ZonesSelected"=w1538) -> (w1539:T17)
                n805 = Index Array(array=w1543, index #1=11 ("index"), index #2=1 ("index")) -> (element #1=w1550:refnum<vi>, element #2=w1549:refnum<vi>)
                n806 = property class="Page"(reference=w1549, error in=w1542, "Page Visible"=w1546) -> (error out=w1548:errorcluster)  [unwired: 1 out]
                n807 = property class="Page"(reference=w1550, error in=w1548, "Page Visible"=w1546) -> (error out=w1547:errorcluster)  [unwired: 1 out]
              }
              frame True {
              }
            }
          }
          event "Current Errors (click to clear)": Mouse Down {
            n808 = event-data() -> ("CtlRef"=w1598:refnum<vi>, "Coords"=w1597:T30)  [unwired: 1 in]
            n809 = invoke on="Invoke Node" class="MCListbox (strict)" method="Point To Row Column"(reference=w1598, "Point"=w1597) -> (reference out=w1594:refnum<vi>, "InBounds"=w1591:bool, "CellPosition"=w1595:T33)  [unwired: 5 in, 4 out]
            n810 = case shown="True" w1591 {
              tunnel: w1595 -> [_ w1611]
              tunnel: w1594 -> [_ w1610]
              tunnel: w1593 -> [w1599 w1609]
              tunnel: [w1599 w1608] -> w1592
              frame False {
              }
              frame True {
                n811 = Unbundle By Name(w1611) -> ("Row"=w1604:i32)
                n812 = property on="Property Node" class="MCListbox (strict)"(reference=w1610, "ActiveCell"=w1611) -> (reference out=w1606:refnum<vi>)  [unwired: 1 in, 1 out]
                n813 = Unbundle By Name(w1609) -> ("ErrorArray"=w1605:string[][], "PrevErrorArray"=w1607:string[][])
                n814 = Index Array(array=w1605, index (row)=w1604, index (col)=1 ("disabled index (col)")) -> (element=w1600:string)
                n815 = Equal?(x=w1600, y="") -> (x = y?=w1602:bool)
                n816 = case shown="False" w1602 {
                  tunnel: w1609 -> [w1621 w1622]
                  tunnel: [w1620 w1622] -> w1608
                  tunnel: w1607 -> [w1619 _]
                  tunnel: w1606 -> [w1617 _]
                  tunnel: w1605 -> [w1613 _]
                  tunnel: w1604 -> [w1612 _]
                  frame False {
                    n817 = control-ref of="Error History"() -> (w1616:refnum<vi>)
                    n818 = Delete From Array(array=w1613, index (row)=w1612) -> (deleted portion=w1618:string[], array with subset deleted=w1614:string[][])  [unwired: 2 in]
                    n819 = Build Array (concatenate)(w1618, w1619) -> (w1615:string[][])
                    n820 = property on="Property Node" class="MCListbox (strict)"(reference=w1617, "ItemNames"=w1614) -> ()  [unwired: 1 in, 2 out]
                    n821 = property on="Property Node" class="MCListbox (strict)"(reference=w1616, "ItemNames"=w1615) -> ()  [unwired: 1 in, 2 out]
                    n822 = Bundle By Name(cluster=w1621, "ErrorArray"=w1614, "PrevErrorArray"=w1615) -> (w1620:T17)
                  }
                  frame True {
                  }
                }
              }
            }
          }
          event "Current Events (click to clear)": Mouse Down {
            n823 = event-data() -> ("CtlRef"=w1630:refnum<vi>, "Coords"=w1629:T30)  [unwired: 1 in]
            n824 = invoke on="Invoke Node" class="MCListbox (strict)" method="Point To Row Column"(reference=w1630, "Point"=w1629) -> (reference out=w1626:refnum<vi>, "InBounds"=w1623:bool, "CellPosition"=w1627:T33)  [unwired: 5 in, 4 out]
            n825 = case shown="True" w1623 {
              tunnel: w1627 -> [_ w1643]
              tunnel: w1626 -> [_ w1642]
              tunnel: w1625 -> [w1631 w1641]
              tunnel: [w1631 w1640] -> w1624
              frame False {
              }
              frame True {
                n826 = Unbundle By Name(w1643) -> ("Row"=w1636:i32)
                n827 = property on="Property Node" class="MCListbox (strict)"(reference=w1642, "ActiveCell"=w1643) -> (reference out=w1638:refnum<vi>)  [unwired: 1 in, 1 out]
                n828 = Unbundle By Name(w1641) -> ("EventArray"=w1637:string[][], "PrevEventArray"=w1639:string[][])
                n829 = Index Array(array=w1637, index (row)=w1636, index (col)=1 ("disabled index (col)")) -> (element=w1632:string)
                n830 = Equal?(x=w1632, y="") -> (x = y?=w1634:bool)
                n831 = case shown="False" w1634 {
                  tunnel: w1641 -> [w1653 w1654]
                  tunnel: [w1652 w1654] -> w1640
                  tunnel: w1639 -> [w1651 _]
                  tunnel: w1638 -> [w1649 _]
                  tunnel: w1637 -> [w1645 _]
                  tunnel: w1636 -> [w1644 _]
                  frame False {
                    n832 = control-ref of="Event History"() -> (w1648:refnum<vi>)
                    n833 = Delete From Array(array=w1645, index (row)=w1644) -> (deleted portion=w1650:string[], array with subset deleted=w1646:string[][])  [unwired: 2 in]
                    n834 = Build Array (concatenate)(w1650, w1651) -> (w1647:string[][])
                    n835 = property on="Property Node" class="MCListbox (strict)"(reference=w1649, "ItemNames"=w1646) -> ()  [unwired: 1 in, 2 out]
                    n836 = property on="Property Node" class="MCListbox (strict)"(reference=w1648, "ItemNames"=w1647) -> ()  [unwired: 1 in, 2 out]
                    n837 = Bundle By Name(cluster=w1653, "EventArray"=w1646, "PrevEventArray"=w1647) -> (w1652:T17)
                  }
                  frame True {
                  }
                }
              }
            }
          }
          event "Clear All Errors": Mouse Down {
            w1659 = 0 ("index")
            n838 = event-data() -> ()  [unwired: 1 in, 5 out]
            n839 = Unbundle By Name(w1672) -> ("ErrorArray"=w1658:string[][], "PrevErrorArray"=w1670:string[][])
            n840 = Array Size(array=w1658) -> (size(s)=w1668:i32[])
            n841 = Index Array(array=w1668, index #1=w1659, index #2=1 ("index")) -> (element #1=w1666:i32)  [unwired: 1 out]
            n842 = Index Array(array=w1658, index (col)=1 ("disabled index (col)")) -> (element=w1661:string[])  [unwired: 1 in]
            n843 = Array Size(array=w1658) -> (size(s)=w1657:i32[])
            n844 = Initialize Array(0, w1666) -> (w1664:i32[])
            n845 = Index Array(array=w1661, index=w1659) -> (element=w1660:string)
            n846 = Index Array(array=w1657, index=0) -> (element=w1655:i32)
            n847 = Not Equal?(x=w1660, y="") -> (x != y?=w1663:bool)
            n848 = case shown="True" w1663 {
              tunnel: w1672 -> [w1674 w1685]
              tunnel: [w1674 w1684] -> w1671
              tunnel: w1670 -> [_ w1683]
              tunnel: w1658 -> [_ w1679]
              tunnel: w1664 -> [_ w1682]
              tunnel: w1655 -> [_ w1676]
              frame False {
              }
              frame True {
                w1675 = string[][] [] ("Item Names")
                n849 = for {
                  N: w1676 -> [_]
                  shift-right: [w1691] -> w1677
                  shift-left: w1683 -> [w1692]
                  shift-right: [w1690] -> w1680
                  shift-left: w1682 -> [w1690]
                  tunnel: w1679 -> [w1686] mode=indexing
                  n850 = Index Array(array=w1686, index=1) -> (element=w1687:string)
                  n851 = Empty String/Path?(string/path=w1687) -> (empty?=w1689:bool)
                  n852 = case shown="False" w1689 {
                    tunnel: w1692 -> [w1695 w1696]
                    tunnel: [w1694 w1696] -> w1691
                    tunnel: w1686 -> [w1693 _]
                    frame False {
                      n853 = Build Array (concatenate)(w1693, w1695) -> (w1694:string[][])
                    }
                    frame True {
                    }
                  }
                }
                n854 = Bundle By Name(cluster=w1685, "ErrorArray"=w1675, "PrevErrorArray"=w1677) -> (w1684:T17)
                n855 = control-ref of="Current Errors (click to clear)"() -> (w1681:refnum<vi>)
                n856 = property on="Property Node" class="MCListbox (strict)"(reference=w1681, "ItemNames"=w1675) -> ()  [unwired: 1 in, 2 out]
                n857 = property on="Property Node" class="MCListbox (strict)"(reference=w1681, "ItemSyms"=w1680) -> ()  [unwired: 1 in, 2 out]
                n858 = control-ref of="Error History"() -> (w1678:refnum<vi>)
                n859 = property on="Property Node" class="MCListbox (strict)"(reference=w1678, "ItemNames"=w1677) -> ()  [unwired: 1 in, 2 out]
              }
            }
          }
          event "Clear All Events": Mouse Down {
            w1701 = 0 ("index")
            n860 = event-data() -> ()  [unwired: 1 in, 5 out]
            n861 = Unbundle By Name(w1714) -> ("EventArray"=w1700:string[][], "PrevEventArray"=w1712:string[][])
            n862 = Array Size(array=w1700) -> (size(s)=w1710:i32[])
            n863 = Index Array(array=w1710, index #1=w1701, index #2=1 ("index")) -> (element #1=w1708:i32)  [unwired: 1 out]
            n864 = Index Array(array=w1700, index (col)=1 ("disabled index (col)")) -> (element=w1703:string[])  [unwired: 1 in]
            n865 = Array Size(array=w1700) -> (size(s)=w1699:i32[])
            n866 = Initialize Array(0, w1708) -> (w1706:i32[])
            n867 = Index Array(array=w1703, index=w1701) -> (element=w1702:string)
            n868 = Index Array(array=w1699, index=0) -> (element=w1697:i32)
            n869 = Not Equal?(x=w1702, y="") -> (x != y?=w1705:bool)
            n870 = case shown="True" w1705 {
              tunnel: w1714 -> [w1716 w1727]
              tunnel: [w1716 w1726] -> w1713
              tunnel: w1712 -> [_ w1725]
              tunnel: w1700 -> [_ w1721]
              tunnel: w1706 -> [_ w1724]
              tunnel: w1697 -> [_ w1718]
              frame False {
              }
              frame True {
                w1717 = string[][] [] ("Item Names")
                n871 = for {
                  N: w1718 -> [_]
                  shift-right: [w1733] -> w1719
                  shift-left: w1725 -> [w1734]
                  shift-right: [w1732] -> w1722
                  shift-left: w1724 -> [w1732]
                  tunnel: w1721 -> [w1728] mode=indexing
                  n872 = Index Array(array=w1728, index=1) -> (element=w1729:string)
                  n873 = Empty String/Path?(string/path=w1729) -> (empty?=w1731:bool)
                  n874 = case shown="False" w1731 {
                    tunnel: w1734 -> [w1737 w1738]
                    tunnel: [w1736 w1738] -> w1733
                    tunnel: w1728 -> [w1735 _]
                    frame False {
                      n875 = Build Array (concatenate)(w1735, w1737) -> (w1736:string[][])
                    }
                    frame True {
                    }
                  }
                }
                n876 = Bundle By Name(cluster=w1727, "EventArray"=w1717, "PrevEventArray"=w1719) -> (w1726:T17)
                n877 = control-ref of="Current Events (click to clear)"() -> (w1723:refnum<vi>)
                n878 = property on="Property Node" class="MCListbox (strict)"(reference=w1723, "ItemNames"=w1717) -> ()  [unwired: 1 in, 2 out]
                n879 = property on="Property Node" class="MCListbox (strict)"(reference=w1723, "ItemSyms"=w1722) -> ()  [unwired: 1 in, 2 out]
                n880 = control-ref of="Event History"() -> (w1720:refnum<vi>)
                n881 = property on="Property Node" class="MCListbox (strict)"(reference=w1720, "ItemNames"=w1719) -> ()  [unwired: 1 in, 2 out]
              }
            }
          }
          event "ZoneSetup.Zone Selection": Mouse Down {
            n882 = event-data() -> ("CtlRef"=w1745:refnum<vi>, "Coords"=w1751:T30)  [unwired: 1 in]
            n883 = Unbundle By Name(w1742) -> ("ZonesSelected"=w1743:bool[])
            n884 = invoke on="Invoke Node" class="LstBox (strict)" method="Point To Row"(reference=w1745, "Point"=w1751) -> ("Row"=w1744:i32)  [unwired: 5 in, 6 out]
            n885 = property on="Property Node" class="LstBox (strict)"(reference=w1745) -> ("Item Symbols"=w1747:i32[])  [unwired: 1 in, 2 out]
            n886 = Index Array(array=w1747, index=w1744) -> (element=w1749:i32)
            n887 = Equal?(x=w1749, y=37) -> (x = y?=w1750:bool)
            n888 = case shown="True" w1750 {
              tunnel: w1747 -> [w1757 w1765]
              tunnel: w1744 -> [w1753 w1762]
              tunnel: [w1756 w1763] -> w1739
              tunnel: w1743 -> [w1755 w1760]
              tunnel: [w1752 w1759] -> w1740
              frame False {
                n889 = Replace Array Subset(array=w1755, new element=FALSE ("Boolean"), index=w1753) -> (w1752:bool[])
                n890 = Replace Array Subset(array=w1757, new element=37, index=w1753) -> (w1756:i32[])
              }
              frame True {
                n891 = Replace Array Subset(array=w1760, new element=TRUE ("Boolean"), index=w1762) -> (w1759:bool[])
                n892 = Replace Array Subset(array=w1765, new element=38, index=w1762) -> (w1763:i32[])
              }
            }
            n893 = Bundle By Name(cluster=w1742, "ZonesSelected"=w1740, "ZoneSetup.Zone Selection"=w1739) -> (w1741:T17)
            n894 = property on="Property Node" class="LstBox (strict)"(reference=w1745, "Item Symbols"=w1739) -> ()  [unwired: 1 in, 2 out]
          }
          event "ZoneSetup.Initiate Setup": Value Change {
            w1772 = TRUE ("Page Visible")
            n895 = event-data() -> ("CtlRef"=w1771:refnum<vi>, "OldVal"=w1770:bool)  [unwired: 1 in, 4 out]
            n896 = control-ref of="Thermal Profile Loader"() -> (w1784:refnum<vi>)
            n897 = property class="Bool (strict)"(reference=w1771, "Value"=w1770) -> ()  [unwired: 1 in, 2 out]
            n898 = control-ref of="Zone Selection"() -> (w1783:refnum<vi>)
            n899 = property on="Property Node" class="TabCtl (strict)"(reference=w1784) -> ("Pages"=w1775:refnum<vi>[])  [unwired: 1 in, 2 out]
            n900 = property on="Property Node" class="LstBox (strict)"(reference=w1783) -> ("Item Symbols"=w1782:i32[])  [unwired: 1 in, 2 out]
            n901 = for {
              N: 13 -> [_]
              tunnel: w1782 -> [w1838]
              tunnel: w1775 -> [w1839] mode=indexing
              i -> [w1833]
              n902 = Greater?(x=w1833, y=1) -> (0:w1835:bool)
              n903 = Less?(x=w1833, y=11 ("x")) -> (x < y?=w1836:bool)
              n904 = And(x=w1836, y=w1835) -> (x .and. y?=w1834:bool)
              n905 = case shown="True" w1834 {
                tunnel: w1839 -> [_ w1847]
                tunnel: w1838 -> [_ w1844]
                tunnel: w1833 -> [_ w1843]
                frame False {
                }
                frame True {
                  n906 = Subtract(x=w1843, y=2) -> (x-y=w1841:i32)
                  n907 = Index Array(array=w1844, index=w1841) -> (element=w1840:i32)
                  n908 = Equal?(x=38, y=w1840) -> (x = y?=w1845:bool)
                  n909 = case shown="True" w1845 {
                    tunnel: w1847 -> [w1848 w1850]
                    frame False {
                      n910 = property class="Page"(reference=w1848, "Page Visible"=FALSE) -> ()  [unwired: 1 in, 2 out]
                    }
                    frame True {
                      n911 = property class="Page"(reference=w1850, "Page Visible"=TRUE) -> ()  [unwired: 1 in, 2 out]
                    }
                  }
                }
              }
            }
            n912 = call-poly "Send Message.vi"("error in (no error)"=w1767, "event"="initThermalProfile") -> ("error out"=w1766:errorcluster)  [unwired: 9 in]
            n913 = Index Array(array=w1775, index #1=11 ("index"), index #2=1 ("index")) -> (element #1=w1779:refnum<vi>, element #2=w1773:refnum<vi>)
            n914 = property on="Number of Set points" class="DigNum (strict)"() -> ("NumText.Text"=w1776:string)  [unwired: 2 in, 2 out]
            n915 = property class="Page"(reference=w1779, "Page Visible"=w1772) -> ()  [unwired: 1 in, 2 out]
            n916 = property class="Page"(reference=w1773, "Page Visible"=w1772) -> ()  [unwired: 1 in, 2 out]
            n917 = Decimal String To Number(string=w1776) -> (number=w1769:i32)  [unwired: 2 in, 1 out]
            n918 = for {
              N: 9 -> [_]
              tunnel: w1769 -> [w1791]
              i -> [w1789]
              n919 = Initialize Array(0, w1791, 2 ("dimension size")) -> (w1790:i32[][])
              n920 = Initialize Array(0, w1791, 3 ("dimension size")) -> (w1796:i32[][])
              n921 = for {
                N: w1791 -> [_]
                shift-right: [w1830] -> w1787
                shift-left: w1796 -> [w1831]
                shift-right: [w1821] -> w1786
                shift-left: w1790 -> [w1822]
                i -> [w1819]
                w1823 = 0 ("disabled index (col)")
                w1825 = 0 ("disabled index (col)")
                n922 = Increment(x=w1819) -> (x+1=w1824:i32)
                n923 = Increment(x=w1819) -> (x+1=w1826:i32)
                n924 = Replace Array Subset(array=i32[][] [[0, 0]], new element=w1824, index (row)=w1823, index (col)=w1823) -> (w1817:i32[][])
                n925 = Replace Array Subset(array=i32[][] [[0, 0, 0]], new element=w1826, index (row)=w1825, index (col)=w1825) -> (w1829:i32[][])
                n926 = Index Array(array=w1817, index (row)=w1823) -> (element=w1820:i32[])  [unwired: 1 in]
                n927 = Index Array(array=w1829, index (row)=w1825) -> (element=w1828:i32[])  [unwired: 1 in]
                n928 = Replace Array Subset(array=w1822, new element=w1820, index (row)=w1819) -> (w1821:i32[][])  [unwired: 1 in]
                n929 = Replace Array Subset(array=w1831, new element=w1828, index (row)=w1819) -> (w1830:i32[][])  [unwired: 1 in]
              }
              n930 = To Double Precision Float(number=w1786) -> (double precision float=w1785:dbl[][])
              n931 = To Double Precision Float(number=w1787) -> (double precision float=w1788:dbl[][])
              n932 = case shown="0, Default" w1789 {
                tunnel: w1788 -> [w1798 _ _ _ _ _ _ _ _]
                tunnel: w1785 -> [w1797 w1801 w1803 w1805 w1807 w1809 w1811 w1813 w1815]
                frame 0, Default {
                  n933 = control-ref of="Temperature Goal"() -> (w1800:refnum<vi>)
                  n934 = control-ref of="RampSoakTimes"() -> (w1799:refnum<vi>)
                  n935 = property class="Arr (strict)"(reference=w1800, "Value"=w1797) -> ()  [unwired: 1 in, 2 out]
                  n936 = property class="Arr (strict)"(reference=w1799, "Value"=w1798) -> ()  [unwired: 1 in, 2 out]
                }
                frame 1 {
                  n937 = control-ref of="Temperature Goal"() -> (w1802:refnum<vi>)
                  n938 = property class="Arr (strict)"(reference=w1802, "Value"=w1801) -> ()  [unwired: 1 in, 2 out]
                }
                frame 2 {
                  n939 = control-ref of="Temperature Goal"() -> (w1804:refnum<vi>)
                  n940 = property class="Arr (strict)"(reference=w1804, "Value"=w1803) -> ()  [unwired: 1 in, 2 out]
                }
                frame 3 {
                  n941 = control-ref of="Temperature Goal"() -> (w1806:refnum<vi>)
                  n942 = property class="Arr (strict)"(reference=w1806, "Value"=w1805) -> ()  [unwired: 1 in, 2 out]
                }
                frame 4 {
                  n943 = control-ref of="Temperature Goal"() -> (w1808:refnum<vi>)
                  n944 = property class="Arr (strict)"(reference=w1808, "Value"=w1807) -> ()  [unwired: 1 in, 2 out]
                }
                frame 5 {
                  n945 = control-ref of="Temperature Goal"() -> (w1810:refnum<vi>)
                  n946 = property class="Arr (strict)"(reference=w1810, "Value"=w1809) -> ()  [unwired: 1 in, 2 out]
                }
                frame 6 {
                  n947 = control-ref of="Temperature Goal"() -> (w1812:refnum<vi>)
                  n948 = property class="Arr (strict)"(reference=w1812, "Value"=w1811) -> ()  [unwired: 1 in, 2 out]
                }
                frame 7 {
                  n949 = control-ref of="Temperature Goal"() -> (w1814:refnum<vi>)
                  n950 = property class="Arr (strict)"(reference=w1814, "Value"=w1813) -> ()  [unwired: 1 in, 2 out]
                }
                frame 8 {
                  n951 = control-ref of="Temperature Goal"() -> (w1816:refnum<vi>)
                  n952 = property class="Arr (strict)"(reference=w1816, "Value"=w1815) -> ()  [unwired: 1 in, 2 out]
                }
              }
            }
          }
          event Mouse Down {
            n953 = event-data() -> ("CtlRef"=w1852:refnum<vi>, "Coords"=w1858:T30)  [unwired: 1 in, 6 out]
            n954 = invoke on="Invoke Node" class="LstBox (strict)" method="Point To Row"(reference=w1852, "Point"=w1858) -> ("InBounds"=w1853:bool, "Row"=w1854:i32)  [unwired: 5 in, 5 out]
            n955 = property on="Property Node" class="LstBox (strict)"(reference=w1852) -> ("Item Symbols"=w1857:i32[])  [unwired: 1 in, 2 out]
            n956 = case shown="True" w1853 {
              tunnel: w1852 -> [_ w1860]
              tunnel: w1857 -> [_ w1868]
              tunnel: w1854 -> [_ w1867]
              frame False {
              }
              frame True {
                n957 = Index Array(array=w1868, index=w1867) -> (element=w1870:i32)
                n958 = control-ref of="Thermocouples Selected"() -> (w1859:refnum<vi>)
                n959 = Equal?(x=w1870, y=37) -> (x = y?=w1865:bool)
                n960 = case shown="True" w1865 {
                  tunnel: w1868 -> [w1883 w1897]
                  tunnel: w1867 -> [w1880 w1893]
                  tunnel: [w1882 w1895] -> w1862
                  tunnel: w1859 -> [w1881 w1894]
                  frame False {
                    n961 = Not Equal To 0?(x=w1880) -> (x != 0?=w1879:bool)
                    n962 = case shown="True" w1879 {
                      tunnel: w1880 -> [_ w1891]
                      tunnel: w1881 -> [_ w1890]
                      frame False {
                      }
                      frame True {
                        n963 = property class="Str"(reference=w1890) -> (reference out=w1889:refnum<vi>, "Text.Text"=w1886:string)  [unwired: 1 in, 1 out]
                        n964 = Number To Decimal String(number=w1891) -> (decimal integer string=w1888:string)  [unwired: 1 in]
                        n965 = call <vilib>:"Space Constant.vi"() -> ("String"=w1887:string)
                        n966 = Search and Replace String(input string=w1886, search string=w1888, replace string=w1887) -> (result string=w1885:string)  [unwired: 5 in, 3 out]
                        n967 = property class="Str"(reference=w1889, "Text.Text"=w1885) -> ()  [unwired: 1 in, 2 out]
                      }
                    }
                    n968 = Replace Array Subset(array=w1883, new element=37, index=w1880) -> (w1882:i32[])
                  }
                  frame True {
                    n969 = Not Equal To 0?(x=w1893) -> (x != 0?=w1892:bool)
                    n970 = case shown="False" w1892 {
                      tunnel: w1894 -> [w1898 w1905]
                      tunnel: w1893 -> [_ w1904]
                      frame False {
                        n971 = property class="Str"(reference=w1898, "Text.Text"="") -> ()  [unwired: 1 in, 2 out]
                      }
                      frame True {
                        n972 = property class="Str"(reference=w1905) -> ("Text.Text"=w1903:string)  [unwired: 1 in, 2 out]
                        n973 = Number To Decimal String(number=w1904) -> (decimal integer string=w1900:string)  [unwired: 1 in]
                        n974 = call <vilib>:"Space Constant.vi"() -> ("String"=w1901:string)
                        n975 = Concatenate Strings(w1903, w1901, w1900) -> (w1902:string)
                        n976 = property class="Str"(reference=w1905, "Text.Text"=w1902) -> ()  [unwired: 1 in, 2 out]
                      }
                    }
                    n977 = Replace Array Subset(array=w1897, new element=38, index=w1893) -> (w1895:i32[])
                  }
                }
                n978 = Equal To 0?(x=w1867) -> (x = 0?=w1866:bool)
                n979 = Array Size(array=w1862) -> (size(s)=w1861:i32)
                n980 = And(x=w1865, y=w1866) -> (x .and. y?=w1864:bool)
                n981 = case shown="True" w1864 {
                  tunnel: w1862 -> [w1871 w1874]
                  tunnel: [w1871 w1873] -> w1863
                  tunnel: w1861 -> [_ w1872]
                  frame False {
                  }
                  frame True {
                    n982 = for {
                      N: w1872 -> [_]
                      shift-right: [w1875] -> w1873
                      shift-left: w1874 -> [w1878]
                      i -> [w1877]
                      n983 = Replace Array Subset(array=w1878, new element=37, index=w1877) -> (w1875:i32[])
                    }
                  }
                }
                n984 = property on="Property Node" class="LstBox (strict)"(reference=w1860, "Item Symbols"=w1863) -> ()  [unwired: 1 in, 2 out]
              }
            }
          }
          event Mouse Down {
            n985 = event-data() -> ("CtlRef"=w1906:refnum<vi>, "Coords"=w1912:T30)  [unwired: 1 in, 6 out]
            n986 = invoke on="Invoke Node" class="LstBox (strict)" method="Point To Row"(reference=w1906, "Point"=w1912) -> ("InBounds"=w1907:bool, "Row"=w1908:i32)  [unwired: 5 in, 5 out]
            n987 = property on="Property Node" class="LstBox (strict)"(reference=w1906) -> ("Item Symbols"=w1911:i32[])  [unwired: 1 in, 2 out]
            n988 = case shown="True" w1907 {
              tunnel: w1906 -> [_ w1914]
              tunnel: w1911 -> [_ w1922]
              tunnel: w1908 -> [_ w1921]
              frame False {
              }
              frame True {
                n989 = Index Array(array=w1922, index=w1921) -> (element=w1924:i32)
                n990 = control-ref of="Thermocouples Selected"() -> (w1913:refnum<vi>)
                n991 = Equal?(x=w1924, y=37) -> (x = y?=w1919:bool)
                n992 = case shown="True" w1919 {
                  tunnel: w1922 -> [w1937 w1951]
                  tunnel: w1921 -> [w1934 w1947]
                  tunnel: [w1936 w1949] -> w1916
                  tunnel: w1913 -> [w1935 w1948]
                  frame False {
                    n993 = Not Equal To 0?(x=w1934) -> (x != 0?=w1933:bool)
                    n994 = case shown="True" w1933 {
                      tunnel: w1934 -> [_ w1945]
                      tunnel: w1935 -> [_ w1944]
                      frame False {
                      }
                      frame True {
                        n995 = property class="Str"(reference=w1944) -> (reference out=w1943:refnum<vi>, "Text.Text"=w1940:string)  [unwired: 1 in, 1 out]
                        n996 = Number To Decimal String(number=w1945) -> (decimal integer string=w1942:string)  [unwired: 1 in]
                        n997 = call <vilib>:"Space Constant.vi"() -> ("String"=w1941:string)
                        n998 = Search and Replace String(input string=w1940, search string=w1942, replace string=w1941) -> (result string=w1939:string)  [unwired: 5 in, 3 out]
                        n999 = property class="Str"(reference=w1943, "Text.Text"=w1939) -> ()  [unwired: 1 in, 2 out]
                      }
                    }
                    n1000 = Replace Array Subset(array=w1937, new element=37, index=w1934) -> (w1936:i32[])
                  }
                  frame True {
                    n1001 = Not Equal To 0?(x=w1947) -> (x != 0?=w1946:bool)
                    n1002 = case shown="True" w1946 {
                      tunnel: w1948 -> [w1952 w1959]
                      tunnel: w1947 -> [_ w1958]
                      frame False {
                        n1003 = property class="Str"(reference=w1952, "Text.Text"="") -> ()  [unwired: 1 in, 2 out]
                      }
                      frame True {
                        n1004 = property class="Str"(reference=w1959) -> ("Text.Text"=w1957:string)  [unwired: 1 in, 2 out]
                        n1005 = Number To Decimal String(number=w1958) -> (decimal integer string=w1954:string)  [unwired: 1 in]
                        n1006 = call <vilib>:"Space Constant.vi"() -> ("String"=w1955:string)
                        n1007 = Concatenate Strings(w1957, w1955, w1954) -> (w1956:string)
                        n1008 = property class="Str"(reference=w1959, "Text.Text"=w1956) -> ()  [unwired: 1 in, 2 out]
                      }
                    }
                    n1009 = Replace Array Subset(array=w1951, new element=38, index=w1947) -> (w1949:i32[])
                  }
                }
                n1010 = Equal To 0?(x=w1921) -> (x = 0?=w1920:bool)
                n1011 = Array Size(array=w1916) -> (size(s)=w1915:i32)
                n1012 = And(x=w1919, y=w1920) -> (x .and. y?=w1918:bool)
                n1013 = case shown="True" w1918 {
                  tunnel: w1916 -> [w1925 w1928]
                  tunnel: [w1925 w1927] -> w1917
                  tunnel: w1915 -> [_ w1926]
                  frame False {
                  }
                  frame True {
                    n1014 = for {
                      N: w1926 -> [_]
                      shift-right: [w1929] -> w1927
                      shift-left: w1928 -> [w1932]
                      i -> [w1931]
                      n1015 = Replace Array Subset(array=w1932, new element=37, index=w1931) -> (w1929:i32[])
                    }
                  }
                }
                n1016 = property on="Property Node" class="LstBox (strict)"(reference=w1914, "Item Symbols"=w1917) -> ()  [unwired: 1 in, 2 out]
              }
            }
          }
          event Mouse Down {
            n1017 = event-data() -> ("CtlRef"=w1960:refnum<vi>, "Coords"=w1966:T30)  [unwired: 1 in, 6 out]
            n1018 = invoke on="Invoke Node" class="LstBox (strict)" method="Point To Row"(reference=w1960, "Point"=w1966) -> ("InBounds"=w1961:bool, "Row"=w1962:i32)  [unwired: 5 in, 5 out]
            n1019 = property on="Property Node" class="LstBox (strict)"(reference=w1960) -> ("Item Symbols"=w1965:i32[])  [unwired: 1 in, 2 out]
            n1020 = case shown="True" w1961 {
              tunnel: w1960 -> [_ w1968]
              tunnel: w1965 -> [_ w1976]
              tunnel: w1962 -> [_ w1975]
              frame False {
              }
              frame True {
                n1021 = Index Array(array=w1976, index=w1975) -> (element=w1978:i32)
                n1022 = control-ref of="Thermocouples Selected"() -> (w1967:refnum<vi>)
                n1023 = Equal?(x=w1978, y=37) -> (x = y?=w1973:bool)
                n1024 = case shown="True" w1973 {
                  tunnel: w1976 -> [w1991 w2005]
                  tunnel: w1975 -> [w1988 w2001]
                  tunnel: [w1990 w2003] -> w1970
                  tunnel: w1967 -> [w1989 w2002]
                  frame False {
                    n1025 = Not Equal To 0?(x=w1988) -> (x != 0?=w1987:bool)
                    n1026 = case shown="True" w1987 {
                      tunnel: w1988 -> [_ w1999]
                      tunnel: w1989 -> [_ w1998]
                      frame False {
                      }
                      frame True {
                        n1027 = property class="Str"(reference=w1998) -> (reference out=w1997:refnum<vi>, "Text.Text"=w1994:string)  [unwired: 1 in, 1 out]
                        n1028 = Number To Decimal String(number=w1999) -> (decimal integer string=w1996:string)  [unwired: 1 in]
                        n1029 = call <vilib>:"Space Constant.vi"() -> ("String"=w1995:string)
                        n1030 = Search and Replace String(input string=w1994, search string=w1996, replace string=w1995) -> (result string=w1993:string)  [unwired: 5 in, 3 out]
                        n1031 = property class="Str"(reference=w1997, "Text.Text"=w1993) -> ()  [unwired: 1 in, 2 out]
                      }
                    }
                    n1032 = Replace Array Subset(array=w1991, new element=37, index=w1988) -> (w1990:i32[])
                  }
                  frame True {
                    n1033 = Not Equal To 0?(x=w2001) -> (x != 0?=w2000:bool)
                    n1034 = case shown="True" w2000 {
                      tunnel: w2002 -> [w2006 w2013]
                      tunnel: w2001 -> [_ w2012]
                      frame False {
                        n1035 = property class="Str"(reference=w2006, "Text.Text"="") -> ()  [unwired: 1 in, 2 out]
                      }
                      frame True {
                        n1036 = property class="Str"(reference=w2013) -> ("Text.Text"=w2011:string)  [unwired: 1 in, 2 out]
                        n1037 = Number To Decimal String(number=w2012) -> (decimal integer string=w2008:string)  [unwired: 1 in]
                        n1038 = call <vilib>:"Space Constant.vi"() -> ("String"=w2009:string)
                        n1039 = Concatenate Strings(w2011, w2009, w2008) -> (w2010:string)
                        n1040 = property class="Str"(reference=w2013, "Text.Text"=w2010) -> ()  [unwired: 1 in, 2 out]
                      }
                    }
                    n1041 = Replace Array Subset(array=w2005, new element=38, index=w2001) -> (w2003:i32[])
                  }
                }
                n1042 = Equal To 0?(x=w1975) -> (x = 0?=w1974:bool)
                n1043 = Array Size(array=w1970) -> (size(s)=w1969:i32)
                n1044 = And(x=w1973, y=w1974) -> (x .and. y?=w1972:bool)
                n1045 = case shown="True" w1972 {
                  tunnel: w1970 -> [w1979 w1982]
                  tunnel: [w1979 w1981] -> w1971
                  tunnel: w1969 -> [_ w1980]
                  frame False {
                  }
                  frame True {
                    n1046 = for {
                      N: w1980 -> [_]
                      shift-right: [w1983] -> w1981
                      shift-left: w1982 -> [w1986]
                      i -> [w1985]
                      n1047 = Replace Array Subset(array=w1986, new element=37, index=w1985) -> (w1983:i32[])
                    }
                  }
                }
                n1048 = property on="Property Node" class="LstBox (strict)"(reference=w1968, "Item Symbols"=w1971) -> ()  [unwired: 1 in, 2 out]
              }
            }
          }
          event Mouse Down {
            n1049 = event-data() -> ("CtlRef"=w2014:refnum<vi>, "Coords"=w2020:T30)  [unwired: 1 in, 6 out]
            n1050 = invoke on="Invoke Node" class="LstBox (strict)" method="Point To Row"(reference=w2014, "Point"=w2020) -> ("InBounds"=w2015:bool, "Row"=w2016:i32)  [unwired: 5 in, 5 out]
            n1051 = property on="Property Node" class="LstBox (strict)"(reference=w2014) -> ("Item Symbols"=w2019:i32[])  [unwired: 1 in, 2 out]
            n1052 = case shown="True" w2015 {
              tunnel: w2014 -> [_ w2022]
              tunnel: w2019 -> [_ w2030]
              tunnel: w2016 -> [_ w2029]
              frame False {
              }
              frame True {
                n1053 = Index Array(array=w2030, index=w2029) -> (element=w2032:i32)
                n1054 = control-ref of="Thermocouples Selected"() -> (w2021:refnum<vi>)
                n1055 = Equal?(x=w2032, y=37) -> (x = y?=w2027:bool)
                n1056 = case shown="True" w2027 {
                  tunnel: w2030 -> [w2045 w2059]
                  tunnel: w2029 -> [w2042 w2055]
                  tunnel: [w2044 w2057] -> w2024
                  tunnel: w2021 -> [w2043 w2056]
                  frame False {
                    n1057 = Not Equal To 0?(x=w2042) -> (x != 0?=w2041:bool)
                    n1058 = case shown="True" w2041 {
                      tunnel: w2042 -> [_ w2053]
                      tunnel: w2043 -> [_ w2052]
                      frame False {
                      }
                      frame True {
                        n1059 = property class="Str"(reference=w2052) -> (reference out=w2051:refnum<vi>, "Text.Text"=w2048:string)  [unwired: 1 in, 1 out]
                        n1060 = Number To Decimal String(number=w2053) -> (decimal integer string=w2050:string)  [unwired: 1 in]
                        n1061 = call <vilib>:"Space Constant.vi"() -> ("String"=w2049:string)
                        n1062 = Search and Replace String(input string=w2048, search string=w2050, replace string=w2049) -> (result string=w2047:string)  [unwired: 5 in, 3 out]
                        n1063 = property class="Str"(reference=w2051, "Text.Text"=w2047) -> ()  [unwired: 1 in, 2 out]
                      }
                    }
                    n1064 = Replace Array Subset(array=w2045, new element=37, index=w2042) -> (w2044:i32[])
                  }
                  frame True {
                    n1065 = Not Equal To 0?(x=w2055) -> (x != 0?=w2054:bool)
                    n1066 = case shown="True" w2054 {
                      tunnel: w2056 -> [w2060 w2067]
                      tunnel: w2055 -> [_ w2066]
                      frame False {
                        n1067 = property class="Str"(reference=w2060, "Text.Text"="") -> ()  [unwired: 1 in, 2 out]
                      }
                      frame True {
                        n1068 = property class="Str"(reference=w2067) -> ("Text.Text"=w2065:string)  [unwired: 1 in, 2 out]
                        n1069 = Number To Decimal String(number=w2066) -> (decimal integer string=w2062:string)  [unwired: 1 in]
                        n1070 = call <vilib>:"Space Constant.vi"() -> ("String"=w2063:string)
                        n1071 = Concatenate Strings(w2065, w2063, w2062) -> (w2064:string)
                        n1072 = property class="Str"(reference=w2067, "Text.Text"=w2064) -> ()  [unwired: 1 in, 2 out]
                      }
                    }
                    n1073 = Replace Array Subset(array=w2059, new element=38, index=w2055) -> (w2057:i32[])
                  }
                }
                n1074 = Equal To 0?(x=w2029) -> (x = 0?=w2028:bool)
                n1075 = Array Size(array=w2024) -> (size(s)=w2023:i32)
                n1076 = And(x=w2027, y=w2028) -> (x .and. y?=w2026:bool)
                n1077 = case shown="True" w2026 {
                  tunnel: w2024 -> [w2033 w2036]
                  tunnel: [w2033 w2035] -> w2025
                  tunnel: w2023 -> [_ w2034]
                  frame False {
                  }
                  frame True {
                    n1078 = for {
                      N: w2034 -> [_]
                      shift-right: [w2037] -> w2035
                      shift-left: w2036 -> [w2040]
                      i -> [w2039]
                      n1079 = Replace Array Subset(array=w2040, new element=37, index=w2039) -> (w2037:i32[])
                    }
                  }
                }
                n1080 = property on="Property Node" class="LstBox (strict)"(reference=w2022, "Item Symbols"=w2025) -> ()  [unwired: 1 in, 2 out]
              }
            }
          }
          event Mouse Down {
            n1081 = event-data() -> ("CtlRef"=w2068:refnum<vi>, "Coords"=w2074:T30)  [unwired: 1 in, 6 out]
            n1082 = invoke on="Invoke Node" class="LstBox (strict)" method="Point To Row"(reference=w2068, "Point"=w2074) -> ("InBounds"=w2069:bool, "Row"=w2070:i32)  [unwired: 5 in, 5 out]
            n1083 = property on="Property Node" class="LstBox (strict)"(reference=w2068) -> ("Item Symbols"=w2073:i32[])  [unwired: 1 in, 2 out]
            n1084 = case shown="True" w2069 {
              tunnel: w2068 -> [_ w2076]
              tunnel: w2073 -> [_ w2084]
              tunnel: w2070 -> [_ w2083]
              frame False {
              }
              frame True {
                n1085 = Index Array(array=w2084, index=w2083) -> (element=w2086:i32)
                n1086 = control-ref of="Thermocouples Selected"() -> (w2075:refnum<vi>)
                n1087 = Equal?(x=w2086, y=37) -> (x = y?=w2081:bool)
                n1088 = case shown="True" w2081 {
                  tunnel: w2084 -> [w2099 w2113]
                  tunnel: w2083 -> [w2096 w2109]
                  tunnel: [w2098 w2111] -> w2078
                  tunnel: w2075 -> [w2097 w2110]
                  frame False {
                    n1089 = Not Equal To 0?(x=w2096) -> (x != 0?=w2095:bool)
                    n1090 = case shown="True" w2095 {
                      tunnel: w2096 -> [_ w2107]
                      tunnel: w2097 -> [_ w2106]
                      frame False {
                      }
                      frame True {
                        n1091 = property class="Str"(reference=w2106) -> (reference out=w2105:refnum<vi>, "Text.Text"=w2102:string)  [unwired: 1 in, 1 out]
                        n1092 = Number To Decimal String(number=w2107) -> (decimal integer string=w2104:string)  [unwired: 1 in]
                        n1093 = call <vilib>:"Space Constant.vi"() -> ("String"=w2103:string)
                        n1094 = Search and Replace String(input string=w2102, search string=w2104, replace string=w2103) -> (result string=w2101:string)  [unwired: 5 in, 3 out]
                        n1095 = property class="Str"(reference=w2105, "Text.Text"=w2101) -> ()  [unwired: 1 in, 2 out]
                      }
                    }
                    n1096 = Replace Array Subset(array=w2099, new element=37, index=w2096) -> (w2098:i32[])
                  }
                  frame True {
                    n1097 = Not Equal To 0?(x=w2109) -> (x != 0?=w2108:bool)
                    n1098 = case shown="True" w2108 {
                      tunnel: w2110 -> [w2114 w2121]
                      tunnel: w2109 -> [_ w2120]
                      frame False {
                        n1099 = property class="Str"(reference=w2114, "Text.Text"="") -> ()  [unwired: 1 in, 2 out]
                      }
                      frame True {
                        n1100 = property class="Str"(reference=w2121) -> ("Text.Text"=w2119:string)  [unwired: 1 in, 2 out]
                        n1101 = Number To Decimal String(number=w2120) -> (decimal integer string=w2116:string)  [unwired: 1 in]
                        n1102 = call <vilib>:"Space Constant.vi"() -> ("String"=w2117:string)
                        n1103 = Concatenate Strings(w2119, w2117, w2116) -> (w2118:string)
                        n1104 = property class="Str"(reference=w2121, "Text.Text"=w2118) -> ()  [unwired: 1 in, 2 out]
                      }
                    }
                    n1105 = Replace Array Subset(array=w2113, new element=38, index=w2109) -> (w2111:i32[])
                  }
                }
                n1106 = Equal To 0?(x=w2083) -> (x = 0?=w2082:bool)
                n1107 = Array Size(array=w2078) -> (size(s)=w2077:i32)
                n1108 = And(x=w2081, y=w2082) -> (x .and. y?=w2080:bool)
                n1109 = case shown="True" w2080 {
                  tunnel: w2078 -> [w2087 w2090]
                  tunnel: [w2087 w2089] -> w2079
                  tunnel: w2077 -> [_ w2088]
                  frame False {
                  }
                  frame True {
                    n1110 = for {
                      N: w2088 -> [_]
                      shift-right: [w2091] -> w2089
                      shift-left: w2090 -> [w2094]
                      i -> [w2093]
                      n1111 = Replace Array Subset(array=w2094, new element=37, index=w2093) -> (w2091:i32[])
                    }
                  }
                }
                n1112 = property on="Property Node" class="LstBox (strict)"(reference=w2076, "Item Symbols"=w2079) -> ()  [unwired: 1 in, 2 out]
              }
            }
          }
          event Mouse Down {
            n1113 = event-data() -> ("CtlRef"=w2122:refnum<vi>, "Coords"=w2128:T30)  [unwired: 1 in, 6 out]
            n1114 = invoke on="Invoke Node" class="LstBox (strict)" method="Point To Row"(reference=w2122, "Point"=w2128) -> ("InBounds"=w2123:bool, "Row"=w2124:i32)  [unwired: 5 in, 5 out]
            n1115 = property on="Property Node" class="LstBox (strict)"(reference=w2122) -> ("Item Symbols"=w2127:i32[])  [unwired: 1 in, 2 out]
            n1116 = case shown="True" w2123 {
              tunnel: w2122 -> [_ w2130]
              tunnel: w2127 -> [_ w2138]
              tunnel: w2124 -> [_ w2137]
              frame False {
              }
              frame True {
                n1117 = Index Array(array=w2138, index=w2137) -> (element=w2140:i32)
                n1118 = control-ref of="Thermocouples Selected"() -> (w2129:refnum<vi>)
                n1119 = Equal?(x=w2140, y=37) -> (x = y?=w2135:bool)
                n1120 = case shown="True" w2135 {
                  tunnel: w2138 -> [w2153 w2167]
                  tunnel: w2137 -> [w2150 w2163]
                  tunnel: [w2152 w2165] -> w2132
                  tunnel: w2129 -> [w2151 w2164]
                  frame False {
                    n1121 = Not Equal To 0?(x=w2150) -> (x != 0?=w2149:bool)
                    n1122 = case shown="True" w2149 {
                      tunnel: w2150 -> [_ w2161]
                      tunnel: w2151 -> [_ w2160]
                      frame False {
                      }
                      frame True {
                        n1123 = property class="Str"(reference=w2160) -> (reference out=w2159:refnum<vi>, "Text.Text"=w2156:string)  [unwired: 1 in, 1 out]
                        n1124 = Number To Decimal String(number=w2161) -> (decimal integer string=w2158:string)  [unwired: 1 in]
                        n1125 = call <vilib>:"Space Constant.vi"() -> ("String"=w2157:string)
                        n1126 = Search and Replace String(input string=w2156, search string=w2158, replace string=w2157) -> (result string=w2155:string)  [unwired: 5 in, 3 out]
                        n1127 = property class="Str"(reference=w2159, "Text.Text"=w2155) -> ()  [unwired: 1 in, 2 out]
                      }
                    }
                    n1128 = Replace Array Subset(array=w2153, new element=37, index=w2150) -> (w2152:i32[])
                  }
                  frame True {
                    n1129 = Not Equal To 0?(x=w2163) -> (x != 0?=w2162:bool)
                    n1130 = case shown="True" w2162 {
                      tunnel: w2164 -> [w2168 w2175]
                      tunnel: w2163 -> [_ w2174]
                      frame False {
                        n1131 = property class="Str"(reference=w2168, "Text.Text"="") -> ()  [unwired: 1 in, 2 out]
                      }
                      frame True {
                        n1132 = property class="Str"(reference=w2175) -> ("Text.Text"=w2173:string)  [unwired: 1 in, 2 out]
                        n1133 = Number To Decimal String(number=w2174) -> (decimal integer string=w2170:string)  [unwired: 1 in]
                        n1134 = call <vilib>:"Space Constant.vi"() -> ("String"=w2171:string)
                        n1135 = Concatenate Strings(w2173, w2171, w2170) -> (w2172:string)
                        n1136 = property class="Str"(reference=w2175, "Text.Text"=w2172) -> ()  [unwired: 1 in, 2 out]
                      }
                    }
                    n1137 = Replace Array Subset(array=w2167, new element=38, index=w2163) -> (w2165:i32[])
                  }
                }
                n1138 = Equal To 0?(x=w2137) -> (x = 0?=w2136:bool)
                n1139 = Array Size(array=w2132) -> (size(s)=w2131:i32)
                n1140 = And(x=w2135, y=w2136) -> (x .and. y?=w2134:bool)
                n1141 = case shown="True" w2134 {
                  tunnel: w2132 -> [w2141 w2144]
                  tunnel: [w2141 w2143] -> w2133
                  tunnel: w2131 -> [_ w2142]
                  frame False {
                  }
                  frame True {
                    n1142 = for {
                      N: w2142 -> [_]
                      shift-right: [w2145] -> w2143
                      shift-left: w2144 -> [w2148]
                      i -> [w2147]
                      n1143 = Replace Array Subset(array=w2148, new element=37, index=w2147) -> (w2145:i32[])
                    }
                  }
                }
                n1144 = property on="Property Node" class="LstBox (strict)"(reference=w2130, "Item Symbols"=w2133) -> ()  [unwired: 1 in, 2 out]
              }
            }
          }
          event Mouse Down {
            n1145 = event-data() -> ("CtlRef"=w2176:refnum<vi>, "Coords"=w2182:T30)  [unwired: 1 in, 6 out]
            n1146 = invoke on="Invoke Node" class="LstBox (strict)" method="Point To Row"(reference=w2176, "Point"=w2182) -> ("InBounds"=w2177:bool, "Row"=w2178:i32)  [unwired: 5 in, 5 out]
            n1147 = property on="Property Node" class="LstBox (strict)"(reference=w2176) -> ("Item Symbols"=w2181:i32[])  [unwired: 1 in, 2 out]
            n1148 = case shown="True" w2177 {
              tunnel: w2176 -> [_ w2184]
              tunnel: w2181 -> [_ w2192]
              tunnel: w2178 -> [_ w2191]
              frame False {
              }
              frame True {
                n1149 = Index Array(array=w2192, index=w2191) -> (element=w2194:i32)
                n1150 = control-ref of="Thermocouples Selected"() -> (w2183:refnum<vi>)
                n1151 = Equal?(x=w2194, y=37) -> (x = y?=w2189:bool)
                n1152 = case shown="True" w2189 {
                  tunnel: w2192 -> [w2207 w2221]
                  tunnel: w2191 -> [w2204 w2217]
                  tunnel: [w2206 w2219] -> w2186
                  tunnel: w2183 -> [w2205 w2218]
                  frame False {
                    n1153 = Not Equal To 0?(x=w2204) -> (x != 0?=w2203:bool)
                    n1154 = case shown="True" w2203 {
                      tunnel: w2204 -> [_ w2215]
                      tunnel: w2205 -> [_ w2214]
                      frame False {
                      }
                      frame True {
                        n1155 = property class="Str"(reference=w2214) -> (reference out=w2213:refnum<vi>, "Text.Text"=w2210:string)  [unwired: 1 in, 1 out]
                        n1156 = Number To Decimal String(number=w2215) -> (decimal integer string=w2212:string)  [unwired: 1 in]
                        n1157 = call <vilib>:"Space Constant.vi"() -> ("String"=w2211:string)
                        n1158 = Search and Replace String(input string=w2210, search string=w2212, replace string=w2211) -> (result string=w2209:string)  [unwired: 5 in, 3 out]
                        n1159 = property class="Str"(reference=w2213, "Text.Text"=w2209) -> ()  [unwired: 1 in, 2 out]
                      }
                    }
                    n1160 = Replace Array Subset(array=w2207, new element=37, index=w2204) -> (w2206:i32[])
                  }
                  frame True {
                    n1161 = Not Equal To 0?(x=w2217) -> (x != 0?=w2216:bool)
                    n1162 = case shown="True" w2216 {
                      tunnel: w2218 -> [w2222 w2229]
                      tunnel: w2217 -> [_ w2228]
                      frame False {
                        n1163 = property class="Str"(reference=w2222, "Text.Text"="") -> ()  [unwired: 1 in, 2 out]
                      }
                      frame True {
                        n1164 = property class="Str"(reference=w2229) -> ("Text.Text"=w2227:string)  [unwired: 1 in, 2 out]
                        n1165 = Number To Decimal String(number=w2228) -> (decimal integer string=w2224:string)  [unwired: 1 in]
                        n1166 = call <vilib>:"Space Constant.vi"() -> ("String"=w2225:string)
                        n1167 = Concatenate Strings(w2227, w2225, w2224) -> (w2226:string)
                        n1168 = property class="Str"(reference=w2229, "Text.Text"=w2226) -> ()  [unwired: 1 in, 2 out]
                      }
                    }
                    n1169 = Replace Array Subset(array=w2221, new element=38, index=w2217) -> (w2219:i32[])
                  }
                }
                n1170 = Equal To 0?(x=w2191) -> (x = 0?=w2190:bool)
                n1171 = Array Size(array=w2186) -> (size(s)=w2185:i32)
                n1172 = And(x=w2189, y=w2190) -> (x .and. y?=w2188:bool)
                n1173 = case shown="True" w2188 {
                  tunnel: w2186 -> [w2195 w2198]
                  tunnel: [w2195 w2197] -> w2187
                  tunnel: w2185 -> [_ w2196]
                  frame False {
                  }
                  frame True {
                    n1174 = for {
                      N: w2196 -> [_]
                      shift-right: [w2199] -> w2197
                      shift-left: w2198 -> [w2202]
                      i -> [w2201]
                      n1175 = Replace Array Subset(array=w2202, new element=37, index=w2201) -> (w2199:i32[])
                    }
                  }
                }
                n1176 = property on="Property Node" class="LstBox (strict)"(reference=w2184, "Item Symbols"=w2187) -> ()  [unwired: 1 in, 2 out]
              }
            }
          }
          event Mouse Down {
            n1177 = event-data() -> ("CtlRef"=w2230:refnum<vi>, "Coords"=w2236:T30)  [unwired: 1 in, 6 out]
            n1178 = invoke on="Invoke Node" class="LstBox (strict)" method="Point To Row"(reference=w2230, "Point"=w2236) -> ("InBounds"=w2231:bool, "Row"=w2232:i32)  [unwired: 5 in, 5 out]
            n1179 = property on="Property Node" class="LstBox (strict)"(reference=w2230) -> ("Item Symbols"=w2235:i32[])  [unwired: 1 in, 2 out]
            n1180 = case shown="True" w2231 {
              tunnel: w2230 -> [_ w2238]
              tunnel: w2235 -> [_ w2246]
              tunnel: w2232 -> [_ w2245]
              frame False {
              }
              frame True {
                n1181 = Index Array(array=w2246, index=w2245) -> (element=w2248:i32)
                n1182 = control-ref of="Thermocouples Selected"() -> (w2237:refnum<vi>)
                n1183 = Equal?(x=w2248, y=37) -> (x = y?=w2243:bool)
                n1184 = case shown="True" w2243 {
                  tunnel: w2246 -> [w2261 w2275]
                  tunnel: w2245 -> [w2258 w2271]
                  tunnel: [w2260 w2273] -> w2240
                  tunnel: w2237 -> [w2259 w2272]
                  frame False {
                    n1185 = Not Equal To 0?(x=w2258) -> (x != 0?=w2257:bool)
                    n1186 = case shown="True" w2257 {
                      tunnel: w2258 -> [_ w2269]
                      tunnel: w2259 -> [_ w2268]
                      frame False {
                      }
                      frame True {
                        n1187 = property class="Str"(reference=w2268) -> (reference out=w2267:refnum<vi>, "Text.Text"=w2264:string)  [unwired: 1 in, 1 out]
                        n1188 = Number To Decimal String(number=w2269) -> (decimal integer string=w2266:string)  [unwired: 1 in]
                        n1189 = call <vilib>:"Space Constant.vi"() -> ("String"=w2265:string)
                        n1190 = Search and Replace String(input string=w2264, search string=w2266, replace string=w2265) -> (result string=w2263:string)  [unwired: 5 in, 3 out]
                        n1191 = property class="Str"(reference=w2267, "Text.Text"=w2263) -> ()  [unwired: 1 in, 2 out]
                      }
                    }
                    n1192 = Replace Array Subset(array=w2261, new element=37, index=w2258) -> (w2260:i32[])
                  }
                  frame True {
                    n1193 = Not Equal To 0?(x=w2271) -> (x != 0?=w2270:bool)
                    n1194 = case shown="True" w2270 {
                      tunnel: w2272 -> [w2276 w2283]
                      tunnel: w2271 -> [_ w2282]
                      frame False {
                        n1195 = property class="Str"(reference=w2276, "Text.Text"="") -> ()  [unwired: 1 in, 2 out]
                      }
                      frame True {
                        n1196 = property class="Str"(reference=w2283) -> ("Text.Text"=w2281:string)  [unwired: 1 in, 2 out]
                        n1197 = Number To Decimal String(number=w2282) -> (decimal integer string=w2278:string)  [unwired: 1 in]
                        n1198 = call <vilib>:"Space Constant.vi"() -> ("String"=w2279:string)
                        n1199 = Concatenate Strings(w2281, w2279, w2278) -> (w2280:string)
                        n1200 = property class="Str"(reference=w2283, "Text.Text"=w2280) -> ()  [unwired: 1 in, 2 out]
                      }
                    }
                    n1201 = Replace Array Subset(array=w2275, new element=38, index=w2271) -> (w2273:i32[])
                  }
                }
                n1202 = Equal To 0?(x=w2245) -> (x = 0?=w2244:bool)
                n1203 = Array Size(array=w2240) -> (size(s)=w2239:i32)
                n1204 = And(x=w2243, y=w2244) -> (x .and. y?=w2242:bool)
                n1205 = case shown="True" w2242 {
                  tunnel: w2240 -> [w2249 w2252]
                  tunnel: [w2249 w2251] -> w2241
                  tunnel: w2239 -> [_ w2250]
                  frame False {
                  }
                  frame True {
                    n1206 = for {
                      N: w2250 -> [_]
                      shift-right: [w2253] -> w2251
                      shift-left: w2252 -> [w2256]
                      i -> [w2255]
                      n1207 = Replace Array Subset(array=w2256, new element=37, index=w2255) -> (w2253:i32[])
                    }
                  }
                }
                n1208 = property on="Property Node" class="LstBox (strict)"(reference=w2238, "Item Symbols"=w2241) -> ()  [unwired: 1 in, 2 out]
              }
            }
          }
          event Mouse Down {
            n1209 = event-data() -> ("CtlRef"=w2284:refnum<vi>, "Coords"=w2290:T30)  [unwired: 1 in, 6 out]
            n1210 = invoke on="Invoke Node" class="LstBox (strict)" method="Point To Row"(reference=w2284, "Point"=w2290) -> ("InBounds"=w2285:bool, "Row"=w2286:i32)  [unwired: 5 in, 5 out]
            n1211 = property on="Property Node" class="LstBox (strict)"(reference=w2284) -> ("Item Symbols"=w2289:i32[])  [unwired: 1 in, 2 out]
            n1212 = case shown="True" w2285 {
              tunnel: w2284 -> [_ w2292]
              tunnel: w2289 -> [_ w2300]
              tunnel: w2286 -> [_ w2299]
              frame False {
              }
              frame True {
                n1213 = Index Array(array=w2300, index=w2299) -> (element=w2302:i32)
                n1214 = control-ref of="Thermocouples Selected"() -> (w2291:refnum<vi>)
                n1215 = Equal?(x=w2302, y=37) -> (x = y?=w2297:bool)
                n1216 = case shown="True" w2297 {
                  tunnel: w2300 -> [w2315 w2329]
                  tunnel: w2299 -> [w2312 w2325]
                  tunnel: [w2314 w2327] -> w2294
                  tunnel: w2291 -> [w2313 w2326]
                  frame False {
                    n1217 = Not Equal To 0?(x=w2312) -> (x != 0?=w2311:bool)
                    n1218 = case shown="True" w2311 {
                      tunnel: w2312 -> [_ w2323]
                      tunnel: w2313 -> [_ w2322]
                      frame False {
                      }
                      frame True {
                        n1219 = property class="Str"(reference=w2322) -> (reference out=w2321:refnum<vi>, "Text.Text"=w2318:string)  [unwired: 1 in, 1 out]
                        n1220 = Number To Decimal String(number=w2323) -> (decimal integer string=w2320:string)  [unwired: 1 in]
                        n1221 = call <vilib>:"Space Constant.vi"() -> ("String"=w2319:string)
                        n1222 = Search and Replace String(input string=w2318, search string=w2320, replace string=w2319) -> (result string=w2317:string)  [unwired: 5 in, 3 out]
                        n1223 = property class="Str"(reference=w2321, "Text.Text"=w2317) -> ()  [unwired: 1 in, 2 out]
                      }
                    }
                    n1224 = Replace Array Subset(array=w2315, new element=37, index=w2312) -> (w2314:i32[])
                  }
                  frame True {
                    n1225 = Not Equal To 0?(x=w2325) -> (x != 0?=w2324:bool)
                    n1226 = case shown="True" w2324 {
                      tunnel: w2326 -> [w2330 w2337]
                      tunnel: w2325 -> [_ w2336]
                      frame False {
                        n1227 = property class="Str"(reference=w2330, "Text.Text"="") -> ()  [unwired: 1 in, 2 out]
                      }
                      frame True {
                        n1228 = property class="Str"(reference=w2337) -> ("Text.Text"=w2335:string)  [unwired: 1 in, 2 out]
                        n1229 = Number To Decimal String(number=w2336) -> (decimal integer string=w2332:string)  [unwired: 1 in]
                        n1230 = call <vilib>:"Space Constant.vi"() -> ("String"=w2333:string)
                        n1231 = Concatenate Strings(w2335, w2333, w2332) -> (w2334:string)
                        n1232 = property class="Str"(reference=w2337, "Text.Text"=w2334) -> ()  [unwired: 1 in, 2 out]
                      }
                    }
                    n1233 = Replace Array Subset(array=w2329, new element=38, index=w2325) -> (w2327:i32[])
                  }
                }
                n1234 = Equal To 0?(x=w2299) -> (x = 0?=w2298:bool)
                n1235 = Array Size(array=w2294) -> (size(s)=w2293:i32)
                n1236 = And(x=w2297, y=w2298) -> (x .and. y?=w2296:bool)
                n1237 = case shown="True" w2296 {
                  tunnel: w2294 -> [w2303 w2306]
                  tunnel: [w2303 w2305] -> w2295
                  tunnel: w2293 -> [_ w2304]
                  frame False {
                  }
                  frame True {
                    n1238 = for {
                      N: w2304 -> [_]
                      shift-right: [w2307] -> w2305
                      shift-left: w2306 -> [w2310]
                      i -> [w2309]
                      n1239 = Replace Array Subset(array=w2310, new element=37, index=w2309) -> (w2307:i32[])
                    }
                  }
                }
                n1240 = property on="Property Node" class="LstBox (strict)"(reference=w2292, "Item Symbols"=w2295) -> ()  [unwired: 1 in, 2 out]
              }
            }
          }
          event "Export Errors": Mouse Down {
            n1241 = event-data() -> ()  [unwired: 1 in, 1 out]
            n1242 = Unbundle By Name(w2341) -> ("MasterErrorArray"=w2338:string[][])
            n1243 = call-poly <vilib>:"Write Delimited Spreadsheet.vi"("2D data"=w2338, "error in (no error)"=w2340) -> ("error out"=w2339:errorcluster)  [unwired: 12 in, 1 out]
          }
          event "Export Events": Mouse Down {
            n1244 = event-data() -> ()  [unwired: 1 in, 1 out]
            n1245 = Unbundle By Name(w2345) -> ("MasterEventArray"=w2342:string[][])
            n1246 = call-poly <vilib>:"Write Delimited Spreadsheet.vi"("2D data"=w2342, "error in (no error)"=w2344) -> ("error out"=w2343:errorcluster)  [unwired: 12 in, 1 out]
          }
          event "Import UUT": Mouse Down {
            n1247 = event-data() -> ()  [unwired: 1 in, 1 out]
            n1248 = call "File Dialog"("prompt"="Select a new image for the UUT", "error in"=w2356, "pattern (all files)"="*.png;*.jpg;*.JPEG") -> ("selected path"=w2350:path, "error out"=w2354:errorcluster)  [unwired: 9 in, 2 out]
            n1249 = Path To String(path=w2350) -> (string=w2349:string)
            n1250 = local write "Path to PNG file"(w2350) -> ()
            n1251 = Match Pattern(string=w2349, regular expression="png") -> (match substring=w2347:string)  [unwired: 1 in, 3 out]
            n1252 = Empty String/Path?(string/path=w2347) -> (empty?=w2346:bool)
            n1253 = case shown="True" w2346 {
              tunnel: [w2364 w2369] -> w2355
              tunnel: w2354 -> [w2363 w2366]
              tunnel: [w2362 w2367] -> w2353
              tunnel: w2350 -> [w2360 w2365]
              frame False {
                n1254 = call <vilib>:"Read PNG File.vi"("error in (no error)"=w2363, "path to PNG file"=w2360) -> ("error out"=w2362:errorcluster, "image data"=w2361:T29)  [unwired: 7 in, 1 out]
                n1255 = call <vilib>:"Draw Flattened Pixmap.vi"("image data"=w2361) -> ("new picture"=w2364:picture)  [unwired: 8 in]
              }
              frame True {
                n1256 = call <vilib>:"Read JPEG File.vi"("error in (no error)"=w2366, "path to JPEG file"=w2365) -> ("error out"=w2367:errorcluster, "image data"=w2368:T29)  [unwired: 7 in, 1 out]
                n1257 = call <vilib>:"Draw Flattened Pixmap.vi"("image data"=w2368) -> ("new picture"=w2369:picture)  [unwired: 8 in]
              }
            }
            n1258 = local read "TC1to75visual"() -> (w2351:T8)
            n1259 = Bundle By Name(cluster=w2351, "new picture"=w2355) -> (w2352:T8)
            n1260 = local write "TC1to75visual"(w2352) -> ()
          }
          event "exit": Value Change {
            n1261 = event-data() -> ()  [unwired: 1 in, 1 out]
            n1262 = call "Broadcast Message.vi"("error in (no error)"=w2372, "event"="exit") -> ("error out"=w2370:errorcluster)  [unwired: 9 in]
          }
        }
      }
      frame "compileProfile" {
        n1263 = Empty String/Path?(string/path=w2393) -> (empty?=w2395:bool)
        n1264 = case shown="False" w2395 {
          tunnel: [w2436 0.0] -> w2394
          tunnel: w2393 -> [w2440 _]
          frame False {
            n1265 = Equal?(x=w2440, y="2") -> (x = y?=w2438:bool)
            n1266 = case shown="True" w2438 {
              tunnel: 1.0 -> [w2441 w2443]
              tunnel: [w2441 w2442] -> w2436
              frame False {
              }
              frame True {
                n1267 = local read "importexe"() -> (w2445:dbl)
                n1268 = Equal?(x=w2445, y=2.0) -> (x = y?=w2446:bool)
                n1269 = case shown="True" w2446 {
                  tunnel: w2443 -> [_ w2448]
                  tunnel: [0.0 w2448] -> w2442
                  frame False {
                  }
                  frame True {
                    n1270 = local write "importexe"(0.0 ("importexe")) -> ()
                  }
                }
              }
            }
          }
          frame True {
          }
        }
        n1271 = local write "ThermalProfileStatus"("Compiling..........." ("String")) -> ()
        n1272 = Initialize Array(T22 {"zone"=0, "average"="", "thermocouples"=[0], "maxTemp"=0, "minTemp"=0, "maxSlope"=0.0, "thermalprofiles"=[{"thermalsetpoint"=0, "tempgoal"=0, "ramp"=0, "soakduration"=0}]} ("ThermalProfileCluster.profiles"), 1 ("dimension size")) -> (w2429:T32)
        n1273 = Unbundle By Name(w2431) -> ("ZonesSelected"=w2432:bool[], "ZoneSetup.Number of Set points"=w2430:dbl)
        n1274 = for {
          N: 9 -> [_]
          tunnel: w2431 -> [w2567]
          tunnel: w2432 -> [w2566] mode=indexing
          shift-right: [w2564] -> w2404
          shift-left: w2431 -> [w2565]
          tunnel: w2430 -> [w2560]
          shift-right: [w2558] -> w2426
          shift-left: w2429 -> [w2559]
          shift-right: [w2556] -> w2375
          shift-left: w2376 -> [w2556]
          i -> [w2557]
          w2563 = 0  # zone
          n1275 = Add(x=w2563, y=w2557) -> (x+y=w2562:i32)
          n1276 = Increment(x=w2562) -> (x+1=w2561:i32)
          n1277 = case shown="True" w2566 {
            tunnel: w2567 -> [_ _]
            tunnel: w2557 -> [_ w2599]
            tunnel: w2565 -> [w2569 w2603]
            tunnel: [w2569 w2603] -> w2564
            tunnel: w2561 -> [_ w2604]
            tunnel: w2560 -> [_ w2597]
            tunnel: w2559 -> [w2568 w2573]
            tunnel: [w2568 w2572] -> w2558
            tunnel: w2557 -> [_ _]
            frame False {
            }
            frame True {
              n1278 = case shown="0, Default" w2599 {
                tunnel: [w2624 w2630 w2636 w2642 w2648 w2654 w2660 w2666 w2672] -> w2593
                tunnel: [w2623 w2629 w2635 w2641 w2647 w2653 w2659 w2665 w2671] -> w2598
                tunnel: [w2622 w2628 w2634 w2640 w2646 w2652 w2658 w2664 w2670] -> w2588
                tunnel: [w2621 w2627 w2633 w2639 w2645 w2651 w2657 w2663 w2669] -> w2583
                tunnel: [w2620 w2626 w2632 w2638 w2644 w2650 w2656 w2662 w2668] -> w2582
                tunnel: [w2619 w2625 w2631 w2637 w2643 w2649 w2655 w2661 w2667] -> w2578
                frame 0, Default {
                  n1279 = control-ref of="Zone Thermocouples"() -> (w2624:refnum<vi>)
                  n1280 = control-ref of="Temperature Goal"() -> (w2622:refnum<vi>)
                  n1281 = control-ref of="Max Temp Slope"() -> (w2619:refnum<vi>)
                  n1282 = control-ref of="Max Allowable Temp"() -> (w2621:refnum<vi>)
                  n1283 = control-ref of="Temperature Calculation"() -> (w2623:refnum<vi>)
                  n1284 = control-ref of="Min Allowable Temp"() -> (w2620:refnum<vi>)
                }
                frame 1 {
                  n1285 = control-ref of="Zone Thermocouples"() -> (w2630:refnum<vi>)
                  n1286 = control-ref of="Max Temp Slope"() -> (w2625:refnum<vi>)
                  n1287 = control-ref of="Temperature Goal"() -> (w2628:refnum<vi>)
                  n1288 = control-ref of="Max Allowable Temp"() -> (w2627:refnum<vi>)
                  n1289 = control-ref of="Temperature Calculation"() -> (w2629:refnum<vi>)
                  n1290 = control-ref of="Min Allowable Temp"() -> (w2626:refnum<vi>)
                }
                frame 2 {
                  n1291 = control-ref of="Zone Thermocouples"() -> (w2636:refnum<vi>)
                  n1292 = control-ref of="Max Temp Slope"() -> (w2631:refnum<vi>)
                  n1293 = control-ref of="Temperature Goal"() -> (w2634:refnum<vi>)
                  n1294 = control-ref of="Max Allowable Temp"() -> (w2633:refnum<vi>)
                  n1295 = control-ref of="Temperature Calculation"() -> (w2635:refnum<vi>)
                  n1296 = control-ref of="Min Allowable Temp"() -> (w2632:refnum<vi>)
                }
                frame 3 {
                  n1297 = control-ref of="Zone Thermocouples"() -> (w2642:refnum<vi>)
                  n1298 = control-ref of="Max Temp Slope"() -> (w2637:refnum<vi>)
                  n1299 = control-ref of="Temperature Goal"() -> (w2640:refnum<vi>)
                  n1300 = control-ref of="Max Allowable Temp"() -> (w2639:refnum<vi>)
                  n1301 = control-ref of="Temperature Calculation"() -> (w2641:refnum<vi>)
                  n1302 = control-ref of="Min Allowable Temp"() -> (w2638:refnum<vi>)
                }
                frame 4 {
                  n1303 = control-ref of="Zone Thermocouples"() -> (w2648:refnum<vi>)
                  n1304 = control-ref of="Max Temp Slope"() -> (w2643:refnum<vi>)
                  n1305 = control-ref of="Temperature Goal"() -> (w2646:refnum<vi>)
                  n1306 = control-ref of="Max Allowable Temp"() -> (w2645:refnum<vi>)
                  n1307 = control-ref of="Temperature Calculation"() -> (w2647:refnum<vi>)
                  n1308 = control-ref of="Min Allowable Temp"() -> (w2644:refnum<vi>)
                }
                frame 5 {
                  n1309 = control-ref of="Zone Thermocouples"() -> (w2654:refnum<vi>)
                  n1310 = control-ref of="Max Temp Slope"() -> (w2649:refnum<vi>)
                  n1311 = control-ref of="Temperature Goal"() -> (w2652:refnum<vi>)
                  n1312 = control-ref of="Max Allowable Temp"() -> (w2651:refnum<vi>)
                  n1313 = control-ref of="Temperature Calculation"() -> (w2653:refnum<vi>)
                  n1314 = control-ref of="Min Allowable Temp"() -> (w2650:refnum<vi>)
                }
                frame 6 {
                  n1315 = control-ref of="Zone Thermocouples"() -> (w2660:refnum<vi>)
                  n1316 = control-ref of="Temperature Goal"() -> (w2658:refnum<vi>)
                  n1317 = control-ref of="Max Temp Slope"() -> (w2655:refnum<vi>)
                  n1318 = control-ref of="Max Allowable Temp"() -> (w2657:refnum<vi>)
                  n1319 = control-ref of="Temperature Calculation"() -> (w2659:refnum<vi>)
                  n1320 = control-ref of="Min Allowable Temp"() -> (w2656:refnum<vi>)
                }
                frame 7 {
                  n1321 = control-ref of="Zone Thermocouples"() -> (w2666:refnum<vi>)
                  n1322 = control-ref of="Temperature Goal"() -> (w2664:refnum<vi>)
                  n1323 = control-ref of="Max Temp Slope"() -> (w2661:refnum<vi>)
                  n1324 = control-ref of="Max Allowable Temp"() -> (w2663:refnum<vi>)
                  n1325 = control-ref of="Temperature Calculation"() -> (w2665:refnum<vi>)
                  n1326 = control-ref of="Min Allowable Temp"() -> (w2662:refnum<vi>)
                }
                frame 8 {
                  n1327 = control-ref of="Zone Thermocouples"() -> (w2672:refnum<vi>)
                  n1328 = control-ref of="Temperature Goal"() -> (w2670:refnum<vi>)
                  n1329 = control-ref of="Max Temp Slope"() -> (w2667:refnum<vi>)
                  n1330 = control-ref of="Max Allowable Temp"() -> (w2669:refnum<vi>)
                  n1331 = control-ref of="Temperature Calculation"() -> (w2671:refnum<vi>)
                  n1332 = control-ref of="Min Allowable Temp"() -> (w2668:refnum<vi>)
                }
              }
              n1333 = To Long Integer(number=w2597) -> (32bit integer=w2596:i32)
              n1334 = property class="Arr (strict)"(reference=w2588) -> ("Value"=w2589:dbl[][])  [unwired: 1 in, 2 out]
              n1335 = Initialize Array(T23 {"thermalsetpoint"=0, "tempgoal"=0, "ramp"=0, "soakduration"=0} ("thermalprofiles"), w2596) -> (w2600:T34)
              n1336 = property class="LstBox (strict)"(reference=w2593) -> ("Item Symbols"=w2594:i32[])  [unwired: 1 in, 2 out]
              n1337 = property class="Str"(reference=w2578) -> ("Value"=w2577:string)  [unwired: 1 in, 2 out]
              n1338 = Fract/Exp String To Number(string=w2577) -> (number=w2576:dbl)  [unwired: 3 in, 1 out]
              n1339 = control-ref of="RampSoakTimes"() -> (w2590:refnum<vi>)
              n1340 = Array Size(array=w2594) -> (size(s)=w2595:i32)
              n1341 = for {
                N: w2595 -> [_]
                tunnel: w2594 -> [w2614]
                shift-right: [w2610] -> w2591
                shift-left: i32[] [] -> [w2609]
                i -> [w2608]
                n1342 = Index Array(array=w2614, index=w2608) -> (element=w2612:i32)
                n1343 = Equal?(x=w2612, y=38) -> (x = y?=w2613:bool)
                n1344 = case shown="True" w2613 {
                  tunnel: w2608 -> [_ w2618]
                  tunnel: [w2615 w2616] -> w2610
                  tunnel: w2609 -> [w2615 w2617]
                  frame False {
                  }
                  frame True {
                    n1345 = Build Array (concatenate)(w2617, w2618) -> (w2616:i32[])
                  }
                }
              }
              n1346 = property class="Ring (strict)"(reference=w2598) -> ("Value"=w2575:u16)  [unwired: 1 in, 2 out]
              n1347 = property class="Str"(reference=w2582) -> ("Value"=w2584:string)  [unwired: 1 in, 2 out]
              n1348 = property class="Str"(reference=w2583) -> ("Value"=w2585:string)  [unwired: 1 in, 2 out]
              n1349 = property class="Arr (strict)"(reference=w2590) -> ("Value"=w2587:dbl[][])  [unwired: 1 in, 2 out]
              n1350 = for {
                N: w2596 -> [_]
                tunnel: w2589 -> [w2681]
                tunnel: T23 {"thermalsetpoint"=0, "tempgoal"=0, "ramp"=0, "soakduration"=0} ("thermalprofiles") -> [w2692]
                shift-right: [w2690] -> w2586
                shift-left: w2600 -> [w2691]
                tunnel: w2587 -> [w2683]
                i -> [w2686]
                w2675 = 60.0 ("y")
                n1351 = Index Array(array=w2681, index (row)=w2686) -> (element=w2680:dbl[])  [unwired: 1 in]
                n1352 = Index Array(array=w2683, index (row)=w2686) -> (element=w2682:dbl[])  [unwired: 1 in]
                n1353 = Index Array(array=w2680, index #1=0 ("index (row)"), index #2=1 ("index (row)")) -> (element #1=w2679:dbl, element #2=w2678:dbl)
                n1354 = Index Array(array=w2682, index #1=1 ("index (row)"), index #2=2 ("index (row)")) -> (element #1=w2676:dbl, element #2=w2677:dbl)
                n1355 = Multiply(x=w2677, y=w2675) -> (x*y=w2673:dbl)
                n1356 = Multiply(x=w2676, y=w2675) -> (x*y=w2674:dbl)
                n1357 = Bundle By Name(cluster=w2692, "thermalsetpoint"=w2679, "tempgoal"=w2678, "ramp"=w2674, "soakduration"=w2673) -> (w2689:T23)
                n1358 = Replace Array Subset(array=w2691, new element=w2689, index=w2686) -> (w2690:T34)
              }
              n1359 = Decimal String To Number(string=w2585) -> (number=w2581:i32)  [unwired: 2 in, 1 out]
              n1360 = Decimal String To Number(string=w2584) -> (number=w2580:i32)  [unwired: 2 in, 1 out]
              n1361 = case shown="0, Default" w2575 {
                tunnel: ["Average" "Min" "Max"] -> w2574
                frame 0, Default {
                }
                frame 1 {
                }
                frame 2 {
                }
              }
              n1362 = Bundle By Name(cluster=T22 {"zone"=0, "average"="", "thermocouples"=[0], "maxTemp"=0, "minTemp"=0, "maxSlope"=0.0, "thermalprofiles"=[{"thermalsetpoint"=0, "tempgoal"=0, "ramp"=0, "soakduration"=0}]} ("ThermalProfileCluster.profiles"), "zone"=w2604, "average"=w2574, "thermocouples"=w2591, "maxTemp"=w2581, "minTemp"=w2580, "maxSlope"=w2576, "thermalprofiles"=w2586) -> (w2571:T22)
              n1363 = local write "profilearray"(dbl[][] []) -> ()
              n1364 = Build Array (concatenate)(w2573, w2571) -> (w2572:T32)
            }
          }
        }
        n1365 = case shown="True" "TVAC Labview" {
          tunnel: [path "C:/Users/stefan/AppData/Local/conda/conda/envs/py35/python.exe" ("Path to Python.exe") path "C:/Users/TVAC-admin/AppData/Local/Programs/Python/Python35/python.exe" ("Path to Python.exe")] -> w2408
          frame False {
          }
          frame True {
          }
        }
        n1366 = control-ref of="Thermal Profile Name"() -> (w2407:refnum<vi>)
        n1367 = Delete From Array(array=w2426, index=0) -> (array with subset deleted=w2424:T32)  [unwired: 1 in, 1 out]
        n1368 = property on="Property Node" class="Str"(reference=w2407) -> ("Text.Text"=w2374:string)  [unwired: 1 in, 2 out]
        n1369 = Bundle By Name(cluster=w2404, "ZoneProfile.profiles"=w2424, "ZoneSetup.Thermal Profile Name"=w2374) -> (w2380:T17)
        n1370 = local write "Current Profile Name"(w2374) -> ()
        n1371 = Flatten To JSON(anything=w2424, error in (no error)=w2375) -> (JSON string=w2421:string, 11:w2423:errorcluster)  [unwired: 1 in]
        n1372 = Unbundle By Name(w2404) -> ("ZonesSelected"=w2403:bool[])
        n1373 = case shown="False" "TVAC Labview" {
          tunnel: [path "C:/Users/stefan/Documents/GitHub/TVAC/head/Labview2017/TVAC_GUI/TestScripts/graph.json" ("file path (use dialog)") path "C:/Users/TVAC-admin/Documents/TVAC_Github/head/Labview2017/TVAC_GUI/TestScripts/graph.json" ("file path (use dialog)")] -> w2419
          frame False {
          }
          frame True {
          }
        }
        n1374 = local read "profilearray"() -> (w2390:dbl[][])
        n1375 = Open/Create/Replace File(file path (use dialog)=w2419, error in=w2423, operation (0:open)=T21."replace or create") -> (refnum out=w2422:refnum<file>, error out=w2420:errorcluster)  [unwired: 3 in, 1 out]
        n1376 = Write to Text File(file (use dialog)=w2422, text=w2421, error in=w2420) -> (refnum out=w2418:refnum<file>, error out=w2386:errorcluster)  [unwired: 1 in, 1 out]
        n1377 = Close File(refnum=w2418, error in=w2386) -> (error out=w2389:errorcluster)  [unwired: 1 out]
        n1378 = Unbundle By Name(w2380) -> ("TCs"=w2379:T14)
        n1379 = Flatten To JSON(anything=w2379) -> (JSON string=w2378:string)  [unwired: 2 in, 1 out]
        n1380 = case shown="False" "TVAC Labview" {
          tunnel: [path "C:/Users/stefan/Documents/GitHub/TVAC/head/Labview2017/TVAC_GUI/TestScripts/currentTC.json" ("file path (use dialog)") path "C:/Users/TVAC-admin/Documents/TVAC_Github/head/Labview2017/TVAC_GUI/TestScripts/currentTC.json" ("file path (use dialog)")] -> w2377
          frame False {
          }
          frame True {
          }
        }
        n1381 = Open/Create/Replace File(file path (use dialog)=w2377, error in=w2389, operation (0:open)=T21."replace or create") -> (refnum out=w2383:refnum<file>, error out=w2388:errorcluster)  [unwired: 3 in, 1 out]
        n1382 = Write to Text File(file (use dialog)=w2383, text=w2378, error in=w2388) -> (refnum out=w2382:refnum<file>, error out=w2387:errorcluster)  [unwired: 1 in, 1 out]
        n1383 = Close File(refnum=w2382, error in=w2387) -> (error out=w2385:errorcluster)  [unwired: 1 out]
        n1384 = call "lvGraphProfile.vi"("pathToJson"=w2419, "error in (no error)"=w2385, "pathToJson 2"=w2377, "Path to Python.exe"=w2408, "RunCount"=w2394) -> ("graphCluster"=w2405:T35, "Raw Python String Output"=w2392:string, "error out"=w2409:errorcluster)  [unwired: 8 in]
        n1385 = Unbundle By Name(w2405) -> ("time"=w2402:dbl[])
        n1386 = local write "Thermal Profile Compiling Summary"(w2392) -> ()
        n1387 = Concatenate Strings("Thermal Profile : ", w2374) -> (w2398:string)
        n1388 = for {
          N: 9 -> [_]
          tunnel: w2405 -> [w2457]
          tunnel: w2403 -> [_] mode=indexing
          shift-right: [w2458] -> w2401
          shift-left: w2402 -> [w2458]
          tunnel: w2398 -> [w2456]
          shift-right: [w2455] -> w2391
          shift-left: w2390 -> [w2452]
          i -> [w2453]
          n1389 = Equal To 0?(x=w2453) -> (x = 0?=w2454:bool)
          n1390 = case shown="True" w2454 {
            tunnel: w2452 -> [w2459 _]
            tunnel: [w2459 dbl[][] [] ("profilearray")] -> w2451
            frame False {
            }
            frame True {
            }
          }
          n1391 = case shown="8" w2453 {
            tunnel: w2457 -> [w2466 w2476 w2486 w2496 w2506 w2516 w2526 w2536 w2547]
            tunnel: w2456 -> [_ _ _ _ _ _ _ _ w2543]
            tunnel: [w2462 w2472 w2482 w2492 w2502 w2512 w2522 w2532 w2542] -> w2455
            tunnel: w2451 -> [w2461 w2471 w2481 w2491 w2501 w2511 w2521 w2531 w2541]
            frame 0, Default {
              n1392 = Unbundle By Name(w2466) -> ("zone1"=w2465:dbl[])
              n1393 = Index Array(array=w2465) -> (element=w2463:dbl)  [unwired: 1 in]
              n1394 = Not Equal To 0?(x=w2463) -> (x != 0?=w2464:bool)
              n1395 = case shown="True" w2464 {
                tunnel: w2465 -> [_ w2469]
                tunnel: [w2467 w2468] -> w2462
                tunnel: w2461 -> [w2467 _]
                frame False {
                }
                frame True {
                  n1396 = local read "profilearray"() -> (w2470:dbl[][])
                  n1397 = Build Array (concatenate)(w2470, w2469) -> (w2468:dbl[][])
                  n1398 = local write "profilearray"(w2468) -> ()
                }
              }
            }
            frame 1 {
              n1399 = Unbundle By Name(w2476) -> ("zone2"=w2475:dbl[])
              n1400 = Index Array(array=w2475) -> (element=w2473:dbl)  [unwired: 1 in]
              n1401 = Not Equal To 0?(x=w2473) -> (x != 0?=w2474:bool)
              n1402 = case shown="False" w2474 {
                tunnel: w2475 -> [_ w2479]
                tunnel: [w2477 w2478] -> w2472
                tunnel: w2471 -> [w2477 _]
                frame False {
                }
                frame True {
                  n1403 = local read "profilearray"() -> (w2480:dbl[][])
                  n1404 = Build Array (concatenate)(w2480, w2479) -> (w2478:dbl[][])
                  n1405 = local write "profilearray"(w2478) -> ()
                }
              }
            }
            frame 2 {
              n1406 = Unbundle By Name(w2486) -> ("zone3"=w2485:dbl[])
              n1407 = Index Array(array=w2485) -> (element=w2483:dbl)  [unwired: 1 in]
              n1408 = Not Equal To 0?(x=w2483) -> (x != 0?=w2484:bool)
              n1409 = case shown="True" w2484 {
                tunnel: w2485 -> [_ w2489]
                tunnel: [w2487 w2488] -> w2482
                tunnel: w2481 -> [w2487 _]
                frame False {
                }
                frame True {
                  n1410 = local read "profilearray"() -> (w2490:dbl[][])
                  n1411 = Build Array (concatenate)(w2490, w2489) -> (w2488:dbl[][])
                  n1412 = local write "profilearray"(w2488) -> ()
                }
              }
            }
            frame 3 {
              n1413 = Unbundle By Name(w2496) -> ("zone4"=w2495:dbl[])
              n1414 = Index Array(array=w2495) -> (element=w2493:dbl)  [unwired: 1 in]
              n1415 = Not Equal To 0?(x=w2493) -> (x != 0?=w2494:bool)
              n1416 = case shown="True" w2494 {
                tunnel: w2495 -> [_ w2499]
                tunnel: [w2497 w2498] -> w2492
                tunnel: w2491 -> [w2497 _]
                frame False {
                }
                frame True {
                  n1417 = local read "profilearray"() -> (w2500:dbl[][])
                  n1418 = Build Array (concatenate)(w2500, w2499) -> (w2498:dbl[][])
                  n1419 = local write "profilearray"(w2498) -> ()
                }
              }
            }
            frame 4 {
              n1420 = Unbundle By Name(w2506) -> ("zone5"=w2505:dbl[])
              n1421 = Index Array(array=w2505) -> (element=w2503:dbl)  [unwired: 1 in]
              n1422 = Not Equal To 0?(x=w2503) -> (x != 0?=w2504:bool)
              n1423 = case shown="True" w2504 {
                tunnel: w2505 -> [_ w2509]
                tunnel: [w2507 w2508] -> w2502
                tunnel: w2501 -> [w2507 _]
                frame False {
                }
                frame True {
                  n1424 = local read "profilearray"() -> (w2510:dbl[][])
                  n1425 = Build Array (concatenate)(w2510, w2509) -> (w2508:dbl[][])
                  n1426 = local write "profilearray"(w2508) -> ()
                }
              }
            }
            frame 5 {
              n1427 = Unbundle By Name(w2516) -> ("zone6"=w2515:dbl[])
              n1428 = Index Array(array=w2515) -> (element=w2513:dbl)  [unwired: 1 in]
              n1429 = Not Equal To 0?(x=w2513) -> (x != 0?=w2514:bool)
              n1430 = case shown="False" w2514 {
                tunnel: w2515 -> [_ w2519]
                tunnel: [w2517 w2518] -> w2512
                tunnel: w2511 -> [w2517 _]
                frame False {
                }
                frame True {
                  n1431 = local read "profilearray"() -> (w2520:dbl[][])
                  n1432 = Build Array (concatenate)(w2520, w2519) -> (w2518:dbl[][])
                  n1433 = local write "profilearray"(w2518) -> ()
                }
              }
            }
            frame 6 {
              n1434 = Unbundle By Name(w2526) -> ("zone7"=w2525:dbl[])
              n1435 = Index Array(array=w2525) -> (element=w2523:dbl)  [unwired: 1 in]
              n1436 = Not Equal To 0?(x=w2523) -> (x != 0?=w2524:bool)
              n1437 = case shown="True" w2524 {
                tunnel: w2525 -> [_ w2529]
                tunnel: [w2527 w2528] -> w2522
                tunnel: w2521 -> [w2527 _]
                frame False {
                }
                frame True {
                  n1438 = local read "profilearray"() -> (w2530:dbl[][])
                  n1439 = Build Array (concatenate)(w2530, w2529) -> (w2528:dbl[][])
                  n1440 = local write "profilearray"(w2528) -> ()
                }
              }
            }
            frame 7 {
              n1441 = Unbundle By Name(w2536) -> ("zone8"=w2535:dbl[])
              n1442 = Index Array(array=w2535) -> (element=w2533:dbl)  [unwired: 1 in]
              n1443 = Not Equal To 0?(x=w2533) -> (x != 0?=w2534:bool)
              n1444 = case shown="True" w2534 {
                tunnel: w2535 -> [_ w2539]
                tunnel: [w2537 w2538] -> w2532
                tunnel: w2531 -> [w2537 _]
                frame False {
                }
                frame True {
                  n1445 = local read "profilearray"() -> (w2540:dbl[][])
                  n1446 = Build Array (concatenate)(w2540, w2539) -> (w2538:dbl[][])
                  n1447 = local write "profilearray"(w2538) -> ()
                }
              }
            }
            frame 8 {
              n1448 = Unbundle By Name(w2547) -> ("zone9"=w2546:dbl[])
              n1449 = Index Array(array=w2546) -> (element=w2544:dbl)  [unwired: 1 in]
              n1450 = Not Equal To 0?(x=w2544) -> (x != 0?=w2545:bool)
              n1451 = case shown="True" w2545 {
                tunnel: w2546 -> [_ w2550]
                tunnel: [w2548 w2549] -> w2542
                tunnel: w2541 -> [w2548 _]
                frame False {
                }
                frame True {
                  n1452 = local read "profilearray"() -> (w2551:dbl[][])
                  n1453 = Build Array (concatenate)(w2551, w2550) -> (w2549:dbl[][])
                  n1454 = local write "profilearray"(w2549) -> ()
                }
              }
              "ThermalProfileStatus" <- w2543
            }
          }
        }
        n1455 = Index Array(array=w2401, index=1) -> (element=w2400:dbl)
        n1456 = Index Array(array=w2401, index=0) -> (element=w2410:dbl)
        n1457 = Subtract(x=w2400, y=w2410) -> (x-y=w2415:dbl)
        n1458 = Divide(x=w2415, y=60.0) -> (x/y=w2413:dbl)
        n1459 = Bundle(0.0, w2413, "profilearray"=w2391) -> (→"Thermal Profile":cluster{dbl, dbl, "profilearray":dbl[][]})  [unwired: 1 in]
      }
      frame "importProfile" {
        n1460 = control-ref of="Import CSV as a Thermal Profile"() -> (w2694:refnum<vi>)
        n1461 = property class="Path"(reference=w2694) -> ("Value"=w2693:path)  [unwired: 1 in, 2 out]
        n1462 = property on="Import CSV as a Thermal Profile" class="Path"() -> ("Text.Text"=w2728:string)  [unwired: 2 in, 2 out]
        n1463 = call-poly <vilib>:"Read Delimited Spreadsheet.vi"("file path (dialog if empty)"=w2693, "delimiter (\\t)"="," ("delimiter (\\t)")) -> ("all rows"=w2713:string[][])  [unwired: 8 in, 5 out]
        n1464 = Array Size(array=w2713) -> (size(s)=w2732:i32[])
        n1465 = Index Array(array=w2732, index=0) -> (element=w2714:i32)
        n1466 = Spreadsheet String To Array(delimiter (Tab)="\\", format string="%s", spreadsheet string=w2728, array type (2D Dbl)=string[][] []) -> (array=w2723:string[][])
        n1467 = for {
          N: w2714 -> [_]
          shift-right: [w2767] -> w2712
          shift-left: w2713 -> [w2768]
          shift-right: [w2759] -> w2709
          shift-left: "LastSetPt" -> [w2758]
          i -> [w2763]
          n1468 = Add(x=7 ("y"), y=w2763) -> (x+y=w2762:i32)
          n1469 = Subtract(x=w2762, y=6) -> (x-y=w2760:i32)
          n1470 = Index Array(array=w2768, index (row)=w2762, index (col)=0 ("disabled index (col)")) -> (element=w2769:string)
          n1471 = Number To Decimal String(number=w2760) -> (decimal integer string=w2761:string)  [unwired: 1 in]
          n1472 = Equal?(x=w2769, y=w2761) -> (x = y?=w2766:bool)
          n1473 = case shown="True" w2766 {
            tunnel: w2768 -> [w2772 w2774]
            tunnel: [w2772 w2774] -> w2767
            tunnel: w2760 -> [_ w2773]
            tunnel: [w2771 w2773] -> w2759
            tunnel: w2758 -> [w2771 _]
            frame False {
            }
            frame True {
              n1474 = local write "LastSetPt"(w2773) -> ()
            }
          }
        }
        n1475 = Array Size(array=w2723) -> (size(s)=w2722:i32[])
        n1476 = Bundle By Name(cluster=w2695, "tprofilesheet"=w2713) -> (w2738:T17)
        n1477 = local write "tprofilesheet"(w2713) -> ()
        n1478 = Index Array(array=w2713, index (row)=1) -> (element=w2739:string[])  [unwired: 1 in]
        n1479 = Index Array(array=w2713, index (row)=2) -> (element=w2735:string[])  [unwired: 1 in]
        n1480 = Index Array(array=w2722, index=1) -> (element=w2720:i32)
        n1481 = Decrement(x=w2720) -> (x-1=w2719:i32)
        n1482 = Index Array(array=w2723, index (row)=0, index (col)=w2719) -> (element=w2718:string)
        n1483 = Match Pattern(string=w2718, regular expression=".csv") -> (before substring=w2715:string)  [unwired: 1 in, 3 out]
        n1484 = Unbundle By Name(w2738) -> ("ZoneSetup.Zone Selection"=w2737:i32[])
        n1485 = To Double Precision Float(number=w2709) -> (double precision float=w2729:dbl)
        n1486 = for {
          N: 9 -> [_]
          shift-right: [w2803] -> w2736
          shift-left: w2738 -> [w2816]
          tunnel: w2739 -> [w2815] mode=indexing
          shift-right: [w2813] -> w2733
          shift-left: w2737 -> [w2814]
          tunnel: w2735 -> [w2807]
          tunnel: w2712 -> [w2788]
          tunnel: w2709 -> [w2778]
          i -> [w2784]
          n1487 = case shown="0, Default" w2784 {
            selector: w2784 -> [w2911 w2946 w2981 w3016 w3051 w3086 w3121 w3156 w3191]
            tunnel: w2816 -> [w2915 w2950 w2985 w3020 w3055 w3090 w3125 w3160 w3195]
            tunnel: [w2914 w2949 w2984 w3019 w3054 w3089 w3124 w3159 w3194] -> w2804
            tunnel: w2815 -> [w2913 w2948 w2983 w3018 w3053 w3088 w3123 w3158 w3193]
            tunnel: w2814 -> [w2912 w2947 w2982 w3017 w3052 w3087 w3122 w3157 w3192]
            tunnel: [w2910 w2945 w2980 w3015 w3050 w3085 w3120 w3155 w3190] -> w2813
            tunnel: [w2909 w2944 w2979 w3014 w3049 w3084 w3119 w3154 w3189] -> w2776
            tunnel: [w2908 w2943 w2978 w3013 w3048 w3083 w3118 w3153 w3188] -> w2801
            tunnel: [w2905 w2940 w2975 w3010 w3045 w3080 w3115 w3150 w3185] -> w2802
            tunnel: [w2903 w2938 w2973 w3008 w3043 w3078 w3113 w3148 w3183] -> w2780
            tunnel: [w2902 w2937 w2972 w3007 w3042 w3077 w3112 w3147 w3182] -> w2789
            tunnel: [w2901 w2936 w2971 w3006 w3041 w3076 w3111 w3146 w3181] -> w2779
            frame 0, Default {
              n1488 = control-ref of="Thermocouples Selected"() -> (w2905:refnum<vi>)
              n1489 = case shown="\"Min\"" w2913 {
                tunnel: [2 1 0 0] -> w2906
                tunnel: w2912 -> [w2919 w2924 w2929 w2934]
                tunnel: w2911 -> [w2918 w2923 w2928 w2933]
                tunnel: [w2917 w2922 w2927 w2932] -> w2910
                frame "Max" {
                  n1490 = Replace Array Subset(array=w2919, new element=38, index=w2918) -> (w2917:i32[])
                }
                frame "Min" {
                  n1491 = Replace Array Subset(array=w2924, new element=38, index=w2923) -> (w2922:i32[])
                }
                frame "Average" {
                  n1492 = Replace Array Subset(array=w2929, new element=38, index=w2928) -> (w2927:i32[])
                }
                frame "", Default {
                  n1493 = Replace Array Subset(array=w2934, new element=37, index=w2933) -> (w2932:i32[])
                }
              }
              n1494 = control-ref of="Max Temp Slope"() -> (w2903:refnum<vi>)
              n1495 = property class="Str"(reference=w2905, "Text.Text"="") -> ()  [unwired: 1 in, 2 out]
              n1496 = control-ref of="Min Allowable Temp"() -> (w2902:refnum<vi>)
              n1497 = control-ref of="Zone Thermocouples"() -> (w2908:refnum<vi>)
              n1498 = property class="LstBox (strict)"(reference=w2908) -> ("Item Symbols"=w2909:i32[])  [unwired: 1 in, 2 out]
              n1499 = control-ref of="Max Allowable Temp"() -> (w2901:refnum<vi>)
              n1500 = Bundle By Name(cluster=w2915, "Zone 1.Temperature Calculation"=w2906) -> (w2914:T17)
              n1501 = control-ref of="Temperature Calculation"() -> (w2907:refnum<vi>)
              n1502 = property class="Ring (strict)"(reference=w2907, "Value"=w2906) -> ()  [unwired: 1 in, 2 out]
            }
            frame 1 {
              n1503 = control-ref of="Thermocouples Selected"() -> (w2940:refnum<vi>)
              n1504 = case shown="\"Min\"" w2948 {
                tunnel: [2 1 0 0] -> w2941
                tunnel: w2947 -> [w2954 w2959 w2964 w2969]
                tunnel: w2946 -> [w2953 w2958 w2963 w2968]
                tunnel: [w2952 w2957 w2962 w2967] -> w2945
                frame "Max" {
                  n1505 = Replace Array Subset(array=w2954, new element=38, index=w2953) -> (w2952:i32[])
                }
                frame "Min" {
                  n1506 = Replace Array Subset(array=w2959, new element=38, index=w2958) -> (w2957:i32[])
                }
                frame "Average" {
                  n1507 = Replace Array Subset(array=w2964, new element=38, index=w2963) -> (w2962:i32[])
                }
                frame "", Default {
                  n1508 = Replace Array Subset(array=w2969, new element=37, index=w2968) -> (w2967:i32[])
                }
              }
              n1509 = control-ref of="Max Temp Slope"() -> (w2938:refnum<vi>)
              n1510 = property class="Str"(reference=w2940, "Text.Text"="") -> ()  [unwired: 1 in, 2 out]
              n1511 = control-ref of="Min Allowable Temp"() -> (w2937:refnum<vi>)
              n1512 = control-ref of="Zone Thermocouples"() -> (w2943:refnum<vi>)
              n1513 = property class="LstBox (strict)"(reference=w2943) -> ("Item Symbols"=w2944:i32[])  [unwired: 1 in, 2 out]
              n1514 = control-ref of="Max Allowable Temp"() -> (w2936:refnum<vi>)
              n1515 = Bundle By Name(cluster=w2950, "Zone 2.Temperature Calculation"=w2941) -> (w2949:T17)
              n1516 = control-ref of="Temperature Calculation"() -> (w2942:refnum<vi>)
              n1517 = property class="Ring (strict)"(reference=w2942, "Value"=w2941) -> ()  [unwired: 1 in, 2 out]
            }
            frame 2 {
              n1518 = control-ref of="Thermocouples Selected"() -> (w2975:refnum<vi>)
              n1519 = case shown="\"Min\"" w2983 {
                tunnel: [2 1 0 0] -> w2976
                tunnel: w2982 -> [w2989 w2994 w2999 w3004]
                tunnel: w2981 -> [w2988 w2993 w2998 w3003]
                tunnel: [w2987 w2992 w2997 w3002] -> w2980
                frame "Max" {
                  n1520 = Replace Array Subset(array=w2989, new element=38, index=w2988) -> (w2987:i32[])
                }
                frame "Min" {
                  n1521 = Replace Array Subset(array=w2994, new element=38, index=w2993) -> (w2992:i32[])
                }
                frame "Average" {
                  n1522 = Replace Array Subset(array=w2999, new element=38, index=w2998) -> (w2997:i32[])
                }
                frame "", Default {
                  n1523 = Replace Array Subset(array=w3004, new element=37, index=w3003) -> (w3002:i32[])
                }
              }
              n1524 = control-ref of="Max Temp Slope"() -> (w2973:refnum<vi>)
              n1525 = property class="Str"(reference=w2975, "Text.Text"="") -> ()  [unwired: 1 in, 2 out]
              n1526 = control-ref of="Min Allowable Temp"() -> (w2972:refnum<vi>)
              n1527 = control-ref of="Zone Thermocouples"() -> (w2978:refnum<vi>)
              n1528 = property class="LstBox (strict)"(reference=w2978) -> ("Item Symbols"=w2979:i32[])  [unwired: 1 in, 2 out]
              n1529 = control-ref of="Max Allowable Temp"() -> (w2971:refnum<vi>)
              n1530 = Bundle By Name(cluster=w2985, "Zone 3.Temperature Calculation"=w2976) -> (w2984:T17)
              n1531 = control-ref of="Temperature Calculation"() -> (w2977:refnum<vi>)
              n1532 = property class="Ring (strict)"(reference=w2977, "Value"=w2976) -> ()  [unwired: 1 in, 2 out]
            }
            frame 3 {
              n1533 = control-ref of="Thermocouples Selected"() -> (w3010:refnum<vi>)
              n1534 = case shown="\"Min\"" w3018 {
                tunnel: [2 1 0 0] -> w3011
                tunnel: w3017 -> [w3024 w3029 w3034 w3039]
                tunnel: w3016 -> [w3023 w3028 w3033 w3038]
                tunnel: [w3022 w3027 w3032 w3037] -> w3015
                frame "Max" {
                  n1535 = Replace Array Subset(array=w3024, new element=38, index=w3023) -> (w3022:i32[])
                }
                frame "Min" {
                  n1536 = Replace Array Subset(array=w3029, new element=38, index=w3028) -> (w3027:i32[])
                }
                frame "Average" {
                  n1537 = Replace Array Subset(array=w3034, new element=38, index=w3033) -> (w3032:i32[])
                }
                frame "", Default {
                  n1538 = Replace Array Subset(array=w3039, new element=37, index=w3038) -> (w3037:i32[])
                }
              }
              n1539 = control-ref of="Max Temp Slope"() -> (w3008:refnum<vi>)
              n1540 = property class="Str"(reference=w3010, "Text.Text"="") -> ()  [unwired: 1 in, 2 out]
              n1541 = control-ref of="Min Allowable Temp"() -> (w3007:refnum<vi>)
              n1542 = control-ref of="Zone Thermocouples"() -> (w3013:refnum<vi>)
              n1543 = property class="LstBox (strict)"(reference=w3013) -> ("Item Symbols"=w3014:i32[])  [unwired: 1 in, 2 out]
              n1544 = control-ref of="Max Allowable Temp"() -> (w3006:refnum<vi>)
              n1545 = Bundle By Name(cluster=w3020, "Zone 4.Temperature Calculation"=w3011) -> (w3019:T17)
              n1546 = control-ref of="Temperature Calculation"() -> (w3012:refnum<vi>)
              n1547 = property class="Ring (strict)"(reference=w3012, "Value"=w3011) -> ()  [unwired: 1 in, 2 out]
            }
            frame 4 {
              n1548 = control-ref of="Thermocouples Selected"() -> (w3045:refnum<vi>)
              n1549 = case shown="\"Min\"" w3053 {
                tunnel: [2 1 0 0] -> w3046
                tunnel: w3052 -> [w3059 w3064 w3069 w3074]
                tunnel: w3051 -> [w3058 w3063 w3068 w3073]
                tunnel: [w3057 w3062 w3067 w3072] -> w3050
                frame "Max" {
                  n1550 = Replace Array Subset(array=w3059, new element=38, index=w3058) -> (w3057:i32[])
                }
                frame "Min" {
                  n1551 = Replace Array Subset(array=w3064, new element=38, index=w3063) -> (w3062:i32[])
                }
                frame "Average" {
                  n1552 = Replace Array Subset(array=w3069, new element=38, index=w3068) -> (w3067:i32[])
                }
                frame "", Default {
                  n1553 = Replace Array Subset(array=w3074, new element=37, index=w3073) -> (w3072:i32[])
                }
              }
              n1554 = control-ref of="Max Temp Slope"() -> (w3043:refnum<vi>)
              n1555 = property class="Str"(reference=w3045, "Text.Text"="") -> ()  [unwired: 1 in, 2 out]
              n1556 = control-ref of="Min Allowable Temp"() -> (w3042:refnum<vi>)
              n1557 = control-ref of="Zone Thermocouples"() -> (w3048:refnum<vi>)
              n1558 = property class="LstBox (strict)"(reference=w3048) -> ("Item Symbols"=w3049:i32[])  [unwired: 1 in, 2 out]
              n1559 = control-ref of="Max Allowable Temp"() -> (w3041:refnum<vi>)
              n1560 = Bundle By Name(cluster=w3055, "Zone 5.Temperature Calculation"=w3046) -> (w3054:T17)
              n1561 = control-ref of="Temperature Calculation"() -> (w3047:refnum<vi>)
              n1562 = property class="Ring (strict)"(reference=w3047, "Value"=w3046) -> ()  [unwired: 1 in, 2 out]
            }
            frame 5 {
              n1563 = control-ref of="Thermocouples Selected"() -> (w3080:refnum<vi>)
              n1564 = case shown="\"Min\"" w3088 {
                tunnel: [2 1 0 0] -> w3081
                tunnel: w3087 -> [w3094 w3099 w3104 w3109]
                tunnel: w3086 -> [w3093 w3098 w3103 w3108]
                tunnel: [w3092 w3097 w3102 w3107] -> w3085
                frame "Max" {
                  n1565 = Replace Array Subset(array=w3094, new element=38, index=w3093) -> (w3092:i32[])
                }
                frame "Min" {
                  n1566 = Replace Array Subset(array=w3099, new element=38, index=w3098) -> (w3097:i32[])
                }
                frame "Average" {
                  n1567 = Replace Array Subset(array=w3104, new element=38, index=w3103) -> (w3102:i32[])
                }
                frame "", Default {
                  n1568 = Replace Array Subset(array=w3109, new element=37, index=w3108) -> (w3107:i32[])
                }
              }
              n1569 = control-ref of="Max Temp Slope"() -> (w3078:refnum<vi>)
              n1570 = property class="Str"(reference=w3080, "Text.Text"="") -> ()  [unwired: 1 in, 2 out]
              n1571 = control-ref of="Min Allowable Temp"() -> (w3077:refnum<vi>)
              n1572 = control-ref of="Zone Thermocouples"() -> (w3083:refnum<vi>)
              n1573 = property class="LstBox (strict)"(reference=w3083) -> ("Item Symbols"=w3084:i32[])  [unwired: 1 in, 2 out]
              n1574 = control-ref of="Max Allowable Temp"() -> (w3076:refnum<vi>)
              n1575 = Bundle By Name(cluster=w3090, "Zone 6.Temperature Calculation"=w3081) -> (w3089:T17)
              n1576 = control-ref of="Temperature Calculation"() -> (w3082:refnum<vi>)
              n1577 = property class="Ring (strict)"(reference=w3082, "Value"=w3081) -> ()  [unwired: 1 in, 2 out]
            }
            frame 6 {
              n1578 = control-ref of="Thermocouples Selected"() -> (w3115:refnum<vi>)
              n1579 = case shown="\"Average\"" w3123 {
                tunnel: [2 1 0 0] -> w3116
                tunnel: w3122 -> [w3129 w3134 w3139 w3144]
                tunnel: w3121 -> [w3128 w3133 w3138 w3143]
                tunnel: [w3127 w3132 w3137 w3142] -> w3120
                frame "Max" {
                  n1580 = Replace Array Subset(array=w3129, new element=38, index=w3128) -> (w3127:i32[])
                }
                frame "Min" {
                  n1581 = Replace Array Subset(array=w3134, new element=38, index=w3133) -> (w3132:i32[])
                }
                frame "Average" {
                  n1582 = Replace Array Subset(array=w3139, new element=38, index=w3138) -> (w3137:i32[])
                }
                frame "", Default {
                  n1583 = Replace Array Subset(array=w3144, new element=37, index=w3143) -> (w3142:i32[])
                }
              }
              n1584 = control-ref of="Max Temp Slope"() -> (w3113:refnum<vi>)
              n1585 = property class="Str"(reference=w3115, "Text.Text"="") -> ()  [unwired: 1 in, 2 out]
              n1586 = control-ref of="Min Allowable Temp"() -> (w3112:refnum<vi>)
              n1587 = control-ref of="Zone Thermocouples"() -> (w3118:refnum<vi>)
              n1588 = property class="LstBox (strict)"(reference=w3118) -> ("Item Symbols"=w3119:i32[])  [unwired: 1 in, 2 out]
              n1589 = control-ref of="Max Allowable Temp"() -> (w3111:refnum<vi>)
              n1590 = Bundle By Name(cluster=w3125, "Zone 7.Temperature Calculation"=w3116) -> (w3124:T17)
              n1591 = control-ref of="Temperature Calculation"() -> (w3117:refnum<vi>)
              n1592 = property class="Ring (strict)"(reference=w3117, "Value"=w3116) -> ()  [unwired: 1 in, 2 out]
            }
            frame 7 {
              n1593 = control-ref of="Thermocouples Selected"() -> (w3150:refnum<vi>)
              n1594 = case shown="\"Min\"" w3158 {
                tunnel: [2 1 0 0] -> w3151
                tunnel: w3157 -> [w3164 w3169 w3174 w3179]
                tunnel: w3156 -> [w3163 w3168 w3173 w3178]
                tunnel: [w3162 w3167 w3172 w3177] -> w3155
                frame "Max" {
                  n1595 = Replace Array Subset(array=w3164, new element=38, index=w3163) -> (w3162:i32[])
                }
                frame "Min" {
                  n1596 = Replace Array Subset(array=w3169, new element=38, index=w3168) -> (w3167:i32[])
                }
                frame "Average" {
                  n1597 = Replace Array Subset(array=w3174, new element=38, index=w3173) -> (w3172:i32[])
                }
                frame "", Default {
                  n1598 = Replace Array Subset(array=w3179, new element=37, index=w3178) -> (w3177:i32[])
                }
              }
              n1599 = control-ref of="Max Temp Slope"() -> (w3148:refnum<vi>)
              n1600 = property class="Str"(reference=w3150, "Text.Text"="") -> ()  [unwired: 1 in, 2 out]
              n1601 = control-ref of="Min Allowable Temp"() -> (w3147:refnum<vi>)
              n1602 = control-ref of="Zone Thermocouples"() -> (w3153:refnum<vi>)
              n1603 = property class="LstBox (strict)"(reference=w3153) -> ("Item Symbols"=w3154:i32[])  [unwired: 1 in, 2 out]
              n1604 = control-ref of="Max Allowable Temp"() -> (w3146:refnum<vi>)
              n1605 = Bundle By Name(cluster=w3160, "Zone 8.Temperature Calculation"=w3151) -> (w3159:T17)
              n1606 = control-ref of="Temperature Calculation"() -> (w3152:refnum<vi>)
              n1607 = property class="Ring (strict)"(reference=w3152, "Value"=w3151) -> ()  [unwired: 1 in, 2 out]
            }
            frame 8 {
              n1608 = control-ref of="Thermocouples Selected"() -> (w3185:refnum<vi>)
              n1609 = case shown="\"Min\"" w3193 {
                tunnel: [2 1 0 0] -> w3186
                tunnel: w3192 -> [w3199 w3204 w3209 w3214]
                tunnel: w3191 -> [w3198 w3203 w3208 w3213]
                tunnel: [w3197 w3202 w3207 w3212] -> w3190
                frame "Max" {
                  n1610 = Replace Array Subset(array=w3199, new element=38, index=w3198) -> (w3197:i32[])
                }
                frame "Min" {
                  n1611 = Replace Array Subset(array=w3204, new element=38, index=w3203) -> (w3202:i32[])
                }
                frame "Average" {
                  n1612 = Replace Array Subset(array=w3209, new element=38, index=w3208) -> (w3207:i32[])
                }
                frame "", Default {
                  n1613 = Replace Array Subset(array=w3214, new element=37, index=w3213) -> (w3212:i32[])
                }
              }
              n1614 = control-ref of="Max Temp Slope"() -> (w3183:refnum<vi>)
              n1615 = property class="Str"(reference=w3185, "Text.Text"="") -> ()  [unwired: 1 in, 2 out]
              n1616 = control-ref of="Min Allowable Temp"() -> (w3182:refnum<vi>)
              n1617 = control-ref of="Zone Thermocouples"() -> (w3188:refnum<vi>)
              n1618 = property class="LstBox (strict)"(reference=w3188) -> ("Item Symbols"=w3189:i32[])  [unwired: 1 in, 2 out]
              n1619 = control-ref of="Max Allowable Temp"() -> (w3181:refnum<vi>)
              n1620 = Bundle By Name(cluster=w3195, "Zone 9.Temperature Calculation"=w3186) -> (w3194:T17)
              n1621 = control-ref of="Temperature Calculation"() -> (w3187:refnum<vi>)
              n1622 = property class="Ring (strict)"(reference=w3187, "Value"=w3186) -> ()  [unwired: 1 in, 2 out]
            }
          }
          n1623 = Index Array(array=w2807, index=w2784) -> (element=w2810:string)
          n1624 = call <vilib>:"Space Constant.vi"() -> ("String"=w2811:string)
          n1625 = Initialize Array("", w2778, 3 ("dimension size")) -> (w2793:string[][])
          n1626 = Spreadsheet String To Array(delimiter (Tab)=w2811, format string="%d", spreadsheet string=w2810) -> (array=w2812:dbl[][])  [unwired: 1 in]
          n1627 = Initialize Array("", w2778, 2 ("dimension size")) -> (w2800:string[][])
          n1628 = Index Array(array=w2812, index (row)=0) -> (element=w2806:dbl[])  [unwired: 1 in]
          n1629 = for {
            N: w2778 -> [_]
            tunnel: w2788 -> [w2838]
            shift-right: [w2835] -> w2797
            shift-left: w2800 -> [w2836]
            tunnel: w2784 -> [w2830]
            shift-right: [w2819] -> w2792
            shift-left: w2793 -> [w2820]
            i -> [w2822]
            n1630 = Add(x=3, y=w2830) -> (x+y=w2829:i32)
            n1631 = Add(x=7, y=w2822) -> (x+y=w2828:i32)
            n1632 = Index Array(array=w2838, index (row) #1=w2828, index (col) #1=0 ("disabled index (col)"), index (row) #2=w2828, index (col) #2=w2829, index (row) #3=w2828, index (col) #3=1 ("disabled index (col)"), index (row) #4=w2828, index (col) #4=2 ("disabled index (col)")) -> (element #1=w2825:string, element #2=w2833:string, element #3=w2824:string, element #4=w2823:string)
            n1633 = Build Array(w2825, w2833) -> (w2832:string[])
            n1634 = Build Array(w2825, w2824, w2823) -> (w2821:string[])
            n1635 = Replace Array Subset(array=w2836, new element=w2832, index (row)=w2822) -> (w2835:string[][])  [unwired: 1 in]
            n1636 = Replace Array Subset(array=w2820, new element=w2821, index (row)=w2822) -> (w2819:string[][])  [unwired: 1 in]
          }
          n1637 = To Long Integer(number=w2806) -> (32bit integer=w2805:i32[])
          n1638 = Array Size(array=w2805) -> (size(s)=w2777:i32)
          n1639 = for {
            N: w2777 -> [_]
            tunnel: w2805 -> [w2886] mode=indexing
            shift-right: [w2884] -> w2775
            shift-left: w2776 -> [w2885]
            tunnel: w2802 -> [w2889]
            n1640 = Not Equal To 0?(x=w2886) -> (x != 0?=w2888:bool)
            n1641 = case shown="True" w2888 {
              tunnel: w2886 -> [_ w2896]
              tunnel: w2889 -> [_ w2895]
              tunnel: 38 -> [_ w2894]
              tunnel: w2886 -> [_ w2893]
              tunnel: [w2890 w2892] -> w2884
              tunnel: w2885 -> [w2890 w2891]
              frame False {
              }
              frame True {
                n1642 = property class="Str"(reference=w2895) -> ("Text.Text"=w2900:string)  [unwired: 1 in, 2 out]
                n1643 = Number To Decimal String(number=w2896) -> (decimal integer string=w2897:string)  [unwired: 1 in]
                n1644 = call <vilib>:"Space Constant.vi"() -> ("String"=w2898:string)
                n1645 = Replace Array Subset(array=w2891, new element=w2894, index=w2893) -> (w2892:i32[])
                n1646 = Concatenate Strings(w2900, w2898, w2897) -> (w2899:string)
                n1647 = property class="Str"(reference=w2895, "Text.Text"=w2899) -> ()  [unwired: 1 in, 2 out]
              }
            }
          }
          n1648 = property class="LstBox (strict)"(reference=w2801, "Item Symbols"=w2775) -> ()  [unwired: 1 in, 2 out]
          n1649 = Fract/Exp String To Number(string=w2792) -> (number=w2790:dbl[][])  [unwired: 3 in, 1 out]
          n1650 = Fract/Exp String To Number(string=w2797) -> (number=w2796:dbl[][])  [unwired: 3 in, 1 out]
          n1651 = case shown="0, Default" w2784 {
            tunnel: w2804 -> [w2843 w2848 w2853 w2858 w2863 w2868 w2873 w2878 w2883]
            tunnel: [w2842 w2847 w2852 w2857 w2862 w2867 w2872 w2877 w2882] -> w2803
            tunnel: w2775 -> [w2841 w2846 w2851 w2856 w2861 w2866 w2871 w2876 w2881]
            tunnel: w2796 -> [w2839 w2844 w2849 w2854 w2859 w2864 w2869 w2874 w2879]
            frame 0, Default {
              n1652 = Bundle By Name(cluster=w2843, "Zone 1.Zone Thermocouples"=w2841) -> (w2842:T17)
              n1653 = control-ref of="Temperature Goal"() -> (w2840:refnum<vi>)
              n1654 = property class="Arr (strict)"(reference=w2840, "Value"=w2839) -> ()  [unwired: 1 in, 2 out]
            }
            frame 1 {
              n1655 = Bundle By Name(cluster=w2848, "Zone 2.Zone Thermocouples"=w2846) -> (w2847:T17)
              n1656 = control-ref of="Temperature Goal"() -> (w2845:refnum<vi>)
              n1657 = property class="Arr (strict)"(reference=w2845, "Value"=w2844) -> ()  [unwired: 1 in, 2 out]
            }
            frame 2 {
              n1658 = Bundle By Name(cluster=w2853, "Zone 3.Zone Thermocouples"=w2851) -> (w2852:T17)
              n1659 = control-ref of="Temperature Goal"() -> (w2850:refnum<vi>)
              n1660 = property class="Arr (strict)"(reference=w2850, "Value"=w2849) -> ()  [unwired: 1 in, 2 out]
            }
            frame 3 {
              n1661 = Bundle By Name(cluster=w2858, "Zone 4.Zone Thermocouples"=w2856) -> (w2857:T17)
              n1662 = control-ref of="Temperature Goal"() -> (w2855:refnum<vi>)
              n1663 = property class="Arr (strict)"(reference=w2855, "Value"=w2854) -> ()  [unwired: 1 in, 2 out]
            }
            frame 4 {
              n1664 = Bundle By Name(cluster=w2863, "Zone 5.Zone Thermocouples"=w2861) -> (w2862:T17)
              n1665 = control-ref of="Temperature Goal"() -> (w2860:refnum<vi>)
              n1666 = property class="Arr (strict)"(reference=w2860, "Value"=w2859) -> ()  [unwired: 1 in, 2 out]
            }
            frame 5 {
              n1667 = Bundle By Name(cluster=w2868, "Zone 6.Zone Thermocouples"=w2866) -> (w2867:T17)
              n1668 = control-ref of="Temperature Goal"() -> (w2865:refnum<vi>)
              n1669 = property class="Arr (strict)"(reference=w2865, "Value"=w2864) -> ()  [unwired: 1 in, 2 out]
            }
            frame 6 {
              n1670 = Bundle By Name(cluster=w2873, "Zone 7.Zone Thermocouples"=w2871) -> (w2872:T17)
              n1671 = control-ref of="Temperature Goal"() -> (w2870:refnum<vi>)
              n1672 = property class="Arr (strict)"(reference=w2870, "Value"=w2869) -> ()  [unwired: 1 in, 2 out]
            }
            frame 7 {
              n1673 = Bundle By Name(cluster=w2878, "Zone 8.Zone Thermocouples"=w2876) -> (w2877:T17)
              n1674 = control-ref of="Temperature Goal"() -> (w2875:refnum<vi>)
              n1675 = property class="Arr (strict)"(reference=w2875, "Value"=w2874) -> ()  [unwired: 1 in, 2 out]
            }
            frame 8 {
              n1676 = Bundle By Name(cluster=w2883, "Zone 9.Zone Thermocouples"=w2881) -> (w2882:T17)
              n1677 = control-ref of="Temperature Goal"() -> (w2880:refnum<vi>)
              n1678 = property class="Arr (strict)"(reference=w2880, "Value"=w2879) -> ()  [unwired: 1 in, 2 out]
            }
          }
          n1679 = Equal To 0?(x=w2784) -> (x = 0?=w2791:bool)
          n1680 = case shown="True" w2791 {
            tunnel: w2790 -> [_ w2817]
            frame False {
            }
            frame True {
              n1681 = control-ref of="RampSoakTimes"() -> (w2818:refnum<vi>)
              n1682 = property class="Arr (strict)"(reference=w2818, "Value"=w2817) -> ()  [unwired: 1 in, 2 out]
            }
          }
          n1683 = Index Array(array=w2788, index (row) #1=3 ("dimension size"), index (col) #1=w2784, index (row) #2=4 ("dimension size"), index (col) #2=w2784, index (row) #3=5 ("dimension size"), index (col) #3=w2784) -> (element #1=w2783:string, element #2=w2782:string, element #3=w2781:string)
          n1684 = property class="Str"(reference=w2779, "Value"=w2783) -> ()  [unwired: 1 in, 2 out]
          n1685 = property class="Str"(reference=w2789, "Value"=w2782) -> ()  [unwired: 1 in, 2 out]
          n1686 = property class="Str"(reference=w2780, "Value"=w2781) -> ()  [unwired: 1 in, 2 out]
        }
        n1687 = control-ref of="Number of Set points"() -> (w2730:refnum<vi>)
        n1688 = control-ref of="Thermal Profile Name"() -> (w2716:refnum<vi>)
        n1689 = control-ref of="Zone Selection"() -> (w2734:refnum<vi>)
        n1690 = Bundle By Name(cluster=w2736, "ZoneSetup.Zone Selection"=w2733, "ZoneSetup.Number of Set points"=w2729, "ZoneSetup.Thermal Profile Name"=w2715) -> (w2702:T17)
        n1691 = property class="Str"(reference=w2716, "Text.Text"=w2715) -> ()  [unwired: 1 in, 2 out]
        n1692 = property class="DigNum (strict)"(reference=w2730, "Value"=w2729) -> ()  [unwired: 1 in, 2 out]
        n1693 = property class="LstBox (strict)"(reference=w2734, "Item Symbols"=w2733) -> ()  [unwired: 1 in, 2 out]
        n1694 = Unbundle By Name(w2702) -> ("ZoneSetup.Zone Selection"=w2708:i32[], "ZonesSelected"=w2706:bool[])
        n1695 = for {
          N: 9 -> [_]
          tunnel: w2708 -> [w2746] mode=indexing
          shift-right: [w2744] -> w2705
          shift-left: w2706 -> [w2749]
          shift-right: [w2748] -> w2699
          shift-left: w2703 -> [w2748]
          i -> [w2743]
          n1696 = Equal?(x=37, y=w2746) -> (x = y?=w2745:bool)
          n1697 = case shown="False" w2745 {
            tunnel: w2749 -> [w2753 w2757]
            tunnel: w2743 -> [w2752 w2756]
            tunnel: [w2750 w2754] -> w2744
            frame False {
              n1698 = Replace Array Subset(array=w2753, new element=TRUE ("new element/subarray"), index=w2752) -> (w2750:bool[])
            }
            frame True {
              n1699 = Replace Array Subset(array=w2757, new element=FALSE ("new element/subarray"), index=w2756) -> (w2754:bool[])
            }
          }
        }
        n1700 = local read "importexe"() -> (w2697:dbl)
        n1701 = Increment(x=w2697) -> (x+1=w2696:dbl)
        n1702 = local write "importexe"(w2696) -> ()
        n1703 = Bundle By Name(cluster=w2702, "ZonesSelected"=w2705) -> (w2704:T17)
        n1704 = call-poly "Send Message.vi"("error in (no error)"=w2699, "event buffer"="2", "event"="compileProfile") -> ("error out"=w2701:errorcluster)  [unwired: 8 in]
      }
      frame "saveProfile" {
        n1705 = Unbundle By Name(w3231) -> ("ZoneSetup.Number of Set points"=w3227:dbl)
        n1706 = Initialize Array("", w3227, 12 ("dimension size")) -> (w3226:string[][])
        n1707 = Build Array (concatenate)(string[][] [["zone1", "zone2", "zone3", "zone4", "zone5", "zone6", "zone7", "zone8", "zone9", "", "", ""], ["", "", "", "", "", "", "", "", "", "", "", ""], ["", "", "", "", "", "", "", "", "", "", "", ""], ["", "", "", "", "", "", "", "", "", "", "", ""], ["", "", "", "", "", "", "", "", "", "", "", ""], ["", "", "", "", "", "", "", "", "", "", "", ""], ["setpt", "ramptime", "soaktime", "zone1", "zone2", "zone3", "zone4", "zone5", "zone6", "zone7", "zone8", "zone9"]], w3226) -> (w3225:string[][])
        n1708 = for {
          N: 9 -> [_]
          shift-right: [w3257] -> w3217
          shift-left: w3231 -> [w3257]
          tunnel: w3227 -> [w3237]
          shift-right: [w3249] -> w3224
          shift-left: w3225 -> [w3253]
          i -> [w3247]
          n1709 = Unbundle By Name(w3257) -> ("ZoneProfile.profiles"=w3252:T32)
          n1710 = Index Array(array=w3252, index=w3247) -> (element=w3251:T22)
          n1711 = Unbundle By Name(w3251) -> ("zone"=w3240:i32, "average"=w3243:string, "thermocouples"=w3248:i32[], "maxTemp"=w3256:i32, "minTemp"=w3255:i32, "maxSlope"=w3254:dbl, "thermalprofiles"=w3236:T34)
          n1712 = Subtract(x=w3240, y=1) -> (x-y=w3238:i32)
          n1713 = Equal?(x=w3243, y="") -> (x = y?=w3245:bool)
          n1714 = Equal?(x=w3243, y="0") -> (x = y?=w3242:bool)
          n1715 = Or(x=w3245, y=w3242) -> (x .or. y?=w3239:bool)
          n1716 = case shown="False" w3239 {
            tunnel: w3243 -> [w3304 _]
            tunnel: w3256 -> [w3300 _]
            tunnel: w3255 -> [w3295 _]
            tunnel: w3254 -> [w3291 _]
            tunnel: w3253 -> [w3290 w3325]
            tunnel: [w3279 w3325] -> w3250
            tunnel: w3248 -> [w3289 _]
            tunnel: w3238 -> [w3278 _]
            tunnel: w3237 -> [w3282 _]
            tunnel: w3236 -> [w3281 _]
            frame False {
              n1717 = Number To Decimal String(number=w3300) -> (decimal integer string=w3299:string)  [unwired: 1 in]
              n1718 = Number To Decimal String(number=w3295) -> (decimal integer string=w3298:string)  [unwired: 1 in]
              n1719 = Number To Decimal String(number=w3289) -> (decimal integer string=w3287:string[])  [unwired: 1 in]
              n1720 = Array Size(array=w3287) -> (size(s)=w3288:i32)
              n1721 = Replace Array Subset(array=w3290, new element=w3304, index (row)=1 ("disabled index (row)"), index (col)=w3278) -> (w3286:string[][])
              n1722 = Number To Fractional String(number=w3291) -> (F-format string=w3294:string)  [unwired: 3 in]
              n1723 = for {
                N: w3288 -> [_]
                tunnel: w3287 -> [w3321] mode=indexing
                shift-right: [w3317] -> w3284
                shift-left: w3286 -> [w3317]
                tunnel: [w3316] -> w3285
                i -> [w3319]
                n1724 = Equal To 0?(x=w3319) -> (x = 0?=w3320:bool)
                n1725 = case shown="True" w3320 {
                  tunnel: [w3323 w3324] -> w3318
                  frame False {
                    n1726 = local read "string"() -> (w3323:string)
                  }
                  frame True {
                    w3324 = ""
                    n1727 = local write "string"(w3324) -> ()
                  }
                }
                n1728 = call <vilib>:"Space Constant.vi"() -> ("String"=w3322:string)
                n1729 = Concatenate Strings(w3318, w3321, w3322) -> (w3316:string)
                n1730 = local write "string"(w3316) -> ()
              }
              n1731 = Replace Array Subset(array=w3284, new element=w3285, index (row)=2 ("disabled index (row)"), index (col)=w3278) -> (w3283:string[][])
              n1732 = Replace Array Subset(array=w3283, new element=w3299, index (row)=3 ("disabled index (row)"), index (col)=w3278) -> (w3296:string[][])
              n1733 = Replace Array Subset(array=w3296, new element=w3298, index (row)=4 ("disabled index (row)"), index (col)=w3278) -> (w3292:string[][])
              n1734 = Replace Array Subset(array=w3292, new element=w3294, index (row)=5 ("disabled index (row)"), index (col)=w3278) -> (w3280:string[][])
              n1735 = for {
                N: w3282 -> [_]
                tunnel: w3281 -> [w3315] mode=indexing
                shift-right: [w3312] -> w3279
                shift-left: w3280 -> [w3313]
                tunnel: w3278 -> [w3308]
                i -> [w3311]
                n1736 = Unbundle By Name(w3315) -> ("tempgoal"=w3314:i32)
                n1737 = Add(x=3 ("disabled index (row)"), y=w3308) -> (x+y=w3306:i32)
                n1738 = Add(x=7 ("disabled index (row)"), y=w3311) -> (x+y=w3309:i32)
                n1739 = Number To Decimal String(number=w3314) -> (decimal integer string=w3305:string)  [unwired: 1 in]
                n1740 = Replace Array Subset(array=w3313, new element=w3305, index (row)=w3309, index (col)=w3306) -> (w3312:string[][])
              }
            }
            frame True {
            }
          }
          n1741 = for {
            N: w3237 -> [_]
            tunnel: w3236 -> [w3263] mode=indexing
            shift-right: [w3266] -> w3249
            shift-left: w3250 -> [w3276]
            tunnel: w3247 -> [_]
            tunnel: w3238 -> [_]
            i -> [w3264]
            w3258 = 60.0
            (unwired) 3 ("disabled index (row)")
            n1742 = Unbundle By Name(w3263) -> ("thermalsetpoint"=w3277:i32, "ramp"=w3261:i32, "soakduration"=w3262:i32)
            n1743 = Add(x=7 ("disabled index (row)"), y=w3264) -> (x+y=w3265:i32)
            n1744 = Number To Decimal String(number=w3277) -> (decimal integer string=w3274:string)  [unwired: 1 in]
            n1745 = Divide(x=w3261, y=w3258) -> (x/y=w3260:dbl)
            n1746 = Divide(x=w3262, y=w3258) -> (x/y=w3259:dbl)
            n1747 = Replace Array Subset(array=w3276, new element=w3274, index (row)=w3265, index (col)=0 ("disabled index (row)")) -> (w3273:string[][])
            n1748 = Number To Decimal String(number=w3260) -> (decimal integer string=w3271:string)  [unwired: 1 in]
            n1749 = Replace Array Subset(array=w3273, new element=w3271, index (row)=w3265, index (col)=1 ("disabled index (row)")) -> (w3267:string[][])
            n1750 = Number To Decimal String(number=w3259) -> (decimal integer string=w3269:string)  [unwired: 1 in]
            n1751 = Replace Array Subset(array=w3267, new element=w3269, index (row)=w3265, index (col)=2 ("disabled index (row)")) -> (w3266:string[][])
          }
        }
        n1752 = local read "TVAC Labview"() -> (w3222:bool)
        n1753 = case shown="True" w3222 {
          tunnel: ["C:\\Users\\stefan\\Documents\\GitHub\\TVAC\\head\\Labview2017\\TVAC_GUI\\DatabaseCSV\\" "C:\\Users\\TVAC-admin\\Documents\\TVAC_Github\\head\\Labview2017\\TVAC_GUI\\DatabaseCSV\\" ("file path (use dialog)")] -> w3221
          frame False {
          }
          frame True {
          }
        }
        n1754 = Unbundle By Name(w3217) -> ("ZoneSetup.Thermal Profile Name"=w3216:string)
        n1755 = Concatenate Strings(w3221, w3216, ".csv" ("string")) -> (w3220:string)
        n1756 = String To Path(string=w3220) -> (path=w3218:path)
        n1757 = call-poly <vilib>:"Write Delimited Spreadsheet.vi"("file path (dialog if empty)"=w3218, "2D data"=w3224, "delimiter (\\t)"="," ("delimiter (\\t)")) -> ()  [unwired: 11 in, 2 out]
      }
      frame "graphTC" {
        n1758 = property on="Waveform Chart" class="WFChart (strict)"("LegScrollVis"=TRUE ("Legend:Scrollbar Visible")) -> ()  [unwired: 2 in, 2 out]
        n1759 = Unbundle By Name(w3337) -> ("working array"=w3334:bool[], "Thermocouples"=w3335:T3, "TCs"=w3328:T14)
        n1760 = for {
          N: 120 -> [_]
          tunnel: w3328 -> [w3370] mode=indexing
          tunnel: [w3369] -> w3329 mode=indexing
          shift-right: [w3348] -> w3331
          shift-left: w3335 -> [w3355]
          shift-right: [w3347] -> w3336
          shift-left: w3334 -> [w3346]
          i -> [w3345]
          n1761 = Unbundle By Name(w3370) -> ("thermocouple"=w3379:i32, "temp"=w3343:dbl, "alarm"=w3374:i32, "working"=w3373:bool)
          n1762 = Quotient & Remainder(x=w3345, y=4) -> (x-y*floor(x/y)=w3353:i32, floor(x/y)=w3354:i32)
          n1763 = Index Array(array=w3355, index (row)=w3354, index (col)=w3353) -> (element=w3368:T18)
          n1764 = Multiply(x=w3354, y=4) -> (x*y=w3363:i32)
          n1765 = Multiply(x=w3354, y=4) -> (x*y=w3375:i32)
          n1766 = Unbundle By Name(w3368) -> ("Graph On/Off"=w3352:u32)
          n1767 = Add(x=w3363, y=w3353) -> (x+y=w3361:i32)
          n1768 = Add(x=w3375, y=w3353) -> (x+y=w3344:i32)
          n1769 = Replace Array Subset(array=w3346, new element=w3373, index=w3345) -> (w3347:bool[])
          n1770 = To Double Precision Float(number=w3343) -> (double precision float=w3342:dbl)
          n1771 = Get Date/Time In Seconds() -> (seconds since 1Jan1904=w3372:timestamp)
          n1772 = property on="Waveform Chart" class="WFChart (strict)"("Active Plot"=w3344) -> ()  [unwired: 2 in, 2 out]
          n1773 = Index Array(array=w3347, index=w3361) -> (element=w3360:bool)
          n1774 = Bundle By Name("t0"=w3372) -> (w3371:waveform(dbl))  [unwired: 1 in]
          n1775 = Build Array(w3342) -> (w3341:dbl[])
          n1776 = Number To Fractional String(number=w3342, precision (6)=i16 2 ("width (-)")) -> (F-format string=w3358:string)  [unwired: 2 in]
          n1777 = Bundle By Name(cluster=w3371, "Y"=w3341) -> (w3369:waveform(dbl))
          n1778 = case shown="True" w3360 {
            tunnel: w3352 -> [_ w3384]
            tunnel: [u32 12369084 ("y") w3384] -> w3356
            tunnel: w3358 -> [_ w3383]
            tunnel: ["NaN" w3383] -> w3357
            frame False {
            }
            frame True {
            }
          }
          n1779 = case shown="2" w3374 {
            tunnel: ["" "L" "H"] -> w3349
            tunnel: w3374 -> [_ _ _]
            tunnel: [u32 12369084 u32 2812927 u32 16711680] -> w3350
            frame 0, Default {
            }
            frame 1 {
            }
            frame 2 {
            }
          }
          n1780 = Number To Decimal String(number=w3379) -> (decimal integer string=w3380:string)  [unwired: 1 in]
          n1781 = Index Array(array=w3355, index (row)=w3354, index (col)=w3353) -> (element=w3366:T18)
          n1782 = Equal?(x=w3356, y=u32 6618880) -> (x = y?=w3364:bool)
          n1783 = Concatenate Strings("TC " ("string"), w3380) -> (w3351:string)
          n1784 = property on="Waveform Chart" class="WFChart (strict)"("Plot.Plot Name"=w3351) -> ()  [unwired: 2 in, 2 out]
          n1785 = case shown="True" w3364 {
            tunnel: [w3392 w3400] -> w3367
            tunnel: w3366 -> [w3391 w3399]
            tunnel: w3356 -> [w3389 w3398]
            tunnel: w3357 -> [w3390 w3397]
            tunnel: w3351 -> [w3388 w3396]
            tunnel: w3350 -> [w3387 w3395]
            tunnel: w3349 -> [w3386 w3394]
            frame False {
              n1786 = Bundle By Name(cluster=w3391, "Graph On/Off"=w3389, "TC Label"=w3388, "PlotColor"=u32 12369084 ("y"), "Temperature"=w3390, "Alarm Color"=w3387, "Alarm Status"=w3386) -> (w3392:T18)
            }
            frame True {
              n1787 = property on="Waveform Chart" class="WFChart (strict)"() -> ("Plot.Plot Color"=w3393:u32)  [unwired: 2 in, 2 out]
              n1788 = Bundle By Name(cluster=w3399, "Graph On/Off"=w3398, "TC Label"=w3396, "PlotColor"=w3393, "Temperature"=w3397, "Alarm Color"=w3395, "Alarm Status"=w3394) -> (w3400:T18)
            }
          }
          n1789 = Replace Array Subset(array=w3355, new element=w3367, index (row)=w3354, index (col)=w3353) -> (w3348:T3)
        }
        n1790 = local write "Thermocouples"(w3331) -> ()
        n1791 = Bundle By Name(cluster=w3337, "Thermocouples"=w3331, "working array"=w3336) -> (w3332:T17)
        n1792 = Build Array (concatenate)(waveform(dbl) {"t0"=timestamp(0 s since 1904-01-01), "dt"=1.0, "Y"=[]} ("element"), w3329) -> (w3339:waveform(dbl)[])
        n1793 = Delete From Array(array=w3339, index=0) -> (array with subset deleted=→"Waveform Chart":waveform(dbl)[])  [unwired: 1 in, 1 out]
      }
      frame "receiveCompressorTemp" {
        n1794 = Unflatten From JSON(JSON string=w3411, type and defaults=cluster{"CompressorTemp":dbl} {"CompressorTemp"=0.0}, default null elements? (F)=TRUE) -> (value=w3409:cluster{"CompressorTemp":dbl})  [unwired: 4 in, 1 out]
        n1795 = Unbundle(w3409) -> ("CompressorTemp"=w3408:dbl)
        n1796 = Bundle By Name(cluster=w3413, "Compressor.CompressorTemp"=w3408) -> (w3414:T17)
      }
      frame "receiveDatabase" {
        n1797 = Spreadsheet String To Array(format string="%s", spreadsheet string=w3418, array type (2D Dbl)=string[] []) -> (array=w3416:string[])  [unwired: 1 in]
        n1798 = control-ref of="Saved Database Profiles"() -> (w3419:refnum<vi>)
        n1799 = property class="Ring (strict)"(reference=w3419, "Strings []"=w3416) -> ()  [unwired: 1 in, 2 out]
      }
      frame "receiveCryoPump_plots" {
        w3423 = T36 {"Duty Cycle (0-100)"=0.0, "1st stage Temp (K)"=0.0, "2st stage Temp (K)"=0.0, "Helium Return Pressure (psig)"=0, "Helium Discharge Temp (C)"=0, "Water Inlet Temp (C)"=0, "Water Outlet Temp (C)"=0}
        n1800 = Flatten To JSON(anything=w3423) -> (JSON string=w3422:string)  [unwired: 2 in, 1 out]
        n1801 = Empty String/Path?(string/path=w3422) -> ()  [unwired: 1 out]
        n1802 = Unflatten From JSON(JSON string=w3426, type and defaults=w3423, default null elements? (F)=TRUE) -> (value=w3432:T36)  [unwired: 4 in, 1 out]
        n1803 = Unbundle By Name(w3432) -> ("1st stage Temp (K)"=w3431:dbl, "2st stage Temp (K)"=w3430:dbl)  [unwired: 5 out]
        n1804 = Build Array(w3431) -> (w3428:dbl[])
        n1805 = Build Array(w3430) -> (w3429:dbl[])
        n1806 = Bundle(w3428, w3429) -> (w3425:cluster{dbl[], dbl[]})  [unwired: 1 in]
        n1807 = Bundle By Name(cluster=w3433, "PumpTemps"=w3425) -> (w3434:T17)
      }
      frame "receiveLastError" {
        w3452 = T37 0 items=["no dialog", "OK message", "continue or stop message", "OK message + warnings", "continue/stop + warnings"] ("type of dialog (OK msg:1)")
        n1808 = Unflatten From JSON(JSON string=w3458, type and defaults=T24 {"time"=[], "event"=[], "item"=[], "itemID"=[], "details"=[], "actions"=[]}, default null elements? (F)=TRUE) -> (value=w3446:T24, error out=w3453:errorcluster)  [unwired: 4 in]
        n1809 = Unbundle By Name(w3446) -> ("time"=w3443:string[])
        n1810 = call <vilib>:"Simple Error Handler.vi"("type of dialog (OK msg:1)"=w3452, "error in (no error)"=w3453) -> ("error?"=w3436:bool, "code out"=w3439:i32)  [unwired: 3 in, 3 out]
        n1811 = Equal?(x=w3439, y=-375008) -> (x = y?=w3437:bool)
        n1812 = Not Exclusive Or(1:w3437, 2:w3436) -> (0:w3435:bool)
        n1813 = Index Array(array=w3443, index=0) -> (element=w3442:string)
        n1814 = Equal?(x=w3442, y="") -> (x = y?=w3444:bool)
        n1815 = And(x=w3435, y=w3444) -> (x .and. y?=w3447:bool)
        n1816 = Unbundle By Name(w3451) -> ("ErrorArray"=w3449:string[][], "MasterErrorArray"=w3450:string[][])
        n1817 = case shown="False" w3447 {
          tunnel: [w3480 w3532] -> w3456
          tunnel: w3446 -> [w3479 _]
          tunnel: w3450 -> [w3478 w3532]
          tunnel: w3449 -> [w3477 w3531]
          tunnel: [w3476 w3531] -> w3448
          frame False {
            n1818 = Unbundle By Name(w3479) -> ("time"=w3468:string[], "event"=w3469:string[], "item"=w3463:string[], "itemID"=w3462:i32[], "details"=w3461:string[], "actions"=w3460:string[][])
            n1819 = Array Size(array=w3468) -> (size(s)=w3467:i32)
            n1820 = control-ref of="Current Errors (click to clear)"() -> (w3459:refnum<vi>)
            n1821 = Initialize Array("", 7 ("dimension size")) -> (w3473:string[])
            n1822 = for {
              N: w3467 -> [_]
              shift-right: [w3516] -> w3480
              shift-left: w3478 -> [w3510]
              tunnel: w3469 -> [w3504]
              tunnel: w3468 -> [w3492]
              shift-right: [w3514] -> w3476
              shift-left: w3477 -> [w3515]
              tunnel: w3463 -> [w3491]
              tunnel: w3462 -> [w3489]
              tunnel: w3461 -> [w3484]
              tunnel: w3460 -> [w3494]
              shift-right: [w3517] -> w3472
              shift-left: w3459 -> [w3511]
              shift-right: [w3481] -> _
              shift-left: w3473 -> [w3507]
              i -> [w3483]
              (unwired) 6 ("index")
              (unwired) 5 ("index")
              (unwired) 4 ("index")
              (unwired) 3 ("index")
              n1823 = Index Array(array=w3510, index (col)=2 ("index (row)")) -> (element=w3512:string[])  [unwired: 1 in]
              n1824 = Index Array(array=w3504, index=w3483) -> (element=w3506:string)
              n1825 = Search 1D Array(1D array=w3512, element=w3506) -> (index of element=w3509:i32)  [unwired: 1 in]
              n1826 = Less Than 0?(x=w3509) -> (x < 0?=w3508:bool)
              n1827 = Replace Array Subset(array=w3507, new element=w3506, index=2) -> (w3503:string[])
              n1828 = Index Array(array=w3492, index=w3483) -> (element=w3493:string)
              n1829 = Bundle(w3483, 2) -> (w3518:cluster{i32, i32})  [unwired: 1 in]
              n1830 = Replace Array Subset(array=w3503, new element=w3493, index=1) -> (w3497:string[])
              n1831 = property on="Property Node" class="MCListbox (strict)"(reference=w3511, "ActiveCell"=w3518) -> (reference out=w3517:refnum<vi>)  [unwired: 1 in, 1 out]
              n1832 = Index Array(array=w3491, index=w3483) -> (element=w3490:string)
              n1833 = Replace Array Subset(array=w3497, new element=w3490, index=3) -> (w3496:string[])
              n1834 = Index Array(array=w3489, index=w3483) -> (element=w3488:i32)
              n1835 = Number To Decimal String(number=w3488) -> (decimal integer string=w3487:string)  [unwired: 1 in]
              n1836 = Replace Array Subset(array=w3496, new element=w3487, index=4) -> (w3495:string[])
              n1837 = Index Array(array=w3494) -> (element=w3498:string[])  [unwired: 2 in]
              n1838 = Replace Array Subset(array=w3495, new element=w3498, index=6) -> (w3482:string[])
              n1839 = Index Array(array=w3484, index=w3483) -> (element=w3485:string)
              n1840 = Replace Array Subset(array=w3482, new element=w3485, index=5) -> (w3481:string[])
              n1841 = case shown="True" w3508 {
                tunnel: [w3527 w3529] -> w3516
                tunnel: w3515 -> [w3524 w3530]
                tunnel: [w3526 w3530] -> w3514
                tunnel: w3510 -> [w3525 w3529]
                tunnel: w3481 -> [w3523 _]
                frame True {
                  n1842 = Build Array (concatenate)(w3523, w3524) -> (w3526:string[][])
                  n1843 = Build Array (concatenate)(w3523, w3525) -> (w3527:string[][])
                  n1844 = One Button Dialog(message="There has been an error", button name ("OK")="Proceed to Error Log") -> (true=w3520:bool)
                  n1845 = case shown="True" w3520 {
                    frame False {
                    }
                    frame True {
                      n1846 = local write "Tab Control"(T25."General Status" ("Tab Control")) -> ()
                    }
                  }
                }
                frame False {
                }
              }
            }
            n1847 = Array Size(array=w3476) -> (size(s)=w3466:i32[])
            n1848 = property class="MCListbox (strict)"(reference=w3472, "ItemNames"=w3476) -> ()  [unwired: 1 in, 2 out]
            n1849 = Index Array(array=w3466, index=0) -> (element=w3464:i32)
            n1850 = Initialize Array(37, w3464) -> (w3470:i32[])
            n1851 = property class="MCListbox (strict)"(reference=w3472, "ItemSyms"=w3470) -> ()  [unwired: 1 in, 2 out]
          }
          frame True {
          }
        }
        n1852 = Bundle By Name(cluster=w3451, "MasterErrorArray"=w3456, "ErrorArray"=w3448) -> (w3457:T17)
      }
      frame "receiveLastEvent" {
        w3547 = T37 0 items=["no dialog", "OK message", "continue or stop message", "OK message + warnings", "continue/stop + warnings"] ("type of dialog (OK msg:1)")
        n1853 = Unflatten From JSON(JSON string=w3553, type and defaults=T26 {"time"=[], "category"=[], "message"=[]}, default null elements? (F)=TRUE) -> (value=w3542:T26, error out=w3548:errorcluster)  [unwired: 4 in]
        n1854 = Unbundle By Name(w3542) -> ("time"=w3540:string[])
        n1855 = Index Array(array=w3540, index=0) -> (element=w3539:string)
        n1856 = Equal?(x=w3539, y="") -> (x = y?=w3533:bool)
        n1857 = call <vilib>:"Simple Error Handler.vi"("type of dialog (OK msg:1)"=w3547, "error in (no error)"=w3548) -> ("error?"=w3536:bool)  [unwired: 3 in, 4 out]
        n1858 = Not(x=w3536) -> (.not. x?=w3535:bool)
        n1859 = And(x=w3535, y=w3533) -> (x .and. y?=w3534:bool)
        n1860 = Unbundle By Name(w3546) -> ("EventArray"=w3544:string[][], "MasterEventArray"=w3545:string[][])
        n1861 = case shown="False" w3534 {
          tunnel: [w3572 w3604] -> w3551
          tunnel: w3542 -> [w3571 _]
          tunnel: w3545 -> [w3570 w3604]
          tunnel: w3544 -> [w3569 w3603]
          tunnel: [w3554 w3603] -> w3543
          frame False {
            n1862 = Unbundle By Name(w3571) -> ("time"=w3561:string[], "message"=w3562:string[], "category"=w3556:string[])
            n1863 = Array Size(array=w3561) -> (size(s)=w3560:i32)
            n1864 = Initialize Array("", 4 ("dimension size")) -> (w3566:string[])
            n1865 = for {
              N: w3560 -> [_]
              tunnel: w3566 -> [w3592]
              tunnel: [w3590] -> w3565
              shift-right: [w3586] -> w3572
              shift-left: w3570 -> [w3580]
              tunnel: w3562 -> [w3587]
              tunnel: w3561 -> [w3579]
              shift-right: [w3584] -> w3554
              shift-left: w3569 -> [w3585]
              tunnel: w3556 -> [w3574]
              i -> [w3578]
              n1866 = Index Array(array=w3580, index (col)=1 ("index (row)")) -> (element=w3582:string[])  [unwired: 1 in]
              n1867 = Index Array(array=w3579, index=w3578) -> (element=w3577:string)
              n1868 = control-ref of="Current Events (click to clear)"() -> (w3595:refnum<vi>)
              n1869 = Replace Array Subset(array=w3592, new element=w3587, index=3) -> (w3589:string[])
              n1870 = Search 1D Array(1D array=w3582, element=w3577) -> (index of element=w3581:i32)  [unwired: 1 in]
              n1871 = Replace Array Subset(array=w3589, new element=w3577, index=1) -> (w3575:string[])
              n1872 = Replace Array Subset(array=w3575, new element=w3574, index=2) -> (w3576:string[])
              n1873 = case shown="-1" w3581 {
                tunnel: [w3596 w3602] -> w3586
                tunnel: w3585 -> [w3597 w3600]
                tunnel: [w3597 w3601] -> w3584
                tunnel: w3576 -> [_ w3599]
                tunnel: w3580 -> [w3596 w3598]
                frame 0, Default {
                }
                frame -1 {
                  n1874 = Build Array (concatenate)(w3599, w3600) -> (w3601:string[][])
                  n1875 = Build Array (concatenate)(w3599, w3598) -> (w3602:string[][])
                }
              }
              n1876 = Bundle(w3578, 2) -> (w3593:cluster{i32, i32})  [unwired: 1 in]
              n1877 = property on="Property Node" class="MCListbox (strict)"(reference=w3595, "ActiveCell"=w3593) -> (reference out=w3590:refnum<vi>)  [unwired: 1 in, 1 out]
            }
            n1878 = control-ref of="Complete Event List"() -> (w3555:refnum<vi>)
            n1879 = Array Size(array=w3554) -> (size(s)=w3559:i32[])
            n1880 = property class="MCListbox (strict)"(reference=w3565, "ItemNames"=w3554) -> ()  [unwired: 1 in, 2 out]
            n1881 = Index Array(array=w3559, index=0) -> (element=w3557:i32)
            n1882 = Initialize Array(37, w3557) -> (w3563:i32[])
            n1883 = property class="MCListbox (strict)"(reference=w3565, "ItemSyms"=w3563) -> ()  [unwired: 1 in, 2 out]
            n1884 = property class="MCListbox (strict)"(reference=w3555, "ItemNames"=w3554) -> ()  [unwired: 1 in, 2 out]
          }
          frame True {
          }
        }
        n1885 = Bundle By Name(cluster=w3546, "MasterEventArray"=w3551, "EventArray"=w3543) -> (w3552:T17)
      }
      frame "receivePressure" {
        n1886 = Unflatten From JSON(JSON string=w3606, type and defaults=T27 {"CryoPressure"=0.0, "ChamberPressure"=0.0, "RoughingPressure"=0.0}, default null elements? (F)=TRUE) -> (value=w3612:T27)  [unwired: 4 in, 1 out]
        n1887 = Unbundle By Name(w3612) -> ("RoughingPressure"=w3611:dbl, "CryoPressure"=w3610:dbl, "ChamberPressure"=w3609:dbl)
        n1888 = Build Array(w3611, w3610, w3609) -> (w3613:dbl[])
        n1889 = Bundle By Name(cluster=w3615, "Pressure"=w3613) -> (w3614:T17)
      }
      frame "receiveTC" {
        n1890 = Unflatten From JSON(JSON string=w3630, type and defaults=T19 {"time"="", "TCs"=[]} ("Cluster"), default null elements? (F)=TRUE) -> (value=w3632:T19)  [unwired: 4 in, 1 out]
        n1891 = control-ref of="TC1to75visual"() -> (w3627:refnum<vi>)
        n1892 = Unbundle By Name(w3632) -> ("TCs"=w3616:T14)
        n1893 = property class="Clust (strict)"(reference=w3627) -> ("Controls[]"=w3624:refnum<vi>[])  [unwired: 1 in, 2 out]
        n1894 = Bundle By Name(cluster=w3631, "TCs"=w3616) -> (w3626:T17)
        n1895 = for {
          N: 75 -> [_]
          tunnel: w3624 -> [w3659] mode=indexing
          tunnel: w3616 -> [w3661] mode=indexing
          n1896 = Unbundle By Name(w3661) -> ("temp"=w3660:dbl)
          n1897 = Number To Decimal String(number=w3660) -> (decimal integer string=w3658:string)  [unwired: 1 in]
          n1898 = property class="Ctl"(reference=w3659, "TipStrip"=w3658) -> ()  [unwired: 1 in, 2 out]
        }
        n1899 = Initialize Array(0.0 ("element"), 30 ("dimension size")) -> (w3619:dbl[])
        n1900 = for {
          N: 30 -> [_]
          shift-right: [w3635] -> w3618
          shift-left: w3619 -> [w3636]
          tunnel: w3616 -> [w3634]
          i -> [w3633]
          n1901 = In Range and Coerce(upper limit=5 ("lower limit"), x=w3633, lower limit=0) -> (In Range?=w3639:bool)  [unwired: 1 out]
          n1902 = case shown="True" w3639 {
            tunnel: w3636 -> [w3648 w3657]
            tunnel: w3633 -> [w3646 w3655]
            tunnel: [w3647 w3656] -> w3635
            tunnel: w3634 -> [w3645 w3651]
            tunnel: w3633 -> [w3644 w3650]
            frame False {
              n1903 = Add(x=90, y=w3644) -> (x+y=w3642:i32)
              n1904 = Index Array(array=w3645, index=w3642) -> (element=w3641:T38)
              n1905 = Unbundle By Name(w3641) -> ("temp"=w3640:dbl)
              n1906 = Replace Array Subset(array=w3648, new element=w3640, index=w3646) -> (w3647:dbl[])
            }
            frame True {
              n1907 = Add(x=75, y=w3650) -> (x+y=w3653:i32)
              n1908 = Index Array(array=w3651, index=w3653) -> (element=w3652:T38)
              n1909 = Unbundle By Name(w3652) -> ("temp"=w3649:dbl)
              n1910 = Replace Array Subset(array=w3657, new element=w3649, index=w3655) -> (w3656:dbl[])
            }
          }
        }
        n1911 = Array To Cluster(array=w3618) -> (cluster=w3617:T39)
        n1912 = local write "Chamber Layout"(w3617) -> ()
      }
      frame "receiveTvacStatus" {
        n1913 = Unflatten From JSON(JSON string=w3704, type and defaults=T12 {"recordData"=FALSE, "currentSetpoint"=0, "vacuumWanted"=FALSE, "inPause"=FALSE, "activeProfile"=FALSE, "inRamp"=FALSE, "inHold"=FALSE, "CryoPressure"=0.0, "ChamberPressure"=0.0, "RoughingPressure"=0.0, "OperationalVacuum"=FALSE} ("OperationalVacuum"), default null elements? (F)=TRUE) -> (value=w3700:T12)  [unwired: 4 in, 1 out]
        n1914 = Bundle By Name(cluster=w3699, "TvacStatus"=w3700) -> (w3674:T17)
        n1915 = Initialize Array(0.0 ("element"), 9 ("dimension size")) -> (w3680:dbl[])
        n1916 = Unbundle By Name(w3674) -> ("TvacStatus"=w3675:T12, "ZoneTemps.ZoneTemps"=w3679:dbl[])
        n1917 = Array Size(array=w3679) -> (size(s)=w3682:i32)
        n1918 = for {
          N: w3682 -> [_]
          shift-right: [w3713] -> _
          shift-left: w3679 -> [w3714]
          shift-right: [w3705] -> w3678
          shift-left: w3680 -> [w3708]
          shift-right: [w3706] -> _
          shift-left: 0 ("dimension size") -> [w3707]
          i -> [w3712]
          n1919 = Quotient & Remainder(x=w3712, y=2) -> (x-y*floor(x/y)=w3710:i32)  [unwired: 1 out]
          n1920 = Equal To 0?(x=w3710) -> (x = 0?=w3709:bool)
          n1921 = case shown="True" w3709 {
            tunnel: w3714 -> [w3715 w3718]
            tunnel: [w3715 w3718] -> w3713
            tunnel: w3712 -> [_ w3724]
            tunnel: w3708 -> [w3716 w3721]
            tunnel: w3707 -> [w3717 w3723]
            tunnel: [w3717 w3722] -> w3706
            tunnel: [w3716 w3719] -> w3705
            frame False {
            }
            frame True {
              n1922 = Index Array(array=w3718, index=w3724) -> (element=w3720:dbl)
              n1923 = Replace Array Subset(array=w3721, new element=w3720, index=w3723) -> (w3719:dbl[])
              n1924 = Increment(x=w3723) -> (x+1=w3722:i32)
            }
          }
        }
        n1925 = Unbundle By Name(w3675) -> ("recordData"=w3685:bool, "currentSetpoint"=w3698:i32, "vacuumWanted"=w3697:bool, "inPause"=w3689:bool, "activeProfile"=w3696:bool, "inRamp"=w3688:bool, "inHold"=w3687:bool, "CryoPressure"=w3694:dbl, "ChamberPressure"=w3693:dbl, "RoughingPressure"=w3695:dbl, "OperationalVacuum"=w3663:bool)
        n1926 = case shown="False" w3689 {
          tunnel: w3688 -> [w3727 _]
          tunnel: w3687 -> [w3726 _]
          tunnel: [w3725 "Paused"] -> w3686
          frame False {
            n1927 = case shown="False" w3727 {
              tunnel: w3726 -> [w3729 _]
              tunnel: [w3728 "Ramping"] -> w3725
              frame False {
                n1928 = case shown="True" w3729 {
                  tunnel: ["" "Holding"] -> w3728
                  frame False {
                  }
                  frame True {
                  }
                }
              }
              frame True {
              }
            }
          }
          frame True {
          }
        }
        n1929 = local write "Database Logging On/Off"(w3685) -> ()
        n1930 = Bundle By Name(cluster=T28 {"Set Point"=0.0, "Vacuum Wanted"=FALSE, "Profile State"="", "Active Profile"=FALSE, "Roughing"=0.0, "Cryo"=0.0, "Chamber"=0.0, "Current Ramp/Soak Time"=0.0, "Zone Temps"=[], "Remaining Ramp/Soak Time"=0.0, "Max Ramp Rate"=0.0, "Vacuum State"="", "At Vacuum"=FALSE} ("tpStatus"), "Set Point"=w3698, "Vacuum Wanted"=w3697, "Profile State"=w3686, "Active Profile"=w3696, "Roughing"=w3695, "Cryo"=w3694, "Chamber"=w3693, "Current Ramp/Soak Time"=0.0, "Zone Temps"=w3678, "Remaining Ramp/Soak Time"=0.0, "Max Ramp Rate"=0.0, "Vacuum State"="", "At Vacuum"=w3663) -> (w3676:T28)
        n1931 = local write "tpStatus"(w3676) -> ()
        n1932 = local write "generalStatus"(w3676) -> ()
        n1933 = Unbundle By Name(w3675) -> ("currentSetpoint"=w3666:i32, "vacuumWanted"=w3671:bool, "activeProfile"=w3670:bool, "CryoPressure"=w3669:dbl, "ChamberPressure"=w3668:dbl, "RoughingPressure"=w3667:dbl)
        n1934 = Bundle By Name(cluster=T1 {"At Vaccum"=FALSE, "Vacuum Wanted"=FALSE, "Roughing"=0.0, "Cryo"=0.0, "Chamber"=0.0, "Active Profile"=FALSE, "Set Point"=0.0, "Max Temp"="", "Min Temp"="", "Uncleared Errors"=FALSE} ("Taskbar Status"), "At Vaccum"=w3663, "Vacuum Wanted"=w3671, "Roughing"=w3667, "Cryo"=w3669, "Chamber"=w3668, "Active Profile"=w3670, "Set Point"=w3666, "Max Temp"="Infinity", "Min Temp"="& Beyond") -> (w3672:T1)
        n1935 = local write "Taskbar Status"(w3672) -> ()
      }
      frame "receiveZoneTemps" {
        n1936 = Unflatten From JSON(JSON string=w3737, type and defaults=cluster{"ZoneTemps":dbl[]} {"ZoneTemps"=[]}, default null elements? (F)=TRUE) -> (value=w3735:cluster{"ZoneTemps":dbl[]})  [unwired: 4 in, 1 out]
        n1937 = Bundle By Name(cluster=w3739, "ZoneTemps"=w3735) -> (w3740:T17)
      }
      frame "masterDatabase" {
        n1938 = Unbundle By Name(w3754) -> ("Thermocouples"=w3755:T3, "Pressure"=w3747:dbl[], "PumpTemps"=w3750:T15, "NumberTCs"=w3756:i32, "ZoneTemps"=w3744:cluster{"ZoneTemps":dbl[]}, "Compressor.CompressorTemp"=w3742:dbl)  [unwired: 1 out]
        n1939 = Initialize Array(0.0 ("element"), w3756) -> (w3758:dbl[])
        n1940 = Unbundle(w3750) -> ("Cp Stage 1 Temp"=w3749:dbl[], "Cp Stage 2 Temp"=w3748:dbl[])
        n1941 = Unbundle(w3744) -> ("ZoneTemps"=w3743:dbl[])
        n1942 = Build Array (concatenate)(w3749, w3748) -> (w3746:dbl[])
        n1943 = Build Array(w3742) -> (w3741:dbl[])
        n1944 = for {
          N: w3756 -> [_]
          shift-right: [w3768] -> w3745
          shift-left: w3758 -> [w3769]
          tunnel: w3755 -> [w3764]
          i -> [w3766]
          n1945 = Quotient & Remainder(x=w3766, y=4) -> (x-y*floor(x/y)=w3763:i32, floor(x/y)=w3765:i32)
          n1946 = Index Array(array=w3764, index (row)=w3765, index (col)=w3763) -> (element=w3762:T18)
          n1947 = Unbundle By Name(w3762) -> ("Temperature"=w3761:string)
          n1948 = Fract/Exp String To Number(string=w3761) -> (number=w3760:dbl)  [unwired: 3 in, 1 out]
          n1949 = To Double Precision Float(number=w3760) -> (double precision float=w3770:dbl)
          n1950 = Replace Array Subset(array=w3769, new element=w3770, index=w3766) -> (w3768:dbl[])
        }
        n1951 = Build Array (concatenate)(dbl[] [0.0], w3747, w3743, w3745, w3746, w3741) -> (w3752:dbl[])
        n1952 = Bundle By Name(cluster=w3754, "Database"=w3752) -> (w3753:T17)
      }
      frame "multipleGraphs" {
        n1953 = local read "Custom Graph Selector"() -> (w3771:i32)
        n1954 = for {
          N: 6 ("Numeric") -> [_]
          tunnel: w3774 -> [w3788]
          tunnel: w3773 -> [w3787]
          tunnel: w3771 -> [w3778]
          i -> [w3775]
          n1955 = case shown="0, Default" w3775 {
            tunnel: [w3834 w3835 w3837 w3839 w3841 w3843] -> w3780
            tunnel: [w3833 w3836 w3838 w3840 w3842 w3844] -> w3779
            frame 0, Default {
              n1956 = control-ref of="Custom Chart 1 Selection"() -> (w3833:refnum<vi>)
              n1957 = control-ref of="Custom Chart 1"() -> (w3834:refnum<vi>)
            }
            frame 1 {
              n1958 = control-ref of="Custom Chart 2 Selection"() -> (w3836:refnum<vi>)
              n1959 = control-ref of="Custom Chart 2"() -> (w3835:refnum<vi>)
            }
            frame 2 {
              n1960 = control-ref of="Custom Chart 3 Selection"() -> (w3838:refnum<vi>)
              n1961 = control-ref of="Custom Chart 3"() -> (w3837:refnum<vi>)
            }
            frame 3 {
              n1962 = control-ref of="Custom Chart 4 Selection"() -> (w3840:refnum<vi>)
              n1963 = control-ref of="Custom Chart 4"() -> (w3839:refnum<vi>)
            }
            frame 4 {
              n1964 = control-ref of="Custom Chart 5 Selection"() -> (w3842:refnum<vi>)
              n1965 = control-ref of="Custom Chart 5"() -> (w3841:refnum<vi>)
            }
            frame 5 {
              n1966 = control-ref of="Custom Chart 6 Selection"() -> (w3844:refnum<vi>)
              n1967 = control-ref of="Custom Chart 6"() -> (w3843:refnum<vi>)
            }
          }
          n1968 = Equal?(x=w3778, y=w3775) -> (x = y?=w3776:bool)
          n1969 = Unbundle By Name(w3787) -> ("Database"=w3785:dbl[], "numSensors"=w3786:i32)
          n1970 = case shown="True" w3776 {
            tunnel: w3788 -> [_ w3802]
            tunnel: [w3791 w3796] -> w3784
            tunnel: [1000 w3795] -> w3783
            tunnel: w3779 -> [w3792 w3794]
            tunnel: [FALSE w3793] -> w3777
            frame False {
              n1971 = property on="Property Node" class="LstBox (strict)"(reference=w3792) -> ("Item Symbols"=w3791:i32[])  [unwired: 1 in, 2 out]
            }
            frame True {
              n1972 = property on="Property Node" class="LstBox (strict)"(reference=w3794) -> ("Item Symbols"=w3796:i32[])  [unwired: 1 in, 2 out]
              n1973 = Decimal String To Number(string=w3802) -> (number=w3795:i32)  [unwired: 2 in, 1 out]
              n1974 = Index Array(array=w3796, index=0) -> (element=w3797:i32)
              n1975 = Equal?(x=37, y=w3797) -> (x = y?=w3799:bool)
              n1976 = Equal To 0?(x=w3795) -> (x = 0?=w3801:bool)
              n1977 = And(x=w3799, y=w3801) -> (x .and. y?=w3793:bool)
            }
          }
          n1978 = case shown="True" w3777 {
            tunnel: [0 ("index") w3911] -> w3782
            tunnel: w3786 -> [w3851 w3907]
            tunnel: w3785 -> [w3850 _]
            tunnel: [w3849 _] -> w3781
            tunnel: w3783 -> [w3847 w3911]
            tunnel: w3784 -> [w3848 w3910]
            tunnel: w3779 -> [w3846 w3906]
            tunnel: w3780 -> [w3845 w3905]
            frame False {
              n1979 = for {
                N: w3851 -> [_]
                tunnel: [w3880] -> w3849 mode=indexing
                tunnel: w3847 -> [w3874]
                tunnel: w3848 -> [w3869]
                tunnel: w3850 -> [w3859] mode=indexing
                tunnel: w3846 -> [w3867]
                tunnel: w3845 -> [w3866]
                i -> [w3856]
                n1980 = Wait (ms)(milliseconds to wait=u32 0) -> ()  [unwired: 1 out]
                n1981 = In Range and Coerce(upper limit=22, x=w3856, lower limit=3) -> (In Range?=w3854:bool)  [unwired: 1 out]
                n1982 = Equal To 0?(x=w3859) -> (x = 0?=w3861:bool)
                n1983 = Not A Number/Path/Refnum?(number/path/refnum=w3859) -> (NaN/Path/Refnum?=w3860:bool)
                n1984 = In Range and Coerce(upper limit=145 ("lower limit"), x=w3856, lower limit=142) -> (In Range?=w3855:bool)  [unwired: 1 out]
                n1985 = Or(x=w3855, y=w3854) -> (x .or. y?=w3853:bool)
                n1986 = Or(x=w3860, y=w3861) -> (x .or. y?=w3862:bool)
                n1987 = Not And(1:w3853, 2:w3862) -> (0:w3863:bool)
                n1988 = case shown="True" w3863 {
                  tunnel: [waveform(dbl) {"t0"=timestamp(0 s since 1904-01-01), "dt"=1.0, "Y"=[]} w3884] -> w3880
                  tunnel: w3859 -> [_ w3882]
                  frame False {
                  }
                  frame True {
                    n1989 = Get Date/Time In Seconds() -> (seconds since 1Jan1904=w3886:timestamp)
                    n1990 = Bundle By Name("t0"=w3886) -> (w3885:waveform(dbl))  [unwired: 1 in]
                    n1991 = Build Array(w3882) -> (w3883:dbl[])
                    n1992 = Bundle By Name(cluster=w3885, "Y"=w3883) -> (w3884:waveform(dbl))
                  }
                }
                n1993 = Index Array(array=w3869, index=w3874) -> (element=w3872:i32)
                n1994 = Index Array(array=w3869, index=w3874) -> (element=w3875:i32)
                n1995 = Equal?(x=w3872, y=38) -> (x = y?=w3871:bool)
                n1996 = Equal?(x=w3875, y=37) -> (x = y?=w3877:bool)
                n1997 = Equal?(x=w3856, y=w3874) -> (x = y?=w3870:bool)
                n1998 = And(x=w3870, y=w3871) -> (x .and. y?=w3868:bool)
                n1999 = And(x=w3870, y=w3877) -> (x .and. y?=w3876:bool)
                n2000 = case shown="True" w3876 {
                  tunnel: w3869 -> [_ w3904]
                  tunnel: w3874 -> [_ _]
                  tunnel: w3856 -> [_ w3899]
                  tunnel: w3866 -> [_ w3898]
                  tunnel: w3867 -> [_ w3897]
                  frame False {
                  }
                  frame True {
                    n2001 = property on="Property Node" class="WFChart (strict)"(reference=w3898, "Active Plot"=w3899) -> (reference out=w3902:refnum<vi>)  [unwired: 1 in, 1 out]
                    n2002 = Replace Array Subset(array=w3904, new element=38, index=w3899) -> (w3900:i32[])
                    n2003 = property on="Property Node" class="WFChart (strict)"(reference=w3898) -> ("Plot.Plot Color"=w3896:u32)  [unwired: 1 in, 2 out]
                    n2004 = property on="Property Node" class="WFChart (strict)"(reference=w3902, "Plot.Visible?"=TRUE ("Plot.Visible")) -> ()  [unwired: 1 in, 2 out]
                    n2005 = property on="Property Node" class="LstBox (strict)"(reference=w3897, "Active Row"=w3899) -> ()  [unwired: 1 in, 2 out]
                    n2006 = property on="Property Node" class="LstBox (strict)"(reference=w3897, "CellBG"=w3896) -> ()  [unwired: 1 in, 2 out]
                    n2007 = property on="Property Node" class="LstBox (strict)"(reference=w3897, "Item Symbols"=w3900) -> ()  [unwired: 1 in, 2 out]
                  }
                }
                n2008 = case shown="True" w3868 {
                  tunnel: w3869 -> [_ w3895]
                  tunnel: w3856 -> [_ w3888]
                  tunnel: w3866 -> [_ w3889]
                  tunnel: w3867 -> [_ w3890]
                  frame False {
                  }
                  frame True {
                    n2009 = property on="Property Node" class="WFChart (strict)"(reference=w3889, "Active Plot"=w3888) -> (reference out=w3893:refnum<vi>)  [unwired: 1 in, 1 out]
                    n2010 = Replace Array Subset(array=w3895, new element=37, index=w3888) -> (w3891:i32[])
                    n2011 = property on="Property Node" class="WFChart (strict)"(reference=w3893, "Plot.Visible?"=FALSE ("Plot.Visible")) -> ()  [unwired: 1 in, 2 out]
                    n2012 = property on="Property Node" class="LstBox (strict)"(reference=w3890, "Active Row"=w3888) -> ()  [unwired: 1 in, 2 out]
                    n2013 = property on="Property Node" class="LstBox (strict)"(reference=w3890, "CellBG"=u32 13816530 ("Active Row:Cell Background Color")) -> ()  [unwired: 1 in, 2 out]
                    n2014 = property on="Property Node" class="LstBox (strict)"(reference=w3890, "Item Symbols"=w3891) -> ()  [unwired: 1 in, 2 out]
                  }
                }
              }
            }
            frame True {
              n2015 = for {
                N: w3907 -> [_]
                tunnel: w3910 -> [_]
                tunnel: w3906 -> [w3913]
                tunnel: w3905 -> [w3912]
                i -> [w3914]
                n2016 = property on="Property Node" class="WFChart (strict)"(reference=w3912, "Active Plot"=w3914) -> (reference out=w3917:refnum<vi>)  [unwired: 1 in, 1 out]
                n2017 = property on="Property Node" class="WFChart (strict)"(reference=w3917, "Plot.Visible?"=FALSE ("Plot.Visible")) -> ()  [unwired: 1 in, 2 out]
                n2018 = property on="Property Node" class="LstBox (strict)"(reference=w3913, "Active Row"=w3914) -> ()  [unwired: 1 in, 2 out]
                n2019 = property on="Property Node" class="LstBox (strict)"(reference=w3913, "CellBG"=u32 13816530 ("Active Row:Cell Background Color")) -> ()  [unwired: 1 in, 2 out]
              }
              n2020 = Initialize Array(37, w3907) -> (w3908:i32[])
              n2021 = property on="Property Node" class="LstBox (strict)"(reference=w3906, "Item Symbols"=w3908) -> ()  [unwired: 1 in, 2 out]
            }
          }
          n2022 = case shown="0, Default" w3775 {
            tunnel: w3782 -> [w3806 w3809 w3814 w3819 w3824 w3829]
            tunnel: w3781 -> [w3804 w3808 w3813 w3818 w3823 w3828]
            frame 0, Default {
              n2023 = Build Array (concatenate)(waveform(dbl) {"t0"=timestamp(0 s since 1904-01-01), "dt"=1.0, "Y"=[]} ("element"), w3804) -> (w3803:waveform(dbl)[])
              n2024 = Delete From Array(array=w3803, index=w3806) -> (array with subset deleted=→"Custom Chart 1":waveform(dbl)[])  [unwired: 1 in, 1 out]
            }
            frame 1 {
              n2025 = Build Array (concatenate)(waveform(dbl) {"t0"=timestamp(0 s since 1904-01-01), "dt"=1.0, "Y"=[]} ("element"), w3808) -> (w3812:waveform(dbl)[])
              n2026 = Delete From Array(array=w3812, index=w3809) -> (array with subset deleted=→"Custom Chart 2":waveform(dbl)[])  [unwired: 1 in, 1 out]
            }
            frame 2 {
              n2027 = Build Array (concatenate)(waveform(dbl) {"t0"=timestamp(0 s since 1904-01-01), "dt"=1.0, "Y"=[]} ("element"), w3813) -> (w3817:waveform(dbl)[])
              n2028 = Delete From Array(array=w3817, index=w3814) -> (array with subset deleted=→"Custom Chart 3":waveform(dbl)[])  [unwired: 1 in, 1 out]
            }
            frame 3 {
              n2029 = Build Array (concatenate)(waveform(dbl) {"t0"=timestamp(0 s since 1904-01-01), "dt"=1.0, "Y"=[]} ("element"), w3818) -> (w3822:waveform(dbl)[])
              n2030 = Delete From Array(array=w3822, index=w3819) -> (array with subset deleted=→"Custom Chart 4":waveform(dbl)[])  [unwired: 1 in, 1 out]
            }
            frame 4 {
              n2031 = Build Array (concatenate)(waveform(dbl) {"t0"=timestamp(0 s since 1904-01-01), "dt"=1.0, "Y"=[]} ("element"), w3823) -> (w3827:waveform(dbl)[])
              n2032 = Delete From Array(array=w3827, index=w3824) -> (array with subset deleted=→"Custom Chart 5":waveform(dbl)[])  [unwired: 1 in, 1 out]
            }
            frame 5 {
              n2033 = Build Array (concatenate)(waveform(dbl) {"t0"=timestamp(0 s since 1904-01-01), "dt"=1.0, "Y"=[]} ("element"), w3828) -> (w3832:waveform(dbl)[])
              n2034 = Delete From Array(array=w3832, index=w3829) -> (array with subset deleted=→"Custom Chart 6":waveform(dbl)[])  [unwired: 1 in, 1 out]
            }
          }
        }
      }
      frame "exit" {
        n2035 = Unbundle By Name(w3919) -> ("Http session"=w3920:T16)
        n2036 = call <vilib>:"CloseHandle.vi"("client handle"=w3920, "error in (no error)"=w3922) -> ("error out"=w3921:errorcluster)  [unwired: 13 in]
        n2037 = Bundle By Name(cluster=w3919, "go"=FALSE ("Bundle Element")) -> (w3923:T17)
      }
      frame Default {
        n2038 = call "Unknown Message Dialog.vi"("error in (no error)"=w3926, "event name"=w3925) -> ("error out"=w3924:errorcluster)  [unwired: 9 in]
      }
    }
    n2039 = Unbundle By Name(w64) -> ("go"=w63:bool)
    n2040 = call "log system event.vi"("error in (no error)"=w60) -> ("error out"=w65:errorcluster, "description"=→"system log event":string)  [unwired: 9 in]
    n2041 = call <vilib>:"Simple Error Handler.vi"("error in (no error)"=w60) -> ()  [unwired: 4 in, 5 out]
  }
  n2042 = local read "TVAC Labview"() -> (w1:bool)
  n2043 = local read "Local Debug"() -> (w29:bool)
  n2044 = call "getData.vi"("TVAC Labview"=w1, "Local Debug"=w29) -> ()  [unwired: 10 in]
  n2045 = while {
    shift-right: [w3929] -> _
    shift-left: "Moving 1" -> [w3930]
    tunnel: T11[] [{"Left"=436, "Top"=451}, {"Left"=477, "Top"=451}, {"Left"=519, "Top"=451}, {"Left"=561, "Top"=451}, {"Left"=602, "Top"=451}, {"Left"=644, "Top"=451}, {"Left"=686, "Top"=451}, {"Left"=727, "Top"=451}, {"Left"=769, "Top"=451}, {"Left"=811, "Top"=451}, {"Left"=851, "Top"=449}, {"Left"=894, "Top"=451}, {"Left"=935, "Top"=451}, {"Left"=977, "Top"=451}, {"Left"=1019, "Top"=451}, {"Left"=1062, "Top"=451}, {"Left"=1103, "Top"=451}, {"Left"=1145, "Top"=451}, {"Left"=1187, "Top"=451}, {"Left"=1228, "Top"=451}, {"Left"=437, "Top"=486}, {"Left"=479, "Top"=486}, {"Left"=520, "Top"=486}, {"Left"=562, "Top"=486}, {"Left"=604, "Top"=486}, {"Left"=645, "Top"=486}, {"Left"=687, "Top"=486}, {"Left"=729, "Top"=486}, {"Left"=770, "Top"=486}, {"Left"=812, "Top"=486}, {"Left"=851, "Top"=484}, {"Left"=894, "Top"=486}, {"Left"=936, "Top"=486}, {"Left"=978, "Top"=486}, {"Left"=1019, "Top"=486}, {"Left"=1061, "Top"=486}, {"Left"=1103, "Top"=486}, {"Left"=1144, "Top"=486}, {"Left"=1186, "Top"=486}, {"Left"=1228, "Top"=486}, {"Left"=438, "Top"=520}, {"Left"=480, "Top"=520}, {"Left"=522, "Top"=520}, {"Left"=563, "Top"=520}, {"Left"=605, "Top"=520}, {"Left"=646, "Top"=521}, {"Left"=687, "Top"=520}, {"Left"=729, "Top"=520}, {"Left"=771, "Top"=520}, {"Left"=812, "Top"=520}, {"Left"=854, "Top"=520}, {"Left"=895, "Top"=520}, {"Left"=936, "Top"=520}, {"Left"=978, "Top"=520}, {"Left"=1020, "Top"=520}, {"Left"=1061, "Top"=520}, {"Left"=1101, "Top"=520}, {"Left"=1145, "Top"=520}, {"Left"=1186, "Top"=520}, {"Left"=1228, "Top"=520}, {"Left"=439, "Top"=554}, {"Left"=480, "Top"=554}, {"Left"=522, "Top"=554}, {"Left"=564, "Top"=554}, {"Left"=605, "Top"=554}, {"Left"=647, "Top"=554}, {"Left"=688, "Top"=554}, {"Left"=730, "Top"=554}, {"Left"=772, "Top"=554}, {"Left"=813, "Top"=554}, {"Left"=854, "Top"=554}, {"Left"=896, "Top"=554}, {"Left"=936, "Top"=554}, {"Left"=978, "Top"=554}, {"Left"=1020, "Top"=554}] ("TCs1to75InitialPositions") -> [w3928]
    stop <- w3932 stop-if-true
    n2046 = event shown="[0] Timeout" {
      selector: _ -> [_ _ _ _ _]
      dyn-events: _ -> [_ _ _ _ _]
      timeout: 750 -> [_ _ _ _ _]
      tunnel: w3930 -> [_ w3933 _ _ _]
      tunnel: [_ w3933 FALSE TRUE _] -> w3929
      tunnel: w3928 -> [_ _ _ _ w3986]
      event Timeout {
        n2047 = event-data() -> ()  [unwired: 1 in, 3 out]
      }
      event "TC1to75visual": Mouse Move {
        n2048 = event-data() -> ("Coords"=w3934:T30)  [unwired: 1 in]
        n2049 = local read "Moving 1"() -> (w3935:bool)
        n2050 = case shown="False" w3935 {
          tunnel: w3933 -> [w3936 w3974]
          tunnel: w3934 -> [w3937 w3972]
          frame False {
            n2051 = control-ref of="TC1to75visual"() -> (w3940:refnum<vi>)
            n2052 = property class="Clust (strict)"(reference=w3940) -> ("Controls[]"=w3938:refnum<vi>[])  [unwired: 1 in, 2 out]
            n2053 = for {
              N: 75 -> [_]
              shift-right: [w3942] -> _
              shift-left: w3937 -> [w3945]
              tunnel: w3938 -> [w3957] mode=indexing
              tunnel: w3936 -> [w3943]
              n2054 = property class="Ctl"(reference=w3957) -> (reference out=w3944:refnum<vi>, "Position"=w3946:T11)  [unwired: 1 in, 1 out]
              n2055 = Unbundle By Name(w3945) -> ("Horizontal"=w3953:i32, "Vertical"=w3952:i32)
              n2056 = Unbundle By Name(w3946) -> ("Left"=w3947:i32, "Top"=w3950:i32)
              n2057 = Add(x=w3950, y=24) -> (x+y=w3951:i32)
              n2058 = Add(x=w3947, y=32) -> (x+y=w3956:i32)
              n2059 = In Range and Coerce(upper limit=w3956, x=w3953, lower limit=w3947) -> (In Range?=w3949:bool)  [unwired: 1 out]
              n2060 = In Range and Coerce(upper limit=w3951, x=w3952, lower limit=w3950) -> (In Range?=w3948:bool)  [unwired: 1 out]
              n2061 = And(x=w3949, y=w3948) -> (x .and. y?=w3941:bool)
              n2062 = case shown="False" w3941 {
                tunnel: w3945 -> [w3958 w3960]
                tunnel: w3944 -> [_ w3962]
                tunnel: w3943 -> [_ w3961]
                tunnel: [w3958 w3959] -> w3942
                frame False {
                }
                frame True {
                  n2063 = local write "TC1to45PicRef"(w3962) -> ()
                  n2064 = case shown="False" w3961 {
                    selector: w3961 -> [_ w3970]
                    tunnel: w3962 -> [_ w3971]
                    tunnel: w3960 -> [w3963 w3964]
                    tunnel: [w3963 w3964] -> w3959
                    frame False {
                    }
                    frame True {
                      n2065 = local write "Moving 1"(w3970) -> ()
                      n2066 = property class="Ctl"(reference=w3971) -> (reference out=w3965:refnum<vi>, "Position"=w3969:T11)  [unwired: 1 in, 1 out]
                      n2067 = Divide(x=w3969, y=T40 {"Width"=2, "Height"=2}) -> (x/y=w3967:cluster{dbl, dbl})
                      n2068 = Subtract(x=w3964, y=w3967) -> (x-y=w3966:cluster{dbl, dbl})
                      n2069 = property on="Property Node" class="Ctl"(reference=w3965, "Position"=w3966) -> ()  [unwired: 1 in, 2 out]
                    }
                  }
                }
              }
            }
          }
          frame True {
            n2070 = local read "TC1to45PicRef"() -> (w3973:refnum<vi>)
            n2071 = case shown="True" w3974 {
              selector: w3974 -> [_ w3982]
              tunnel: w3973 -> [_ w3981]
              tunnel: w3972 -> [_ w3976]
              frame False {
              }
              frame True {
                # "Place control where the mouse is."
                n2072 = local write "Moving 1"(w3982) -> ()
                n2073 = property class="Ctl"(reference=w3981) -> (reference out=w3977:refnum<vi>, "Bounds"=w3979:T40)  [unwired: 1 in, 1 out]
                n2074 = Divide(x=w3979, y=T40 {"Width"=2, "Height"=2}) -> (x/y=w3975:cluster{"Width":dbl, "Height":dbl})
                n2075 = Subtract(x=w3976, y=w3975) -> (x-y=w3978:cluster{dbl, dbl})
                n2076 = property on="Property Node" class="Ctl"(reference=w3977, "Position"=w3978) -> ()  [unwired: 1 in, 2 out]
              }
            }
          }
        }
      }
      event "TC1to75visual": Mouse Up {
        # "This case is needed to unlock cursor from the Boolean."
        n2077 = event-data() -> ()  [unwired: 1 in, 1 out]
        n2078 = local write "Moving 1"(FALSE ("Moving 1")) -> ()
      }
      event "TC1to75visual": Mouse Down {
        # "Begin moving Boolean with cursor when the mouse button is pressed."
        n2079 = event-data() -> ()  [unwired: 1 in, 1 out]
      }
      event "Reset All TC Positions": Mouse Down {
        n2080 = event-data() -> ()  [unwired: 1 in, 1 out]
        n2081 = control-ref of="TC1to75visual"() -> (w3988:refnum<vi>)
        n2082 = property class="Clust (strict)"(reference=w3988) -> ("Controls[]"=w3987:refnum<vi>[])  [unwired: 1 in, 2 out]
        n2083 = for {
          N: 75 -> [_]
          tunnel: w3987 -> [w3991] mode=indexing
          tunnel: w3986 -> [w3990] mode=indexing
          n2084 = property class="Ctl"(reference=w3991, "Position"=w3990) -> ()  [unwired: 1 in, 2 out]
        }
      }
    }
    n2085 = local read "exit"() -> (w3932:bool)
  }
  n2086 = case shown="True" FALSE {
    frame False {
    }
    frame True {
      n2087 = control-ref of="TC1to75visual"() -> (w3996:refnum<vi>)
      n2088 = property class="Clust (strict)"(reference=w3996) -> ("Controls[]"=w3995:refnum<vi>[])  [unwired: 1 in, 2 out]
      n2089 = Initialize Array(T11 {"Left"=0, "Top"=0} ("Position"), 75 ("dimension size")) -> (w3992:T11[])
      n2090 = for {
        N: 75 -> [_]
        tunnel: w3995 -> [w4002] mode=indexing
        shift-right: [w4000] -> _
        shift-left: w3992 -> [w4001]
        i -> [w3998]
        # "Delete at End"
        n2091 = property class="Ctl"(reference=w4002) -> ("Position"=w3999:T11)  [unwired: 1 in, 2 out]
        n2092 = Replace Array Subset(array=w4001, new element=w3999, index=w3998) -> (w4000:T11[])
      }
    }
  }
  n2093 = call "Flush Module Queue.vi"("error in (no error)"=w13) -> ("error out"=w12:errorcluster, "flushed msgs"=→"flushed msgs":T10)  [unwired: 9 in]
  n2094 = call "Unload Module.vi"("error in (no error)"=w12) -> ()  [unwired: 10 in, 1 out]
  n2095 = property on="Waveform Chart" class="WFChart (strict)" props=["Plot", "Visible?"]() -> ()  [unwired: 2 in, 3 out]
